vi "AlliGator Settings Storage.vi"(6 "Get(F)/Set":bool, 7 "AlliGator Settings List":T1=enum."Source Image:Use Image Histogram for Contrast", 8 "Error In":errorcluster, 11 "Variant Data in":variant) -> (0 "Error Out":errorcluster, 3 "Variant Data out":variant)   [LabVIEW 2021, in "AlliGator Settings.lvlib"]
doc: "Get/Set Settings parameter values using variant attributes."
uses:
  AlliGator Settings.lvlib
  Phasor/Phasor Explorer Gate Parameters.ctl
  Phasor/Phasor Gate Type.ctl
  Phasor/Phasor Type of User-defined Function.ctl
  Phasor/Phasor Explorer Decay Parameters.ctl
  Phasor/Phasor IRF Model.ctl
  Phasor/Phasor Explorer Phasor Parameters.ctl
  Phasor/Phasor Calculation Type.ctl
  Phasor/Phasor SEPL Type.ctl
  Phasor/Phasor Explorer Display Parameters.ctl
  Phasor/Phasor Type of Series.ctl
  Image/Image Save File Format.ctl
  AlliGator Phasor Plot Size.ctl
  AlliGator Gates to Skip.ctl
  Graphs/XY Graph/XY Graph Plot Shift Parameters.ctl
  Graphs/XY Graph/XY Graph Plot Shift Method.ctl
  Fits/IRF(X)PSED/IRF(X)PSED Extraction Options.ctl
  Fits/IRF(X)PSED/Fourier Series Smoothing Option.ctl
  Fits/IRF(X)PSED/Fourier Series Truncation.ctl
  Fits/IRF(X)PSED/IRF Extraction Method.ctl
  AlliGator Settings List.ctl
  AlliGator Low Count Pixels Rejection Options.ctl
  Phasor/Phasor Ratio Type.ctl
  AlliGator Baseline Subtraction Method.ctl
  Fits/IRF(X)PSED/Decay Fit Options v2.ctl
  Fits/Decay Convolution/Decay Model.ctl
  Fits/Residual Type.ctl
  Fits/IRF(X)PSED/Fit Weights Type.ctl
  Fits/Non-linear Fitting Method v2.ctl
  Fits/Fit Calculation Method.ctl
  Fits/Non-linear Fitting Algorithm.ctl
  Fits/IRF(X)PSED/Decay Fit Parameters & Derived Quantities List.ctl
  AlliGator Decay Fit Parameter Constraints 2.ctl
  Fits/IRF(X)PSED/Decay Fit Parameters In List.ctl
  AlliGator IRF Optimization Controls.ctl
  AlliGator IRF Deconvolution Metrics.ctl
  Math/Advanced Signal Processing Toolkit/Wavelet Analysis Options.ctl
  AlliGator High Count Pixels Rejection Options.ctl
  AlliGator Image Smoothing Options.ctl
  Arrays/Kernel Type.ctl
  Arrays/Smoothing Algorithm.ctl
  Fits/Square Pulse/Square Pulse Options.ctl
  Fits/Square Pulse/Square Pulse Levels Type.ctl
  AlliGator Image Binning Options.ctl
  AlliGator Phasor Plot Smoothing Options.ctl
  AlliGator Phasor Plot Graphics Options.ctl
  AlliGator Exported Image Settings.ctl
  AlliGator Define Gates to.ctl
  AlliGator Gates to Keep.ctl
  AlliGator Phasor Ratio Color-Coded Quantity.ctl
  Phasor/Phasor Calibration Type.ctl
  Histograms/Linear Histogram Options.ctl
  Histograms/Histogram Bin Option.ctl
  Histograms/Histogram Bin Position.ctl
  AlliGator Gate Arithmetic.ctl
  AlliGator Phasor Reference Associated with Shortest Lifetime.ctl
  AlliGator Python Settings.ctl
  SwissSPAD/SwissSPAD Live_Image Display Options.ctl
  AlliGator Average Lifetime Options.ctl
  AlliGator Calibration Map Algorithm.ctl
  AlliGator Guess Parameters Options.ctl
  Phasor/Phasor Standard Deviation Options.ctl
  AlliGator Source Image Scale Bar Options.ctl
  Fits/IRF(X)PSED/MLE Baseline Offset Type.ctl
  Image/Flatfield Correction Options.ctl
  Graphs/XY Graph/XY Plot Data.ctl
  Phasor/Phasor User-defined Gate & IRF.vi
  Notebook/Verbose Mode.vi
  Notebook/Notebook.lvlib
  Graphs/XY Graph/XY Graph Add-Ons.lvlib
  Phasor/Phasor.lvlib
  Utilities/Utilities.lvlib
  AlliGator Decay Analysis.lvlib
  AlliGator Phasor Plot.lvlib
  Image/Image.lvlib
  AlliGator Decay Preprocessing.lvlib
  Fits/Fits.lvlib
  AlliGator Decay Fit.lvlib
  AlliGator IRF.lvlib
  Math/Math.lvlib
  Arrays/Arrays.lvlib
  AlliGator Source Image.lvlib
  Phasor/Phasor Explorer.lvlib
  AlliGator Phasor Ratio.lvlib
  Histograms/Histogram Window.lvlib
  SwissSPAD/SwissSPAD Live.lvlib
  AlliGator Phasor Calibration.lvlib
panel:
  in  "Show Dead Left Columns Correction":bool
  in  "Tab Control":T2(tab)
  in  "Source ImageTab":T3(tab)
  in  "Use Image Histogram for Contrast":bool=TRUE
  in  "Low Count Pixels Rejection Options":T4={"Background Low Threshold Factor"=0.0, "Fixed Low Background Threshold"=20000.0, "Reject Low Count Pixels"=FALSE, "Low Percentile"=0.0} {"Low Percentile" min=0.0 max=100.0}
  in  "High Count Pixels Rejection Options":T5={"Background High Threshold Factor"=0.0, "Fixed High Background Threshold"=20000.0, "Reject High Count Pixels"=FALSE, "High Percentile"=100.0} {"High Percentile" min=0.0 max=100.0}
  in  "Hot Pixel Removal":T6 {"Percentile" min=0 max=100}
  in  "Dead Left Columns Correction":bool
  in  "Use Fixed ROI Diameter":bool
  in  "ROI Diameter":i32=12
  in  "ROI Center Color":u32(colorbox)=16711680
  in  "Image Binning Options":T7={"Use Image Binning"=FALSE, "X Bin"=1, "Y Bin"=1} {"Y Bin" min=1; "X Bin" min=1}
  in  "Flatfield Correction":T8={"Flatfield Estimation Options"={"Sampling Grid Size X"=256, "Sampling Grid Size Y"=256, "Polynomial Degree"=5}, "Background Options"={"Estimate Background"=TRUE, "Background Estimation Size"=32, "Niblack Deviation Factor [0. 1]"=0.2}, "Correction Factor"=1.1} {"Background Options"."Niblack Deviation Factor [0. 1]" min=0.0 max=1.0}
  in  "Image Smoothing Options":T9={"Use Image Smoothing"=FALSE, "Kernel Type"=enum."Bilinear", "Bin"=500, "Algorithm"=enum."Rapid"} {"Bin" min=1}
  in  "Peak Threshold":dbl=500.0
  in  "Intensity Threshold":dbl=500.0
  in  "Invert Binary Mask":bool
  in  "Image Pre-Processing Operations Order":string[](array[string]) caption="Order"
  in  "Median Overlay Color":u32(colorbox)
  in  "Overlay ROI Median":bool=TRUE caption="Use Image Brightness"
  in  "Image Resolution (Pixel Size)":dbl[unit]
  in  "Scale Bar Options":T12 caption="Scale Bar Options (*)"
  in  "Overlay Analyzed ROI Center":bool
  in  "Use Image Brightness":bool=TRUE
  in  "Blend Overlay with Image Background":bool=TRUE
  in  "Dataset Scaling Factor":dbl=1.0 caption="Scaling Factor" min=0.0
  in  "Gate Image Integration":dbl[unit]=3e-10 min=0.0 format="%#.3g"
  in  "Gate Image Exposure":dbl[unit]=3e-10 min=0.0 format="%#.3g"
  in  "Background File Subtraction":bool
  in  "Background Scaling Factor":dbl=1.0 caption="Scaling Factor"
  in  "Background File":path
  in  "Background Pile-up Correction":bool caption="Pile-up Correction"
  in  "Background Pixel Well Capacity":u32=1 caption="Max Value" min=1 step=1
  in  "Channel Arithmetic":T13
  in  "Available Gate Names":string[](array[string])
  in  "Channel Name":u16(ring) items=["Gate"]
  in  "Gates to Keep":T14 caption="Gates to Keep (*)"
  in  "Define Gates to":T15
  in  "Laser Period":dbl[unit] format="%#_3g"
  in  "Gates to Skip":T16
  in  "Gate Separation":dbl[unit]=4e-11
  in  "Gate Width":dbl[unit]=3e-10
  in  "Gate Step":i32=1 min=1
  in  "Pile-up Correction":bool
  in  "Pixel Well Capacity":i32=1 min=1
  in  "# Gates":u32=1 min=1 step=1
  in  "SYNC Period":dbl[unit] caption="IRF Period" min=0.0 format="%#_3g"
  in  "Mscrotime Gate Separation":dbl[unit]=1.0 min=0.0
  in  "Decay Tabs":T17(tab)
  in  "# Folds":u32=1 min=1
  in  "Fold Decay":bool caption="Straighten Decay"
  in  "Use Decay Pre-Processing":bool=TRUE
  in  "Head Fraction":dbl min=0.0 max=1.0
  in  "Use Cursors":bool
  in  "Use Periodicity":bool
  in  "Pixel-Normalize Decay":bool
  in  "Verbose Decay Pre-Processing":bool=TRUE caption="Verbose Devay Pre-Processing"
  in  "Straighten Decay":bool
  in  "Reverse Gates":bool caption="Revert Gates"
  in  "Additional Points":u32 caption="Gate Duration"
  in  "Tail Fraction":dbl caption="Gate Duration" min=0.0 max=1.0
  in  "Extrapolate Decay":bool
  in  "Baseline Subtraction Method":T18=enum."Min" caption="Method"
  in  "Background Definition Range":T19={"Min Gate"=0.0, "Max Gate"=8e-10}
  in  "Decay Shift Parameters":T20
  in  "Shift Decay":bool
  in  "Smoothen Decay":bool caption="Smooth Decay"
  in  "Smoothing Parameter":dbl caption="Gate Duration" min=0.0 max=1.0
  in  "1-Normalize Decay":bool
  in  "Background Subtraction":bool=TRUE
  in  "Constant Background":dbl=1.0
  in  "Decay Pre-Processing Operations Order":string[](array[string]) caption="Order"
  in  "[0-1]-Normalize Decay":bool caption="1- Normalize Decay"
  in  "Average Lifetime Options":T22={"Use Local IRF "=TRUE, "Use IRF Offset"=TRUE, "Use Fixed Offset"=TRUE, "Fixed Offset"=0.0, "Baseline %"=0.0} caption="Use Local IRF" {"Baseline %" min=0.0 max=100.0}
  in  "IRF Time Constants":dbl[](array[numeric])
  in  "IRF order":i32
  in  "Square Pulse Options":T23={"Method"=enum."Mode", "# Bins"=0, "Threshold %"=10.0, "Center on Midpoint"=FALSE, "Smoothen Plot"=FALSE} {"Threshold %" min=0.0 max=100.0}
  in  "Wavelet Analysis Options":T25={"Wavelet"=enum."db02", "Option for Approximate Coefficients"=enum."None", "# Levels"=1, "Threshold Settings"={"Thresholding Rule"=enum."Universal", "Rescaling Method"=enum."Single level", "Soft Threshold?"=TRUE}, "Wavelet Transform Type"=enum."Discrete"}
  in  "Time Constant for IRF Extraction":T26={"Time Constant for IRF Extraction"=1e-18, "IRF Order"=1, "Fourier Series Smoothing"=enum."None", "Noise Threshold"=0.0, "Smoothing Width"=0.0, "Fourier Series Truncation"=enum."Automatic", "Truncation Order"=0, "Save Power Spectrum"=FALSE, "Smoothing"=FALSE, "Smoothing Parameter"=0.0, "Smoothing Order"=1, "Method"=enum."Direct"} caption="Gate Duration" {"Smoothing Order" min=1 max=10; "Time Constant for IRF Extraction" format="%#_5g"}
  in  "Extract IRF instead of Decay":bool
  in  "IRF Optimization Options":T30={"Search Range"=1e-18, "Search Step"=1e-09, "Tail Threshold (%)"=1e-09, "Regularized IRF"=FALSE, "Export Plot"=FALSE, "Export Data"=FALSE, "Smooth Metrics"=FALSE, "S-G Side Points"=1, "S-G Polynomial Order"=3, "Metrics"=enum."Average"} {"S-G Polynomial Order" min=3 max=10; "S-G Side Points" min=1; "Search Range" min=0.0 max=1e-09}
  in  "Use Data Information Laser Period":bool
  in  "Use Legagy Fitting Approach":bool
  in  "Fit Options":T32={"Show Fit Residuals"=TRUE, "Fit Model"=enum."1-Exponential", "Residual Type"=enum."Standard", "Max Decay Percentile"=0.0, "Min Decay Percentile"=0.0, "Show Full Decay"=TRUE, "Weights"=enum."Unweighted", "Fitting Method"=enum."Least Square", "Compute Parameter Uncertainties"=TRUE, "Periodic Boundaries"=TRUE, "Model Calculation"=enum."Simulation", "Period"=1.2500000000000001e-08, "Termination Criteria"={"Max Iterations"=1000, "Max Function Calls"=0, "Max Time"=1000.0, "Function Tolerance"=1e-06, "Parameter Tolerance"=1e-06, "Gradient Tolerance"=0.0, "Min Lambda"=1e-06, "Max Lambda"=1e-06, "Initial Tick Count"=0}, "Offset Resolution"=1.2500000000000001e-08, "Use Local IRF"=TRUE, "Fitting Algorithm"=enum."Levenberg-Marquardt"} {"Offset Resolution" min=0.0; "Period" min=0.0; "Min Decay Percentile" min=0.0 max=1.0; "Max Decay Percentile" min=0.0 max=1.0}
  in  "MLE Baseline Offset Type":T39
  in  "MLE Baseline Offset":dbl
  in  "Guess Parameters Options":T40 caption="Options"
  in  "Guess Parameters Names":T41[](array[typedef])
  in  "Guess Parameter Values":dbl[](array[numeric]) caption="Guess Parameters"
  in  "Fit Parameter Constraints":T42[](array[typedef]) {"Max Value" format="%#.3g"; "Min Value" format="%#.3g"}
  in  "Displayed Fit Parameters":T43[](array[typedef])
  in  "Export Tabulated Results":bool=TRUE
  in  "Decay Graph Color Array":u32[](array[colorbox])
  in  "Show Last Decay only":bool
  in  "Max Peak Value":dbl
  in  "Reject High Decay Peak Pixels":bool
  in  "Min Peak Value":dbl
  in  "Reject Low Decay Peak Pixels":bool
  in  "Intensity Correction File":path
  in  "Use Intensity Correction File":bool
  in  "Use File Timestamp":bool
  in  "Time Step":dbl[unit]=1.0
  in  "User-defined Quantity":string
  in  "Blend Overlay with Phasor Background":bool=TRUE
  in  "Draw Reference Segment":bool
  in  "Store Phasor Harmonics":bool
  in  "All Phasor Plot ROIs":bool
  in  "Selected Phasor Plot ROI(s)":bool
  in  "Phasor Ratio Color-Coded Quantity":T44 caption="Displayed Quantity"
  in  "All Image ROIs":bool
  in  "Selected Image ROI(s)":bool
  in  "Reference Radius":i32=512
  in  "Phasor Ratio Display Range":cluster{dbl, dbl}(slide)={0.0, 454.0} scale=0.0..1.0
  in  "Phasor Plot Graphics Options":T45={"UC Color"=3381759, "Show UC Tau Ticks"=FALSE, "SEPL Color"=3381759, "Show SEPL Tau Ticks"=FALSE, "Axes Color"=16776960, "Show (g,s) Ticks"=FALSE, "Show UC"=FALSE, "Show SEPL"=FALSE, "Show Axes"=FALSE, "Show UC Tau Labels"=FALSE, "Show SEPL Tau Labels"=FALSE, "Show (g,s) Labels"=FALSE, "UC Label Size"=18, "UC Label Distance"=0.0, "SEPL Label Size"=18, "SEPL Label Distance"=0.0, "Axes Label Size"=18, "Axes Label Distance"=0.0}
  in  "Phasor Plot Smoothing Options":T46={"Use Phasor Plot Smoothing"=FALSE, "Kernel Type"=enum."Uniform", "Bin"=1, "Algorithm"=enum."Rapid"} {"Bin" min=1 step=2}
  in  "Phasor Ratio Color Map":string
  in  "Phasor Ratio Color Map Type":T47(radio)
  in  "Show Color Map Vertices":bool=TRUE
  in  "Exponential Fading":bool
  in  "Phasor Ratio Reference Colors":T48={"Reference 1"=3381759, "Reference 2"=3381759, "Boundary"=3381759}
  in  "Phasor Ratio Decay Range":dbl=1.0
  in  "Show References":bool
  in  "Save Phasor Plot":bool
  in  "Cumulative Phasor Plot":bool
  in  "Phasor Plot Size":T49={"H"=512, "V"=512, "Margin"=0.2} {"Margin" min=0.0}
  in  "Use Phasor Brightness":bool
  in  "Phasor SDV Options":T50={"Compute Estimated SDV"=FALSE, "# Replicas"=100, "Use Estimated Average Phasor"=FALSE}
  in  "Define Shortest Lifetime as":T51
  in  "Save Phasor Graph Image":bool
  in  "Pixel-level Phasor Computation":bool
  in  "Phasor Ratio Type":T52
  in  "Phasor Frequency":dbl[unit]=160000000.0
  in  "Phasor Graph Active":bool caption="Save Phasor Graph Image"
  in  "SEPL Tabs":enum32{"Display", "Phasor", "IRF", "Gates"}(tab)
  in  "SEPL Display Parameters":T53={"# Points"=1000, "Ramp Type"=enum."Logarithmic", "Type of Series"=enum."1-Exp Decays", "Min tau"=1.0000000000000002e-12, "Max tau"=1.0000000000000001e-07, "Include 0"=FALSE, "Include Infinity"=FALSE} {"Min tau" min=0.0; "Max tau" min=0.0; "# Points" min=1 step=1}
  in  "SEPL Phasor Parameters":T55={"Harmonic Frequency"=0.0, "Use f* = 1/D Frequency"=FALSE, "Calibrated Phasor"=FALSE, "Calibration Lifetime"=1e-09, "Phasor Calculation"=enum."Direct Sum", "SEPL Type"=enum."UC", "# Gates"=1.0, "Square Gate Width"=1e-09, "Show Ticks"=FALSE} {"Square Gate Width" min=0.0; "# Gates" min=0.0; "Calibration Lifetime" min=0.0; "Harmonic Frequency" min=0.0}
  in  "SEPL IRF Parameters":T58={"Lifetime"=3.0000000000000004e-09, "IRF Offset"=0.0, "IRF Period"=1.2500000000000001e-08, "Normalized Decays"=FALSE, "IRF Model"=enum."Dirac", "IRF Parameter 1"=0.0} {"Lifetime" min=0.0; "IRF Period" min=0.0}
  in  "SEPL Gate Parameters":T60={"First Gate Start"=0.0, "Use Gate Center"=FALSE, "Gate Width"=0.0, "Gate Step"=0.0, "# Gates"=1.0, "Gate Type"=enum."Square", "Edge Width"=0.0, "Top Slope"=0.0, "Reversed Sawtooth?"=FALSE, "Analytical Computation"=FALSE, "Integration"=enum."Item 0", "Tolerance"=1.0, "# Steps"=1.0, "Type of User-defined Function"=enum."Gate", "Use Gate Step"=FALSE} {"# Steps" min=0.0; "Tolerance" min=0.0; "Top Slope" min=0.0; "Edge Width" min=0.0; "Gate Step" min=0.0; "# Gates" min=1.0 step=1.0; "Gate Width" min=0.0}
  in  "Calibration Map Algorithm":T63
  in  "Calibration Type":T64=enum."Single Phasor"
  in  "Use Backup Calibration if needed":bool=TRUE
  in  "Backup Calibration Type":T65(ring) caption="Backup Calibration"
  in  "Calibration Lifetime":dbl[unit]=1e-09
  in  "Decay Analysis Parameters":T20
  in  "Python Settings":T66
  in  "Transparent Mask Color":u32(colorbox)
  in  "ROI Description Max Characters":i32=256
  in  "Beep on Error":bool caption="Verbose Error Mode"
  in  "# Logical Processors Used":i32 caption="Used" min=1 max=16
  in  "Histogram Options":T67={"Bin Size"=0.0, "Bin Number"=0, "Bin Option"=enum."Bin Number", "Min Value"=-inf, "Max Value"=inf, "Filter NaN & Infinite Values"=TRUE, "Frequency Plot"=FALSE, "Align Bins"=FALSE, "Bin Location"=enum."Left", "Project Outside Values"=FALSE, "Max Histogram Size"=100000} {"Max Histogram Size" format="%.0e"}
  in  "Exported Gate Image Settings":T70
  in  "Verbose Error Mode":bool
  in  "Verbose Settings Mode":bool
  in  "Beep after Script":bool
  in  "Verbose Mode":bool
  in  "Saved Displayed Image File Format":T71
  in  "Visible Settings Tab":string caption="Settings Tab List"
  in  "Include Loading in Timing":bool
  in  "Last Run Version":string
  # "see the AlliGator License on the block diagram (Ctrl+E or Window:Show Block Diagram)"
  # "Gates Characteristics"
  # "Limit Phasor Plot Analysis  to:"
  # "Lifetime Analysis Options"
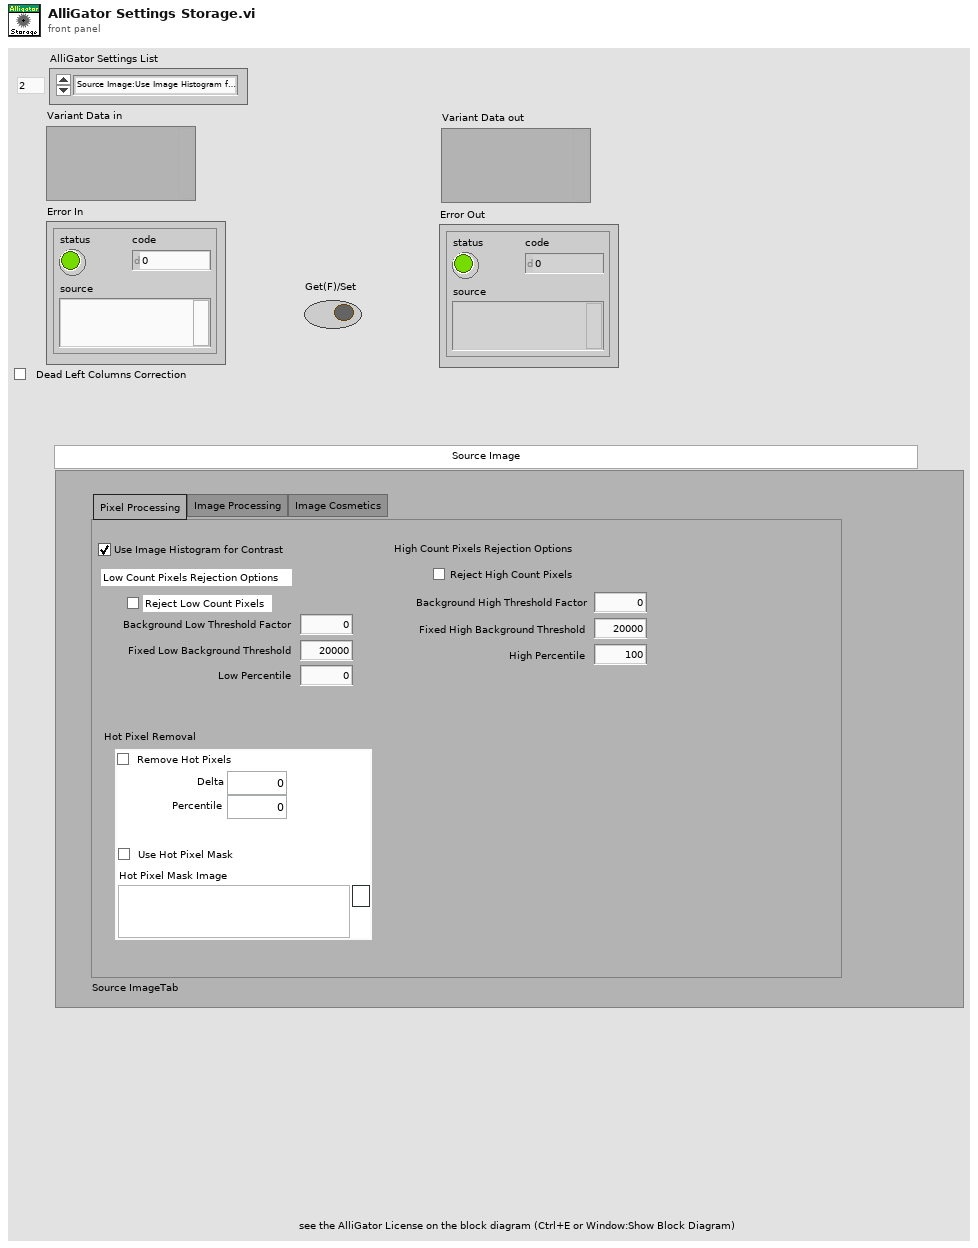
[diagram p1: front panel]
types:
  T1 = typedef "AlliGator Settings.lvlib/AlliGator Settings List.ctl" = enum16{"GUI:Visible Settings Tab", "GUI:Last Run Version", "Source Image:Use Image Histogram for Contrast", "Source Image:Low Count Pixels Rejection Options", "Source Image:High Count Pixels Rejection Options", "Source Image:Use Image Brightness", "Source Image:Blend Overlay with Image Background", "Source Image:Use Fixed ROI Diameter", "Source Image:ROI Diameter", "Source Image:ROI Center Color", "Source Image:Peak Threshold", "Source Image:Intensity Threshold", "Source Image:Image Binning Options", "Source Image:Image Smoothing Options", "Source Image:Image Histogram Active", "Source Image:Invert Binary Mask", "Source Image:Hot Pixel Removal", "Source Image:Overlay Analyzed ROI Center", "Source Image:Auto-Adjust Contrast", "Source Image:Histogram Lower Percentile", "Source Image:Histogram Upper Percentile", "Source Image:Save Source Image", "Source Image:Scale Bar Options", "Source Image:Image Resolution (Pixel Size)", "Source Image:Flatfield Correction", "Source Image:Show Dead Left Columns Correction", "Source Image:Dead Left Columns Correction", "Source Image:Image Pre-Processing Operations Order", "Source Image:Overlay ROI Median", "Source Image:Median Overlay Color", "Data Information:Gate Width", "Data Information:Nanotime Gate Separation", "Data Information:Macrotime Gate Separation", "Data Information:Gate Step", "Data Information:# Gates", "Data Information:Gate Image Exposure", "Data Information:Gate Image Integration", "Data Information:Gates to Skip", "Data Information:Gates to Keep", "Data Information:Define Gates to", "Data Information:Channel Name", "Data Information:Available Channel Names", "Data Information:Channel Arithmetic", "Data Information:Background File Subtraction", "Data Information:Background File", "Data Information:Background Scaling Factor", "Data Information:Background Pile-up Correction", "Data Information:Background Pixel Well Capacity", "Data Information:Laser Period", "Data Information:SYNC Period", "Data Information:Pile-up Correction", "Data Information:Pixel Well Capacity", "Data Information:Dataset Scaling Factor", "Fluorescence Decay_Decay Pre-Processing:Reverse Gates", "Fluorescence Decay_Decay Pre-Processing:Verbose Decay Pre-Processing", "Fluorescence Decay_Decay Pre-Processing:Use Decay Pre-Processing", "Fluorescence Decay_Decay Pre-Processing:Background Subtraction", "Fluorescence Decay_Decay Pre-Processing:Background Definition Range", "Fluorescence Decay_Decay Pre-Processing:Baseline Subtraction Method", "Fluorescence Decay_Decay Pre-Processing:Decay Pre-Processing Operations Order", "Fluorescence Decay_Decay Pre-Processing:Smoothing Parameter", "Fluorescence Decay_Decay Pre-Processing:Shift Decay", "Fluorescence Decay_Decay Pre-Processing:Decay Shift Parameters", "Fluorescence Decay_Decay Pre-Processing:Fold Decay", "Fluorescence Decay_Decay Pre-Processing:# Folds", "Fluorescence Decay_Decay Pre-Processing:1-Normalize Decay", "Fluorescence Decay_Decay Pre-Processing:[0-1]-Normalize Decay", "Fluorescence Decay_Decay Pre-Processing:Smoothen Decay", "Fluorescence Decay_Decay Pre-Processing:Extrapolate Decay", "Fluorescence Decay_Decay Pre-Processing:Use Periodicity", "Fluorescence Decay_Decay Pre-Processing:Use Cursors", "Fluorescence Decay_Decay Pre-Processing:Tail Fraction", "Fluorescence Decay_Decay Pre-Processing:Head Fraction", "Fluorescence Decay_Decay Pre-Processing:Additional Points", "Fluorescence Decay_Decay Pre-Processing:Straighten Decay", "Fluorescence Decay_Decay Pre-Processing:Constant Background", "Fluorescence Decay_Decay Pre-Processing:Pixel-Normalize Decay", "Fluorescence Decay_Advanced Analysis:Extract IRF instead of Decay", "Fluorescence Decay_Advanced Analysis:IRF Extraction Options", "Fluorescence Decay_Advanced Analysis:IRF Optimization Options", "Fluorescence Decay_Advanced Analysis:Square Pulse Options", "Fluorescence Decay_Advanced Analysis:IRF Order", "Fluorescence Decay_Advanced Analysis:IRF Time Constants", "Fluorescence Decay_Advanced Analysis:Wavelet Analysis Options", "Fluorescence Decay_Advanced Analysis:Average Lifetime Options", "Fluorescence Decay_Fit Options:Fit Options", "Fluorescence Decay_Fit Options:Use Legacy Fitting Approach", "Fluorescence Decay_Fit Options:Use Data Information Laser Period", "Fluorescence Decay_Fit Parameters:Displayed Fit Parameters", "Fluorescence Decay_Fit Parameters:Fit Parameter Constraints", "Fluorescence Decay_Fit Parameters:Export Tabulated Results", "Fluorescence Decay_Fit Parameters:MLE Baseline Offset Type", "Fluorescence Decay_Fit Parameters:MLE Baseline Offset", "Fluorescence Decay_Fit Parameters:Guess Parameter Names", "Fluorescence Decay_Fit Parameters:Guess Parameter Values", "Fluorescence Decay_Fit Parameters:Guess Parameters Options", "Fluorescence Decay_Styles:Show Last Decay Only", "Fluorescence Decay_Styles:Decay Graph Color Array", "Fluorescence Decay:Decay Graph Active", "Fluorescence Decay Statistics:Min Peak Value", "Fluorescence Decay Statistics:Reject Low Decay Peak Pixels", "Fluorescence Decay Statistics:Reject High Decay Peak Pixels", "Fluorescence Decay Statistics:Max Peak Value", "Time Traces:Use File Timestamp", "Time Traces:Time Step", "Time Traces:Use Intensity Correction File", "Time Traces:Intensity Correction File", "Phasor Plot:Phasor Plot Smoothing Options", "Phasor Plot:Phasor Plot Size", "Phasor Plot:Phasor Plot Graphics Options", "Phasor Plot:Cumulative Phasor Plot", "Phasor Plot:Use Phasor Brightness", "Phasor Plot:Blend Overlay with Phasor Background", "Phasor Plot:Save Phasor Plot", "Phasor Plot:Show References", "Phasor Plot:Phasor Ratio Decay Range", "Phasor Plot:Exponential Fading", "Phasor Plot:Phasor Ratio Reference Colors", "Phasor Plot:Reference Radius", "Phasor Plot:Show Color Map Vertices", "Phasor Plot:Phasor Plot Active", "Phasor Plot:Phasor Ratio Color Map Type", "Phasor Plot:Phasor Ratio Color Map", "Phasor Plot:Phasor Ratio Display Range", "Phasor Plot:Selected Image ROI(s)", "Phasor Plot:All Image ROIs", "Phasor Plot:Selected Phasor Plot ROI(s)", "Phasor Plot:All Phasor Plot ROIs", "Phasor Plot:Phasor Ratio Color-Coded Quantity", "Phasor Plot:Store Phasor Harmonics", "Phasor Plot:Draw Reference Segment", "Phasor Plot:User-Defined Quantity", "Phasor Graph:Phasor Frequency", "Phasor Graph:Phasor Ratio Type", "Phasor Graph:Pixel-level Phasor Computation", "Phasor Graph:Save Phasor Graph", "Phasor Graph:Phasor Graph Active", "Phasor Graph:Phasor SDV Options", "Phasor Calibration:Use Backup Calibration if needed", "Phasor Graph:Define Shortest Lifetime as", "Phasor Calibration:Backup Calibration Type", "Phasor Calibration:Calibration Type", "Phasor Calibration:Calibration Lifetime", "Phasor Calibration:Calibration Map Algorithm", "Single-Exponential Phasor Locus (SEPL):Gate Parameters", "Single-Exponential Phasor Locus (SEPL):User-defined Gate", "Single-Exponential Phasor Locus (SEPL):User-defined IRF", "Single-Exponential Phasor Locus (SEPL):Phasor Parameters", "Single-Exponential Phasor Locus (SEPL):Decay & IRF Parameters", "Single-Exponential Phasor Locus (SEPL):Display Parameters", "Lifetime Analysis:Decay Analysis Parameters", "Lifetime Analysis:Lifetime Map Active", "Plugins:Python Settings", "Miscellaneous:Verbose Mode", "Miscellaneous:Beep after Script", "Miscellaneous:Saved Image File Format", "Miscellaneous:Exported Gate Image Settings", "Miscellaneous:Include Loading in Timing", "Miscellaneous:Verbose Settings Mode", "Miscellaneous:Histogram Options", "Miscellaneous:Beep on Error", "Miscellaneous:# Logical Processors Used", "Miscellaneous:ROI Description Max Characters", "Miscellaneous:Verbose Error Mode", "Miscellaneous:Transparent Mask Color"}
  T2 = enum32{"Source Image", "Data Information", "Fluorescence Decay", "Fluorescence Decay Statistics", "Time Traces", "Phasor Plot", "Phasor Graph", "Single-Exponential Phasor Locus (SEPL)", "Phasor Calibration", "Lifetime Analysis", "Plugins", "Miscellaneous"}
  T3 = enum32{"Pixel Processing", "Image Processing", "Image Cosmetics"}
  T4 = typedef "AlliGator Settings.lvlib/AlliGator Low Count Pixels Rejection Options.ctl" = cluster{"Background Low Threshold Factor":dbl, "Fixed Low Background Threshold":dbl, "Reject Low Count Pixels":bool, "Low Percentile":dbl}
  T5 = typedef "AlliGator Settings.lvlib/AlliGator High Count Pixels Rejection Options.ctl" = cluster{"Background High Threshold Factor":dbl, "Fixed High Background Threshold":dbl, "Reject High Count Pixels":bool, "High Percentile":dbl}
  T6 = typedef "SwissSPAD Live.lvlib/SwissSPAD Live_Image Display Options.ctl" = cluster{"Remove Screamers":bool, "Delta":sgl, "Equalize Histogram":bool, "Percentile":sgl, "Hot Pixel Mask Image":path, "Use Hot Pixel Mask":bool}
  T7 = typedef "AlliGator Source Image.lvlib/AlliGator Image Binning Options.ctl" = cluster{"Use Image Binning":bool, "X Bin":i32, "Y Bin":i32}
  T8 = typedef "Image.lvlib/Flatfield Correction Options.ctl" = cluster{"Flatfield Estimation Options":cluster{"Sampling Grid Size X":i32, "Sampling Grid Size Y":i32, "Polynomial Degree":i32}, "Background Options":cluster{"Estimate Background":bool, "Background Estimation Size":i32, "Niblack Deviation Factor [0. 1]":dbl}, "Correction Factor":sgl}
  T9 = typedef "AlliGator Settings.lvlib/AlliGator Image Smoothing Options.ctl" = cluster{"Use Image Smoothing":bool, "Kernel Type":T10, "Bin":i32, "Algorithm":T11}
  T10 = typedef "Arrays.lvlib/Kernel Type.ctl" = enum16{"Uniform", "Bilinear", "Gaussian"}
  T11 = typedef "Arrays.lvlib/Smoothing Algorithm.ctl" = enum16{"Rapid", "Thorough"}
  T12 = typedef "AlliGator Source Image.lvlib/AlliGator Source Image Scale Bar Options.ctl" = cluster{"Show Scale Bar Overlay":bool, "Scale Bar Length":dbl[unit], "Scale Bar Color":u32, "Scale Bar X":u32, "Scale Bar Y":u32, "Scale Bar Height":dbl[unit]}
  T13 = typedef "AlliGator Settings.lvlib/AlliGator Gate Arithmetic.ctl" = enum16{"None", "INT-G2", "G2/INT*<INT>", "(1 - G2/INT)*<INT>"}
  T14 = typedef "AlliGator Settings.lvlib/AlliGator Gates to Keep.ctl" = cluster{"First":u32, "Last":u32}
  T15 = typedef "AlliGator Settings.lvlib/AlliGator Define Gates to.ctl" = enum32{"Skip", "Keep"}
  T16 = typedef "AlliGator Decay Analysis.lvlib/AlliGator Gates to Skip.ctl" = cluster{"Start":u32, "End":u32}
  T17 = enum32{"Decay Pre-Processing", "Advanced Analysis", "Fit Options", "Fit Parameters", "Styles"}
  T18 = typedef "AlliGator Decay Analysis.lvlib/AlliGator Decay Preprocessing.lvlib/AlliGator Baseline Subtraction Method.ctl" = enum16{"Mean", "Min", "Square Gated Single-Exponential", "File", "Constant"}
  T19 = cluster{"Min Gate":dbl[unit], "Max Gate":dbl[unit]}
  T20 = typedef "XY Graph Add-Ons.lvlib/XY Graph Plot Shift Parameters.ctl" = cluster{"Type":T21, "Shift":dbl[unit], "Threshold":dbl, "Rotate":bool}
  T21 = typedef "XY Graph Add-Ons.lvlib/XY Graph Plot Shift Method.ctl" = enum16{"Default", "CFD", "Threshold", "Cross-Correlation"}
  T22 = typedef "AlliGator Settings.lvlib/AlliGator Average Lifetime Options.ctl" = cluster{"Use Local IRF ":bool, "Use IRF Offset":bool, "Use Fixed Offset":bool, "Fixed Offset":dbl[unit], "Baseline %":dbl}
  T23 = typedef "Fits.lvlib/Square Pulse Options.ctl" = cluster{"Method":T24, "# Bins":i32, "Threshold %":dbl, "Center on Midpoint":bool, "Smoothen Plot":bool}
  T24 = typedef "Fits.lvlib/Square Pulse Levels Type.ctl" = enum16{"Mode", "Mean"}
  T25 = typedef "Math.lvlib/Wavelet Analysis Options.ctl" = cluster{"Wavelet":enum16{"db02", "db03", "db04", "db05", "db06", "db07", "db08", "db09", "db10", "db11", "db12", "db13", "db14", "Haar", "bior1_3", "bior1_5", "bior2_2", "bior2_4", "bior2_6", "bior2_8", "bior3_1", "bior3_3", "bior3_5", "bior3_7", "bior3_9", "bior4_4 (FBI)", "bior5_5", "bior6_8", "coif1", "coif2", "coif3", "coif4", "coif5", "sym2", "sym3", "sym4", "sym5", "sym6", "sym7", "sym8"}, "Option for Approximate Coefficients":enum16{"None", "Threshold", "Detrend"}, "# Levels":i32, "Threshold Settings":cluster{"Thresholding Rule":enum16{"SURE", "Hybrid", "Universal", "Minimax"}, "Rescaling Method":enum16{"One", "Single level", "Multiple levels"}, "Soft Threshold?":bool}, "Wavelet Transform Type":enum16{"Discrete", "Undecimated"}}
  T26 = typedef "Fits.lvlib/IRF(X)PSED Extraction Options.ctl" = cluster{"Time Constant for IRF Extraction":dbl[unit], "IRF Order":i32, "Fourier Series Smoothing":T27, "Noise Threshold":dbl, "Smoothing Width":dbl, "Fourier Series Truncation":T28, "Truncation Order":i32, "Save Power Spectrum":bool, "Smoothing":bool, "Smoothing Parameter":dbl, "Smoothing Order":u32, "Method":T29}
  T27 = typedef "Fits.lvlib/Fourier Series Smoothing Option.ctl" = enum16{"None", "Lanczos Factors", "Fejer Summation"}
  T28 = typedef "Fits.lvlib/Fourier Series Truncation.ctl" = enum16{"Automatic", "Fixed"}
  T29 = typedef "Fits.lvlib/IRF Extraction Method.ctl" = enum16{"Direct", "Topless", "Toeplitz"}
  T30 = typedef "AlliGator Decay Analysis.lvlib/AlliGator IRF.lvlib/AlliGator IRF Optimization Controls.ctl" = cluster{"Search Range":dbl[unit], "Search Step":dbl[unit], "Tail Threshold (%)":dbl, "Regularized IRF":bool, "Export Plot":bool, "Export Data":bool, "Smooth Metrics":bool, "S-G Side Points":i32, "S-G Polynomial Order":i32, "Metrics":T31}
  T31 = typedef "AlliGator Decay Analysis.lvlib/AlliGator IRF.lvlib/AlliGator IRF Deconvolution Metrics.ctl" = enum16{"Average", "SDV", "Max", "Average * SDV", "Slope"}
  T32 = typedef "Fits.lvlib/Decay Fit Options v2.ctl" = cluster{"Show Fit Residuals":bool, "Fit Model":T33, "Residual Type":T34, "Max Decay Percentile":dbl, "Min Decay Percentile":dbl, "Show Full Decay":bool, "Weights":T35, "Fitting Method":T36, "Compute Parameter Uncertainties":bool, "Periodic Boundaries":bool, "Model Calculation":T37, "Period":dbl[unit], "Termination Criteria":cluster{"Max Iterations":i32, "Max Function Calls":i32, "Max Time":dbl[unit], "Function Tolerance":dbl, "Parameter Tolerance":dbl, "Gradient Tolerance":dbl, "Min Lambda":dbl, "Max Lambda":dbl, "Initial Tick Count":u32}, "Offset Resolution":dbl[unit], "Use Local IRF":bool, "Fitting Algorithm":T38}
  T33 = typedef "Fits.lvlib/Decay Model.ctl" = enum16{"1-Exponential", "2-Exponentials"}
  T34 = typedef "Fits.lvlib/Residual Type.ctl" = enum16{"Standard", "Normalized", "Reduced"}
  T35 = typedef "Fits.lvlib/Fit Weights Type.ctl" = enum16{"Unweighted", "1/Variance", "Best of All"}
  T36 = typedef "Fits.lvlib/Non-linear Fitting Method v2.ctl" = enum16{"Least Square", "Least Absolute Residual", "Bisquare", "MLE", "-", "Best of All"}
  T37 = typedef "Fits.lvlib/Fit Calculation Method.ctl" = enum16{"Simulation", "Convolution", "Integration"}
  T38 = typedef "Fits.lvlib/Non-linear Fitting Algorithm.ctl" = enum16{"Levenberg-Marquardt", "Trust-Region Dogleg"}
  T39 = typedef "Fits.lvlib/MLE Baseline Offset Type.ctl" = enum32{"Absolute", "Percentage"}
  T40 = typedef "AlliGator Decay Analysis.lvlib/AlliGator Decay Fit.lvlib/AlliGator Guess Parameters Options.ctl" = enum16{"Numerically estimated", "User-provided", "User-provided (normalized)", "Last valid fitted parameters"}
  T41 = typedef "Fits.lvlib/Decay Fit Parameters In List.ctl" = enum16{"Offset", "Baseline", "A_1", "tau_1", "A_2", "tau_2"}
  T42 = typedef "AlliGator Decay Analysis.lvlib/AlliGator Decay Fit.lvlib/AlliGator Decay Fit Parameter Constraints 2.ctl" = cluster{"Fit Parameter":T41, "Min Value":dbl, "Max Value":dbl, "Global":bool, "Used":bool}
  T43 = typedef "Fits.lvlib/Decay Fit Parameters & Derived Quantities List.ctl" = enum16{"Offset", "Baseline", "A_1", "tau_1", "A_2", "tau_2", "<tau>_a", "f1_a", "f2_a", "<tau>_i", "f1_i", "f2_i", "-", "R^2", "Chi^2"}
  T44 = typedef "AlliGator Phasor Ratio.lvlib/AlliGator Phasor Ratio Color-Coded Quantity.ctl" = enum16{"Phasor Ratio (f1 or a1)", "Average Lifetime (<tau>_i or <tau>_a))", "User-Defined Quantity"}
  T45 = typedef "AlliGator Settings.lvlib/AlliGator Phasor Plot Graphics Options.ctl" = cluster{"UC Color":u32, "Show UC Tau Ticks":bool, "SEPL Color":u32, "Show SEPL Tau Ticks":bool, "Axes Color":u32, "Show (g,s) Ticks":bool, "Show UC":bool, "Show SEPL":bool, "Show Axes":bool, "Show UC Tau Labels":bool, "Show SEPL Tau Labels":bool, "Show (g,s) Labels":bool, "UC Label Size":i16, "UC Label Distance":dbl, "SEPL Label Size":i16, "SEPL Label Distance":dbl, "Axes Label Size":i16, "Axes Label Distance":dbl}
  T46 = typedef "AlliGator Phasor Plot.lvlib/AlliGator Phasor Plot Smoothing Options.ctl" = cluster{"Use Phasor Plot Smoothing":bool, "Kernel Type":T10, "Bin":i32, "Algorithm":T11}
  T47 = enum32{"Interpolate Reference Colors", "Use Custom Map"}
  T48 = cluster{"Reference 1":u32, "Reference 2":u32, "Boundary":u32}
  T49 = typedef "AlliGator Phasor Plot.lvlib/AlliGator Phasor Plot Size.ctl" = cluster{"H":i32, "V":i32, "Margin":dbl}
  T50 = typedef "Phasor.lvlib/Phasor Standard Deviation Options.ctl" = cluster{"Compute Estimated SDV":bool, "# Replicas":u32, "Use Estimated Average Phasor":bool}
  T51 = typedef "AlliGator Phasor Ratio.lvlib/AlliGator Phasor Reference Associated with Shortest Lifetime.ctl" = enum32{"Reference 1", "Reference 2"}
  T52 = typedef "Phasor.lvlib/Phasor Ratio Type.ctl" = enum32{"Intensity-weighted", "Amplitude-weighted"}
  T53 = typedef "Phasor Explorer.lvlib/Phasor Explorer Display Parameters.ctl" = cluster{"# Points":i32, "Ramp Type":enum16{"Linear", "Logarithmic"}, "Type of Series":T54, "Min tau":dbl[unit], "Max tau":dbl[unit], "Include 0":bool, "Include Infinity":bool}
  T54 = typedef "Phasor.lvlib/Phasor Type of Series.ctl" = enum16{"1-Exp Decays", "Linear Combination of 1-Exp"}
  T55 = typedef "Phasor Explorer.lvlib/Phasor Explorer Phasor Parameters.ctl" = cluster{"Harmonic Frequency":dbl[unit], "Use f* = 1/D Frequency":bool, "Calibrated Phasor":bool, "Calibration Lifetime":dbl[unit], "Phasor Calculation":T56, "SEPL Type":T57, "# Gates":dbl, "Square Gate Width":dbl[unit], "Show Ticks":bool}
  T56 = typedef "Phasor.lvlib/Phasor Calculation Type.ctl" = enum16{"Direct Sum", "Analytical Formula"}
  T57 = typedef "Phasor.lvlib/Phasor SEPL Type.ctl" = enum16{"UC", "L_N", "L_N[W]", "L_X"}
  T58 = typedef "Phasor Explorer.lvlib/Phasor Explorer Decay Parameters.ctl" = cluster{"Lifetime":dbl[unit], "IRF Offset":dbl[unit], "IRF Period":dbl[unit], "Normalized Decays":bool, "IRF Model":T59, "IRF Parameter 1":dbl[unit]}
  T59 = typedef "Phasor.lvlib/Phasor IRF Model.ctl" = enum16{"Dirac", "Exponential"}
  T60 = typedef "Phasor Explorer.lvlib/Phasor Explorer Gate Parameters.ctl" = cluster{"First Gate Start":dbl[unit], "Use Gate Center":bool, "Gate Width":dbl[unit], "Gate Step":dbl[unit], "# Gates":dbl, "Gate Type":T61, "Edge Width":dbl[unit], "Top Slope":dbl[unit], "Reversed Sawtooth?":bool, "Analytical Computation":bool, "Integration":enum32{"Item 0", "Item 1"}, "Tolerance":dbl, "# Steps":dbl, "Type of User-defined Function":T62, "Use Gate Step":bool}
  T61 = typedef "Phasor.lvlib/Phasor Gate Type.ctl" = enum16{"Square", "Finite Edge Square", "Finite Edge, Tilted Top Square", "Triangle", "Sawtooth", "User-defined"}
  T62 = typedef "Phasor.lvlib/Phasor Type of User-defined Function.ctl" = enum16{"Gate", "IRF"}
  T63 = typedef "AlliGator Phasor Calibration.lvlib/AlliGator Calibration Map Algorithm.ctl" = enum16{"Simple Search", "Min Distance"}
  T64 = typedef "Phasor.lvlib/Phasor Calibration Type.ctl" = enum16{"None", "Single Phasor", "Phasor Series", "Phasor Map"}
  T65 = enum16{"Single Calibration", "Nearest Valid Calibration"}
  T66 = typedef "AlliGator Settings.lvlib/AlliGator Python Settings.ctl" = cluster{"Python Version":string, "Use PATH definition":bool, "Python.exe Path":path, "Include Example Plugins":bool}
  T67 = typedef "Histogram Window.lvlib/Linear Histogram Options.ctl" = cluster{"Bin Size":dbl, "Bin Number":i32, "Bin Option":T68, "Min Value":dbl, "Max Value":dbl, "Filter NaN & Infinite Values":bool, "Frequency Plot":bool, "Align Bins":bool, "Bin Location":T69, "Project Outside Values":bool, "Max Histogram Size":i32}
  T68 = typedef "Histogram Window.lvlib/Histogram Bin Option.ctl" = enum32{"Bin Number", "Bin Size"}
  T69 = typedef "Histogram Window.lvlib/Histogram Bin Position.ctl" = enum16{"Left", "Center", "Right"}
  T70 = typedef "AlliGator Settings.lvlib/AlliGator Exported Image Settings.ctl" = cluster{"bitness":bool, " Min Value":sgl, " Max Value":sgl}
  T71 = typedef "Image.lvlib/Image Save File Format.ctl" = enum16{"PNG", "JPEG", "BMP"}
  T72 = typedef "XY Graph Add-Ons.lvlib/XY Plot Data.ctl" = cluster{"X Array":dbl[], "Y Array":dbl[]}
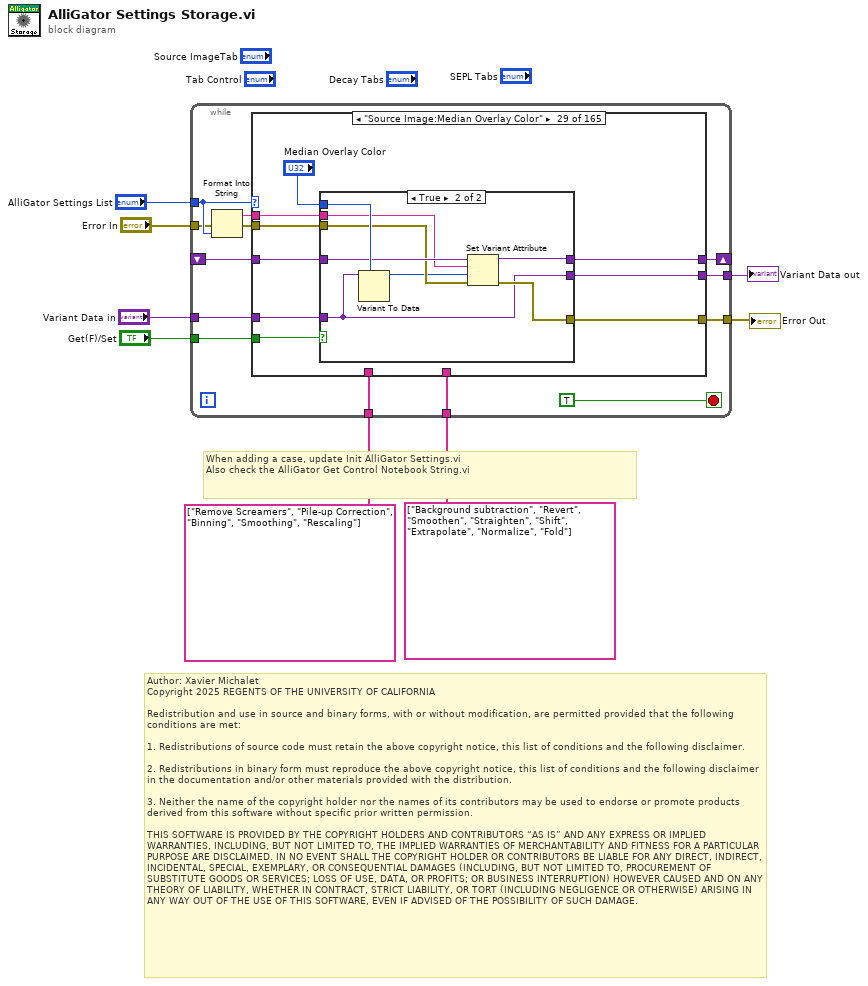
[diagram p0: block diagram]
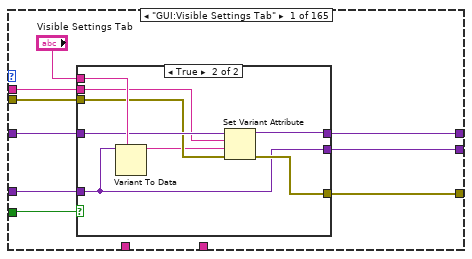
[diagram p2: hidden frame]
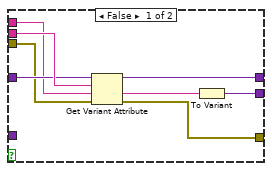
[diagram p3: hidden frame]
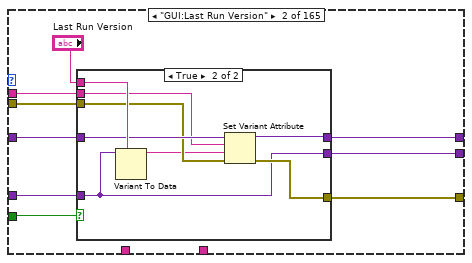
[diagram p4: hidden frame]
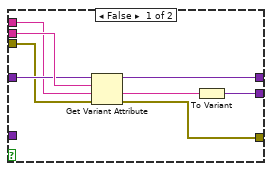
[diagram p5: hidden frame]
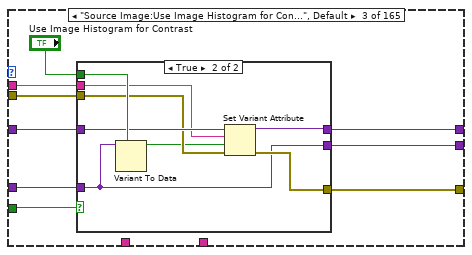
[diagram p6: hidden frame]
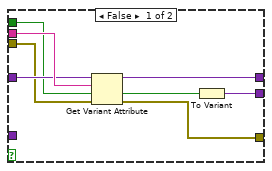
[diagram p7: hidden frame]
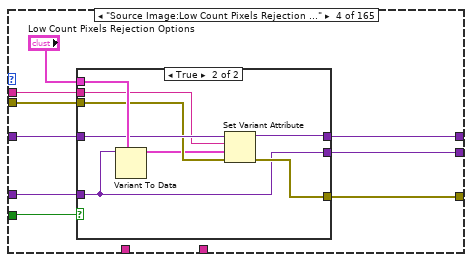
[diagram p8: hidden frame]
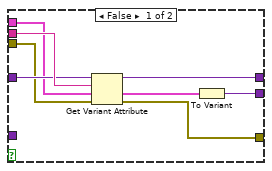
[diagram p9: hidden frame]
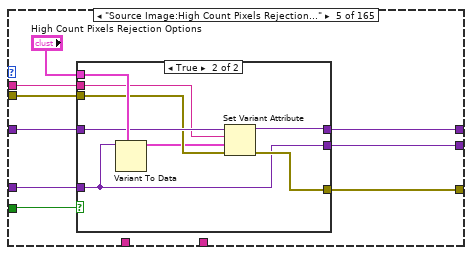
[diagram p10: hidden frame]
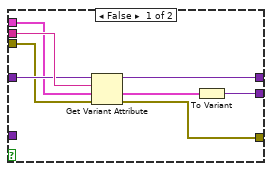
[diagram p11: hidden frame]
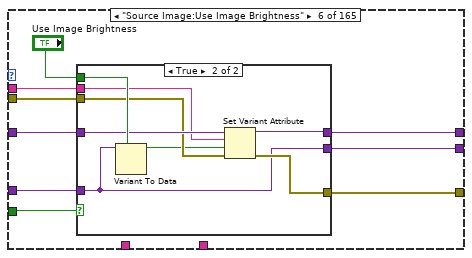
[diagram p12: hidden frame]
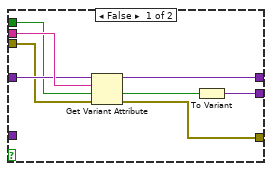
[diagram p13: hidden frame]
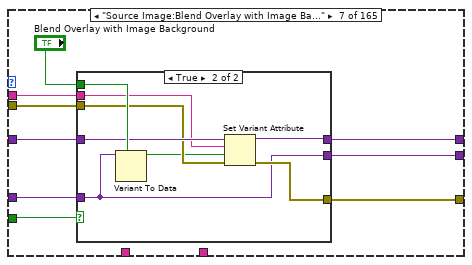
[diagram p14: hidden frame]
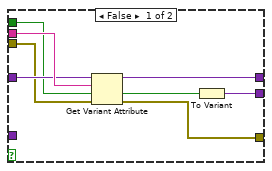
[diagram p15: hidden frame]
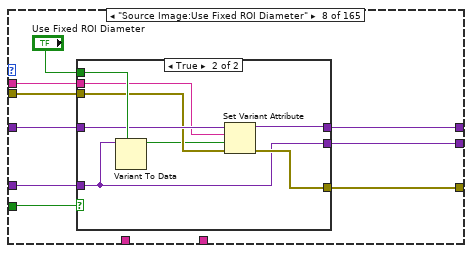
[diagram p16: hidden frame]
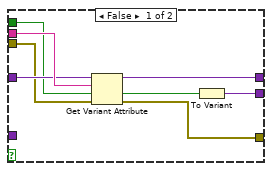
[diagram p17: hidden frame]
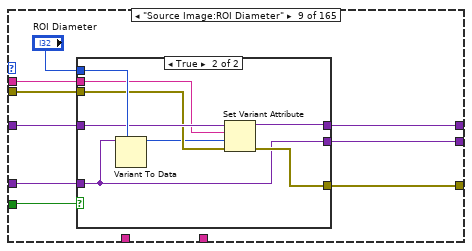
[diagram p18: hidden frame]
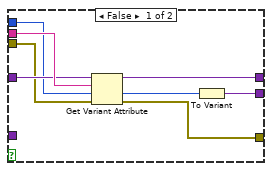
[diagram p19: hidden frame]
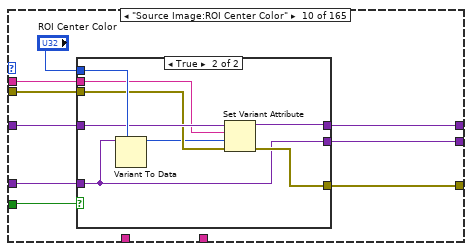
[diagram p20: hidden frame]
diagram:
  # "Author: Xavier Michalet\nCopyright 2025 REGENTS OF THE UNIVERSITY OF CALIFORNIA\n\nRedistribution and use in source and binary forms, with or without modification, are permitted provided that the following conditions are met:\n\n1. Redistributions of source code must retain the above copyright notice, this list of conditions and the following disclaimer.\n\n2. Redistributions in binary form must reproduce the above copyright notice, this list of conditions and the following disclaimer in the documentation and/or other materials provided with the distribution.\n\n3. Neither the name of the copyright holder nor the names of its contributors may be used to endorse or promote products derived from this software without specific prior written permission.\n\nTHIS SOFTWARE IS PROVIDED BY THE COPYRIGHT HOLDERS AND CONTRIBUTORS “AS IS” AND ANY EXPRESS OR IMPLIED WARRANTIES, INCLUDING, BUT NOT LIMITED TO, THE IMPLIED WARRANTIES OF MERCHANTABILITY AND FITNESS FOR A PARTICULAR PURPOSE ARE DISCLAIMED. IN NO EVENT SHALL THE COPYRIGHT HOLDER OR CONTRIBUTORS BE LIABLE FOR ANY DIRECT, INDIRECT, INCIDENTAL, SPECIAL, EXEMPLARY, OR CONSEQUENTIAL DAMAGES (INCLUDING, BUT NOT LIMITED TO, PROCUREMENT OF SUBSTITUTE GOODS OR SERVICES; LOSS OF USE, DATA, OR PROFITS; OR BUSINESS INTERRUPTION) HOWEVER CAUSED AND ON ANY THEORY OF LIABILITY, WHETHER IN CONTRACT, STRICT LIABILITY, OR TORT (INCLUDING NEGLIGENCE OR OTHERWISE) ARISING IN ANY WAY OUT OF THE USE OF THIS SOFTWARE, EVEN IF ADVISED OF THE POSSIBILITY OF SUCH DAMAGE."
  # "When adding a case, update Init AlliGator Settings.vi\nAlso check the AlliGator Get Control Notebook String.vi"
  n1 = while {
    tunnel: "AlliGator Settings List" -> [w21]
    tunnel: "Get(F)/Set" -> [w18]
    tunnel: "Variant Data in" -> [w17]
    tunnel: "Error In" -> [w16]
    shift-right: [w13] -> _
    shift-left: _ -> [w14]
    tunnel: [w12] -> w4
    tunnel: [w11] -> w3
    tunnel: string[] ["Background subtraction", "Revert", "Smoothen", "Straighten", "Shift", "Extrapolate", "Normalize", "Fold"] ("Operation Order") -> [w10]
    tunnel: string[] ["Remove Screamers", "Pile-up Correction", "Binning", "Smoothing", "Rescaling"] ("Operation Order") -> [w9]
    stop <- TRUE stop-if-true
    n2 = Format Into String(error in=w16, w21) -> (resulting string=w20:string, error out=w15:errorcluster)  [unwired: 2 in]
    n3 = case shown="\"Source Image:Median Overlay Color\"" w21 {
      tunnel: w20 -> [w29 w54 w79 w104 w129 w154 w179 w204 w229 w254 w279 w304 w329 w354 w379 w404 w429 w454 w479 w504 w529 w554 w579 w604 w629 w654 w679 w704 w729 w754 w779 w804 w829 w854 w879 w904 w929 w954 w979 w1004 w1029 w1054 w1079 w1104 w1129 w1154 w1179 w1204 w1229 w1254 w1279 w1304 w1329 w1354 w1379 w1404 w1429 w1454 w1480 w1511 w1541 w1566 w1591 w1616 w1641 w1666 w1691 w1716 w1741 w1766 w1791 w1816 w1841 w1866 w1891 w1916 w1941 w1966 w1991 w2016 w2041 w2066 w2091 w2118 w2143 w2168 w2193 w2218 w2243 w2268 w2293 w2318 w2343 w2368 w2393 w2418 w2443 w2468 w2493 w2518 w2543 w2568 w2593 w2618 w2643 w2668 w2693 w2718 w2743 w2768 w2793 w2818 w2843 w2868 w2893 w2918 w2943 w2968 w2993 w3018 w3043 w3068 w3093 w3121 w3146 w3171 w3196 w3221 w3246 w3271 w3296 w3321 w3346 w3371 w3396 w3421 w3446 w3471 w3496 w3521 w3546 w3571 w3596 w3621 w3646 w3671 w3696 w3721 w3746 w3771 w3796 w3821 w3846 w3871 w3896 w3921 w3946 w3971 w3996 w4021 w4046 w4071 w4097 w4122 w4147]
      tunnel: w18 -> [w30 w55 w80 w105 w130 w155 w180 w205 w230 w255 w280 w305 w330 w355 w380 w405 w430 w455 w480 w505 w530 w555 w580 w605 w630 w655 w680 w705 w730 w755 w780 w805 w830 w855 w880 w905 w930 w955 w980 w1005 w1030 w1055 w1080 w1105 w1130 w1155 w1180 w1205 w1230 w1255 w1280 w1305 w1330 w1355 w1380 w1405 w1430 w1455 w1481 w1512 w1542 w1567 w1592 w1617 w1642 w1667 w1692 w1717 w1742 w1767 w1792 w1817 w1842 w1867 w1892 w1917 w1942 w1967 w1992 w2017 w2042 w2067 w2092 w2119 w2144 w2169 w2194 w2219 w2244 w2269 w2294 w2319 w2344 w2369 w2394 w2419 w2444 w2469 w2494 w2519 w2544 w2569 w2594 w2619 w2644 w2669 w2694 w2719 w2744 w2769 w2794 w2819 w2844 w2869 w2894 w2919 w2944 w2969 w2994 w3019 w3044 w3069 w3094 w3122 w3147 w3172 w3197 w3222 w3247 w3272 w3297 w3322 w3347 w3372 w3397 w3422 w3447 w3472 w3497 w3522 w3547 w3572 w3597 w3622 w3647 w3672 w3697 w3722 w3747 w3772 w3797 w3822 w3847 w3872 w3897 w3922 w3947 w3972 w3997 w4022 w4047 w4072 w4098 w4123 w4148]
      tunnel: w17 -> [w23 w48 w72 w98 w123 w148 w173 w198 w223 w248 w273 w298 w323 w348 w373 w398 w423 w448 w473 w498 w523 w548 w573 w598 w623 w648 w673 w698 w723 w748 w773 w798 w823 w848 w873 w898 w923 w948 w973 w998 w1023 w1048 w1073 w1098 w1123 w1148 w1173 w1198 w1223 w1248 w1273 w1298 w1323 w1348 w1373 w1398 w1423 w1448 w1474 w1505 w1535 w1560 w1585 w1610 w1635 w1660 w1685 w1710 w1735 w1760 w1785 w1810 w1835 w1860 w1885 w1910 w1935 w1960 w1985 w2010 w2035 w2060 w2085 w2112 w2137 w2162 w2187 w2212 w2237 w2262 w2287 w2312 w2337 w2362 w2387 w2412 w2437 w2462 w2487 w2512 w2537 w2562 w2587 w2612 w2637 w2662 w2687 w2712 w2737 w2762 w2787 w2812 w2837 w2862 w2887 w2912 w2937 w2962 w2987 w3012 w3037 w3062 w3087 w3116 w3141 w3166 w3191 w3216 w3241 w3266 w3291 w3316 w3340 w3365 w3390 w3415 w3440 w3465 w3490 w3515 w3540 w3565 w3590 w3615 w3640 w3665 w3690 w3715 w3740 w3765 w3790 w3815 w3840 w3865 w3890 w3915 w3940 w3965 w3990 w4015 w4040 w4065 w4091 w4116 w4141]
      tunnel: w15 -> [w26 w51 w76 w101 w126 w151 w176 w201 w226 w251 w276 w301 w326 w351 w376 w401 w426 w451 w476 w501 w526 w551 w576 w601 w626 w651 w676 w701 w726 w751 w776 w801 w826 w851 w876 w901 w926 w951 w976 w1001 w1026 w1051 w1076 w1101 w1126 w1151 w1176 w1201 w1226 w1251 w1276 w1301 w1326 w1351 w1376 w1401 w1426 w1451 w1477 w1508 w1538 w1563 w1588 w1613 w1638 w1663 w1688 w1713 w1738 w1763 w1788 w1813 w1838 w1863 w1888 w1913 w1938 w1963 w1988 w2013 w2038 w2063 w2088 w2115 w2140 w2165 w2190 w2215 w2240 w2265 w2290 w2315 w2340 w2365 w2390 w2415 w2440 w2465 w2490 w2515 w2540 w2565 w2590 w2615 w2640 w2665 w2690 w2715 w2740 w2765 w2790 w2815 w2840 w2865 w2890 w2915 w2940 w2965 w2990 w3015 w3040 w3065 w3090 w3113 w3140 w3165 w3190 w3215 w3240 w3265 w3290 w3315 w3343 w3368 w3393 w3418 w3443 w3468 w3493 w3518 w3543 w3568 w3593 w3618 w3643 w3668 w3693 w3718 w3743 w3768 w3793 w3818 w3843 w3868 w3893 w3918 w3943 w3968 w3993 w4018 w4043 w4068 w4094 w4119 w4144]
      tunnel: w14 -> [w28 w53 w78 w103 w128 w153 w178 w203 w228 w253 w278 w303 w328 w353 w378 w403 w428 w453 w478 w503 w528 w553 w578 w603 w628 w653 w678 w703 w728 w753 w778 w803 w828 w853 w878 w903 w928 w953 w978 w1003 w1028 w1053 w1078 w1103 w1128 w1153 w1178 w1203 w1228 w1253 w1278 w1303 w1328 w1353 w1378 w1403 w1428 w1453 w1479 w1510 w1540 w1565 w1590 w1615 w1640 w1665 w1690 w1715 w1740 w1765 w1790 w1815 w1840 w1865 w1890 w1915 w1940 w1965 w1990 w2015 w2040 w2065 w2090 w2117 w2142 w2167 w2192 w2217 w2242 w2267 w2292 w2317 w2342 w2367 w2392 w2417 w2442 w2467 w2492 w2517 w2542 w2567 w2592 w2617 w2642 w2667 w2692 w2717 w2742 w2767 w2792 w2817 w2842 w2867 w2892 w2917 w2942 w2967 w2992 w3017 w3042 w3067 w3092 w3120 w3145 w3170 w3195 w3220 w3245 w3270 w3295 w3320 w3345 w3370 w3395 w3420 w3445 w3470 w3495 w3520 w3545 w3570 w3595 w3620 w3645 w3670 w3695 w3720 w3745 w3770 w3795 w3820 w3845 w3870 w3895 w3920 w3945 w3970 w3995 w4020 w4045 w4070 w4096 w4121 w4146]
      tunnel: [w27 w52 w77 w102 w127 w152 w177 w202 w227 w252 w277 w302 w327 w352 w377 w402 w427 w452 w477 w502 w527 w552 w577 w602 w627 w652 w677 w702 w727 w752 w777 w802 w827 w852 w877 w902 w927 w952 w977 w1002 w1027 w1052 w1077 w1102 w1127 w1152 w1177 w1202 w1227 w1252 w1277 w1302 w1327 w1352 w1377 w1402 w1427 w1452 w1478 w1509 w1539 w1564 w1589 w1614 w1639 w1664 w1689 w1714 w1739 w1764 w1789 w1814 w1839 w1864 w1889 w1914 w1939 w1964 w1989 w2014 w2039 w2064 w2089 w2116 w2141 w2166 w2191 w2216 w2241 w2266 w2291 w2316 w2341 w2366 w2391 w2416 w2441 w2466 w2491 w2516 w2541 w2566 w2591 w2616 w2641 w2666 w2691 w2716 w2741 w2766 w2791 w2816 w2841 w2866 w2891 w2916 w2941 w2966 w2991 w3016 w3041 w3066 w3091 w3119 w3144 w3169 w3194 w3219 w3244 w3269 w3294 w3319 w3344 w3369 w3394 w3419 w3444 w3469 w3494 w3519 w3544 w3569 w3594 w3619 w3644 w3669 w3694 w3719 w3744 w3769 w3794 w3819 w3844 w3869 w3894 w3919 w3944 w3969 w3994 w4019 w4044 w4069 w4095 w4120 w4145] -> w13
      tunnel: [w25 w50 w75 w100 w125 w150 w175 w200 w225 w250 w275 w300 w325 w350 w375 w400 w425 w450 w475 w500 w525 w550 w575 w600 w625 w650 w675 w700 w725 w750 w775 w800 w825 w850 w875 w900 w925 w950 w975 w1000 w1025 w1050 w1075 w1100 w1125 w1150 w1175 w1200 w1225 w1250 w1275 w1300 w1325 w1350 w1375 w1400 w1425 w1450 w1476 w1507 w1537 w1562 w1587 w1612 w1637 w1662 w1687 w1712 w1737 w1762 w1787 w1812 w1837 w1862 w1887 w1912 w1937 w1962 w1987 w2012 w2037 w2062 w2087 w2114 w2139 w2164 w2189 w2214 w2239 w2264 w2289 w2314 w2339 w2364 w2389 w2414 w2439 w2464 w2489 w2514 w2539 w2564 w2589 w2614 w2639 w2664 w2689 w2714 w2739 w2764 w2789 w2814 w2839 w2864 w2889 w2914 w2939 w2964 w2989 w3014 w3039 w3064 w3089 w3118 w3143 w3168 w3193 w3218 w3243 w3268 w3293 w3318 w3342 w3367 w3392 w3417 w3442 w3467 w3492 w3517 w3542 w3567 w3592 w3617 w3642 w3667 w3692 w3717 w3742 w3767 w3792 w3817 w3842 w3867 w3892 w3917 w3942 w3967 w3992 w4017 w4042 w4067 w4093 w4118 w4143] -> w12
      tunnel: [w24 w49 w73 w99 w124 w149 w174 w199 w224 w249 w274 w299 w324 w349 w374 w399 w424 w449 w474 w499 w524 w549 w574 w599 w624 w649 w674 w699 w724 w749 w774 w799 w824 w849 w874 w899 w924 w949 w974 w999 w1024 w1049 w1074 w1099 w1124 w1149 w1174 w1199 w1224 w1249 w1274 w1299 w1324 w1349 w1374 w1399 w1424 w1449 w1475 w1506 w1536 w1561 w1586 w1611 w1636 w1661 w1686 w1711 w1736 w1761 w1786 w1811 w1836 w1861 w1886 w1911 w1936 w1961 w1986 w2011 w2036 w2061 w2086 w2113 w2138 w2163 w2188 w2213 w2238 w2263 w2288 w2313 w2338 w2363 w2388 w2413 w2438 w2463 w2488 w2513 w2538 w2563 w2588 w2613 w2638 w2663 w2688 w2713 w2738 w2763 w2788 w2813 w2838 w2863 w2888 w2913 w2938 w2963 w2988 w3013 w3038 w3063 w3088 w3117 w3142 w3167 w3192 w3217 w3242 w3267 w3292 w3317 w3341 w3366 w3391 w3416 w3441 w3466 w3491 w3516 w3541 w3566 w3591 w3616 w3641 w3666 w3691 w3716 w3741 w3766 w3791 w3816 w3841 w3866 w3891 w3916 w3941 w3966 w3991 w4016 w4041 w4066 w4092 w4117 w4142] -> w11
      tunnel: w10 -> [_ _ _ _ _ _ _ _ _ _ _ _ _ _ _ _ _ _ _ _ _ _ _ _ _ _ _ _ _ _ _ _ _ _ _ _ _ _ _ _ _ _ _ _ _ _ _ _ _ _ _ _ _ _ _ _ _ _ w1472 _ _ _ _ _ _ _ _ _ _ _ _ _ _ _ _ _ _ _ _ _ _ _ _ _ _ _ _ _ _ _ _ _ _ _ _ _ _ _ _ _ _ _ _ _ _ _ _ _ _ _ _ _ _ _ _ _ _ _ _ _ _ _ _ _ _ _ _ _ _ _ _ _ _ _ _ _ _ _ _ _ _ _ _ _ _ _ _ _ _ _ _ _ _ _ _ _ _ _ _ _ _ _ _ _ _]
      tunnel: w9 -> [_ _ _ _ _ _ _ _ _ _ _ _ _ _ _ _ _ _ _ _ _ _ _ _ _ _ _ _ _ _ _ _ _ _ _ _ _ _ _ _ _ _ _ _ _ _ _ _ _ _ _ _ _ _ _ _ _ _ _ w1503 _ _ _ _ _ _ _ _ _ _ _ _ _ _ _ _ _ _ _ _ _ _ _ _ _ _ _ _ _ _ _ _ _ _ _ _ _ _ _ _ _ _ _ _ _ _ _ _ _ _ _ _ _ _ _ _ _ _ _ _ _ _ _ _ _ _ _ _ _ _ _ _ _ _ _ _ _ _ _ _ _ _ _ _ _ _ _ _ _ _ _ _ _ _ _ _ _ _ _ _ _ _ _ _ _]
      frame "GUI:Visible Settings Tab" {
        n4 = case shown="True" w30 {
          tunnel: w29 -> [w38 w42]
          tunnel: w28 -> [w37 w45]
          tunnel: [w36 w44] -> w27
          tunnel: w26 -> [w35 w43]
          tunnel: [w34 w40] -> w25
          tunnel: "Visible Settings Tab" -> [w33 w46]
          tunnel: [w31 w39] -> w24
          tunnel: w23 -> [_ w39]
          frame False {
            n5 = Get Variant Attribute(Variant=w37, name=w38, default value (empty Variant)=w33, error in=w35) -> (duplicate Variant=w36:variant, value=w32:string, error out=w34:errorcluster)  [unwired: 1 out]
            n6 = To Variant(anything=w32) -> (Variant=w31:variant)
          }
          frame True {
            n7 = Variant To Data(type=w46, Variant=w39) -> (data=w41:string)  [unwired: 1 in, 1 out]
            n8 = Set Variant Attribute(Variant=w45, name=w42, value=w41, error in=w43) -> (Variant out=w44:variant, error out=w40:errorcluster)  [unwired: 1 out]
          }
        }
      }
      frame "GUI:Last Run Version" {
        n9 = case shown="True" w55 {
          tunnel: w54 -> [w63 w67]
          tunnel: w53 -> [w62 w70]
          tunnel: [w61 w69] -> w52
          tunnel: w51 -> [w60 w68]
          tunnel: [w59 w65] -> w50
          tunnel: "Last Run Version" -> [w58 w71]
          tunnel: [w56 w64] -> w49
          tunnel: w48 -> [_ w64]
          frame False {
            n10 = Get Variant Attribute(Variant=w62, name=w63, default value (empty Variant)=w58, error in=w60) -> (duplicate Variant=w61:variant, value=w57:string, error out=w59:errorcluster)  [unwired: 1 out]
            n11 = To Variant(anything=w57) -> (Variant=w56:variant)
          }
          frame True {
            n12 = Variant To Data(type=w71, Variant=w64) -> (data=w66:string)  [unwired: 1 in, 1 out]
            n13 = Set Variant Attribute(Variant=w70, name=w67, value=w66, error in=w68) -> (Variant out=w69:variant, error out=w65:errorcluster)  [unwired: 1 out]
          }
        }
      }
      frame "Source Image:Use Image Histogram for Contrast", Default {
        n14 = case shown="True" w80 {
          tunnel: w79 -> [w88 w92]
          tunnel: w78 -> [w87 w95]
          tunnel: [w86 w94] -> w77
          tunnel: w76 -> [w85 w93]
          tunnel: [w84 w90] -> w75
          tunnel: "Use Image Histogram for Contrast" -> [w83 w96]
          tunnel: [w81 w89] -> w73
          tunnel: w72 -> [_ w89]
          frame False {
            n15 = Get Variant Attribute(Variant=w87, name=w88, default value (empty Variant)=w83, error in=w85) -> (duplicate Variant=w86:variant, value=w82:bool, error out=w84:errorcluster)  [unwired: 1 out]
            n16 = To Variant(anything=w82) -> (Variant=w81:variant)
          }
          frame True {
            n17 = Variant To Data(type=w96, Variant=w89) -> (data=w91:bool)  [unwired: 1 in, 1 out]
            n18 = Set Variant Attribute(Variant=w95, name=w92, value=w91, error in=w93) -> (Variant out=w94:variant, error out=w90:errorcluster)  [unwired: 1 out]
          }
        }
      }
      frame "Source Image:Low Count Pixels Rejection Options" {
        n19 = case shown="True" w105 {
          tunnel: w104 -> [w113 w117]
          tunnel: w103 -> [w112 w120]
          tunnel: [w111 w119] -> w102
          tunnel: w101 -> [w110 w118]
          tunnel: [w109 w115] -> w100
          tunnel: "Low Count Pixels Rejection Options" -> [w108 w121]
          tunnel: [w106 w114] -> w99
          tunnel: w98 -> [_ w114]
          frame False {
            n20 = Get Variant Attribute(Variant=w112, name=w113, default value (empty Variant)=w108, error in=w110) -> (duplicate Variant=w111:variant, value=w107:T4, error out=w109:errorcluster)  [unwired: 1 out]
            n21 = To Variant(anything=w107) -> (Variant=w106:variant)
          }
          frame True {
            n22 = Variant To Data(type=w121, Variant=w114) -> (data=w116:T4)  [unwired: 1 in, 1 out]
            n23 = Set Variant Attribute(Variant=w120, name=w117, value=w116, error in=w118) -> (Variant out=w119:variant, error out=w115:errorcluster)  [unwired: 1 out]
          }
        }
      }
      frame "Source Image:High Count Pixels Rejection Options" {
        n24 = case shown="True" w130 {
          tunnel: w129 -> [w138 w142]
          tunnel: w128 -> [w137 w145]
          tunnel: [w136 w144] -> w127
          tunnel: w126 -> [w135 w143]
          tunnel: [w134 w140] -> w125
          tunnel: "High Count Pixels Rejection Options" -> [w133 w146]
          tunnel: [w131 w139] -> w124
          tunnel: w123 -> [_ w139]
          frame False {
            n25 = Get Variant Attribute(Variant=w137, name=w138, default value (empty Variant)=w133, error in=w135) -> (duplicate Variant=w136:variant, value=w132:T5, error out=w134:errorcluster)  [unwired: 1 out]
            n26 = To Variant(anything=w132) -> (Variant=w131:variant)
          }
          frame True {
            n27 = Variant To Data(type=w146, Variant=w139) -> (data=w141:T5)  [unwired: 1 in, 1 out]
            n28 = Set Variant Attribute(Variant=w145, name=w142, value=w141, error in=w143) -> (Variant out=w144:variant, error out=w140:errorcluster)  [unwired: 1 out]
          }
        }
      }
      frame "Source Image:Use Image Brightness" {
        n29 = case shown="True" w155 {
          tunnel: w154 -> [w163 w167]
          tunnel: w153 -> [w162 w170]
          tunnel: [w161 w169] -> w152
          tunnel: w151 -> [w160 w168]
          tunnel: [w159 w165] -> w150
          tunnel: "Use Image Brightness" -> [w158 w171]
          tunnel: [w156 w164] -> w149
          tunnel: w148 -> [_ w164]
          frame False {
            n30 = Get Variant Attribute(Variant=w162, name=w163, default value (empty Variant)=w158, error in=w160) -> (duplicate Variant=w161:variant, value=w157:bool, error out=w159:errorcluster)  [unwired: 1 out]
            n31 = To Variant(anything=w157) -> (Variant=w156:variant)
          }
          frame True {
            n32 = Variant To Data(type=w171, Variant=w164) -> (data=w166:bool)  [unwired: 1 in, 1 out]
            n33 = Set Variant Attribute(Variant=w170, name=w167, value=w166, error in=w168) -> (Variant out=w169:variant, error out=w165:errorcluster)  [unwired: 1 out]
          }
        }
      }
      frame "Source Image:Blend Overlay with Image Background" {
        n34 = case shown="True" w180 {
          tunnel: w179 -> [w188 w192]
          tunnel: w178 -> [w187 w195]
          tunnel: [w186 w194] -> w177
          tunnel: w176 -> [w185 w193]
          tunnel: [w184 w190] -> w175
          tunnel: "Blend Overlay with Image Background" -> [w183 w196]
          tunnel: [w181 w189] -> w174
          tunnel: w173 -> [_ w189]
          frame False {
            n35 = Get Variant Attribute(Variant=w187, name=w188, default value (empty Variant)=w183, error in=w185) -> (duplicate Variant=w186:variant, value=w182:bool, error out=w184:errorcluster)  [unwired: 1 out]
            n36 = To Variant(anything=w182) -> (Variant=w181:variant)
          }
          frame True {
            n37 = Variant To Data(type=w196, Variant=w189) -> (data=w191:bool)  [unwired: 1 in, 1 out]
            n38 = Set Variant Attribute(Variant=w195, name=w192, value=w191, error in=w193) -> (Variant out=w194:variant, error out=w190:errorcluster)  [unwired: 1 out]
          }
        }
      }
      frame "Source Image:Use Fixed ROI Diameter" {
        n39 = case shown="True" w205 {
          tunnel: w204 -> [w213 w217]
          tunnel: w203 -> [w212 w220]
          tunnel: [w211 w219] -> w202
          tunnel: w201 -> [w210 w218]
          tunnel: [w209 w215] -> w200
          tunnel: "Use Fixed ROI Diameter" -> [w208 w221]
          tunnel: [w206 w214] -> w199
          tunnel: w198 -> [_ w214]
          frame False {
            n40 = Get Variant Attribute(Variant=w212, name=w213, default value (empty Variant)=w208, error in=w210) -> (duplicate Variant=w211:variant, value=w207:bool, error out=w209:errorcluster)  [unwired: 1 out]
            n41 = To Variant(anything=w207) -> (Variant=w206:variant)
          }
          frame True {
            n42 = Variant To Data(type=w221, Variant=w214) -> (data=w216:bool)  [unwired: 1 in, 1 out]
            n43 = Set Variant Attribute(Variant=w220, name=w217, value=w216, error in=w218) -> (Variant out=w219:variant, error out=w215:errorcluster)  [unwired: 1 out]
          }
        }
      }
      frame "Source Image:ROI Diameter" {
        n44 = case shown="True" w230 {
          tunnel: w229 -> [w238 w242]
          tunnel: w228 -> [w237 w245]
          tunnel: [w236 w244] -> w227
          tunnel: w226 -> [w235 w243]
          tunnel: [w234 w240] -> w225
          tunnel: "ROI Diameter" -> [w233 w246]
          tunnel: [w231 w239] -> w224
          tunnel: w223 -> [_ w239]
          frame False {
            n45 = Get Variant Attribute(Variant=w237, name=w238, default value (empty Variant)=w233, error in=w235) -> (duplicate Variant=w236:variant, value=w232:i32, error out=w234:errorcluster)  [unwired: 1 out]
            n46 = To Variant(anything=w232) -> (Variant=w231:variant)
          }
          frame True {
            n47 = Variant To Data(type=w246, Variant=w239) -> (data=w241:i32)  [unwired: 1 in, 1 out]
            n48 = Set Variant Attribute(Variant=w245, name=w242, value=w241, error in=w243) -> (Variant out=w244:variant, error out=w240:errorcluster)  [unwired: 1 out]
          }
        }
      }
      frame "Source Image:ROI Center Color" {
        n49 = case shown="True" w255 {
          tunnel: w254 -> [w263 w267]
          tunnel: w253 -> [w262 w270]
          tunnel: [w261 w269] -> w252
          tunnel: w251 -> [w260 w268]
          tunnel: [w259 w265] -> w250
          tunnel: "ROI Center Color" -> [w258 w271]
          tunnel: [w256 w264] -> w249
          tunnel: w248 -> [_ w264]
          frame False {
            n50 = Get Variant Attribute(Variant=w262, name=w263, default value (empty Variant)=w258, error in=w260) -> (duplicate Variant=w261:variant, value=w257:u32, error out=w259:errorcluster)  [unwired: 1 out]
            n51 = To Variant(anything=w257) -> (Variant=w256:variant)
          }
          frame True {
            n52 = Variant To Data(type=w271, Variant=w264) -> (data=w266:u32)  [unwired: 1 in, 1 out]
            n53 = Set Variant Attribute(Variant=w270, name=w267, value=w266, error in=w268) -> (Variant out=w269:variant, error out=w265:errorcluster)  [unwired: 1 out]
          }
        }
      }
      frame "Source Image:Peak Threshold" {
        n54 = case shown="True" w280 {
          tunnel: w279 -> [w288 w292]
          tunnel: w278 -> [w287 w295]
          tunnel: [w286 w294] -> w277
          tunnel: w276 -> [w285 w293]
          tunnel: [w284 w290] -> w275
          tunnel: "Peak Threshold" -> [w283 w296]
          tunnel: [w281 w289] -> w274
          tunnel: w273 -> [_ w289]
          frame False {
            n55 = Get Variant Attribute(Variant=w287, name=w288, default value (empty Variant)=w283, error in=w285) -> (duplicate Variant=w286:variant, value=w282:dbl, error out=w284:errorcluster)  [unwired: 1 out]
            n56 = To Variant(anything=w282) -> (Variant=w281:variant)
          }
          frame True {
            n57 = Variant To Data(type=w296, Variant=w289) -> (data=w291:dbl)  [unwired: 1 in, 1 out]
            n58 = Set Variant Attribute(Variant=w295, name=w292, value=w291, error in=w293) -> (Variant out=w294:variant, error out=w290:errorcluster)  [unwired: 1 out]
          }
        }
      }
      frame "Source Image:Intensity Threshold" {
        n59 = case shown="True" w305 {
          tunnel: w304 -> [w313 w317]
          tunnel: w303 -> [w312 w320]
          tunnel: [w311 w319] -> w302
          tunnel: w301 -> [w310 w318]
          tunnel: [w309 w315] -> w300
          tunnel: "Intensity Threshold" -> [w308 w321]
          tunnel: [w306 w314] -> w299
          tunnel: w298 -> [_ w314]
          frame False {
            n60 = Get Variant Attribute(Variant=w312, name=w313, default value (empty Variant)=w308, error in=w310) -> (duplicate Variant=w311:variant, value=w307:dbl, error out=w309:errorcluster)  [unwired: 1 out]
            n61 = To Variant(anything=w307) -> (Variant=w306:variant)
          }
          frame True {
            n62 = Variant To Data(type=w321, Variant=w314) -> (data=w316:dbl)  [unwired: 1 in, 1 out]
            n63 = Set Variant Attribute(Variant=w320, name=w317, value=w316, error in=w318) -> (Variant out=w319:variant, error out=w315:errorcluster)  [unwired: 1 out]
          }
        }
      }
      frame "Source Image:Image Binning Options" {
        n64 = case shown="True" w330 {
          tunnel: w329 -> [w338 w342]
          tunnel: w328 -> [w337 w345]
          tunnel: [w336 w344] -> w327
          tunnel: w326 -> [w335 w343]
          tunnel: [w334 w340] -> w325
          tunnel: "Image Binning Options" -> [w333 w346]
          tunnel: [w331 w339] -> w324
          tunnel: w323 -> [_ w339]
          frame False {
            n65 = Get Variant Attribute(Variant=w337, name=w338, default value (empty Variant)=w333, error in=w335) -> (duplicate Variant=w336:variant, value=w332:T7, error out=w334:errorcluster)  [unwired: 1 out]
            n66 = To Variant(anything=w332) -> (Variant=w331:variant)
          }
          frame True {
            n67 = Variant To Data(type=w346, Variant=w339) -> (data=w341:T7)  [unwired: 1 in, 1 out]
            n68 = Set Variant Attribute(Variant=w345, name=w342, value=w341, error in=w343) -> (Variant out=w344:variant, error out=w340:errorcluster)  [unwired: 1 out]
          }
        }
      }
      frame "Source Image:Image Smoothing Options" {
        n69 = case shown="True" w355 {
          tunnel: w354 -> [w363 w367]
          tunnel: w353 -> [w362 w370]
          tunnel: [w361 w369] -> w352
          tunnel: w351 -> [w360 w368]
          tunnel: [w359 w365] -> w350
          tunnel: "Image Smoothing Options" -> [w358 w371]
          tunnel: [w356 w364] -> w349
          tunnel: w348 -> [_ w364]
          frame False {
            n70 = Get Variant Attribute(Variant=w362, name=w363, default value (empty Variant)=w358, error in=w360) -> (duplicate Variant=w361:variant, value=w357:T9, error out=w359:errorcluster)  [unwired: 1 out]
            n71 = To Variant(anything=w357) -> (Variant=w356:variant)
          }
          frame True {
            n72 = Variant To Data(type=w371, Variant=w364) -> (data=w366:T9)  [unwired: 1 in, 1 out]
            n73 = Set Variant Attribute(Variant=w370, name=w367, value=w366, error in=w368) -> (Variant out=w369:variant, error out=w365:errorcluster)  [unwired: 1 out]
          }
        }
      }
      frame "Source Image:Image Histogram Active" {
        w372 = FALSE  # Not a Settings Window Control
        n74 = case shown="True" w380 {
          tunnel: w379 -> [w388 w392]
          tunnel: w378 -> [w387 w395]
          tunnel: [w386 w394] -> w377
          tunnel: w376 -> [w385 w393]
          tunnel: [w384 w390] -> w375
          tunnel: w372 -> [w383 w396]
          tunnel: [w381 w389] -> w374
          tunnel: w373 -> [_ w389]
          frame False {
            n75 = Get Variant Attribute(Variant=w387, name=w388, default value (empty Variant)=w383, error in=w385) -> (duplicate Variant=w386:variant, value=w382:bool, error out=w384:errorcluster)  [unwired: 1 out]
            n76 = To Variant(anything=w382) -> (Variant=w381:variant)
          }
          frame True {
            n77 = Variant To Data(type=w396, Variant=w389) -> (data=w391:bool)  [unwired: 1 in, 1 out]
            n78 = Set Variant Attribute(Variant=w395, name=w392, value=w391, error in=w393) -> (Variant out=w394:variant, error out=w390:errorcluster)  [unwired: 1 out]
          }
        }
      }
      frame "Source Image:Invert Binary Mask" {
        n79 = case shown="True" w405 {
          tunnel: w404 -> [w413 w417]
          tunnel: w403 -> [w412 w420]
          tunnel: [w411 w419] -> w402
          tunnel: w401 -> [w410 w418]
          tunnel: [w409 w415] -> w400
          tunnel: "Invert Binary Mask" -> [w408 w421]
          tunnel: [w406 w414] -> w399
          tunnel: w398 -> [_ w414]
          frame False {
            n80 = Get Variant Attribute(Variant=w412, name=w413, default value (empty Variant)=w408, error in=w410) -> (duplicate Variant=w411:variant, value=w407:bool, error out=w409:errorcluster)  [unwired: 1 out]
            n81 = To Variant(anything=w407) -> (Variant=w406:variant)
          }
          frame True {
            n82 = Variant To Data(type=w421, Variant=w414) -> (data=w416:bool)  [unwired: 1 in, 1 out]
            n83 = Set Variant Attribute(Variant=w420, name=w417, value=w416, error in=w418) -> (Variant out=w419:variant, error out=w415:errorcluster)  [unwired: 1 out]
          }
        }
      }
      frame "Source Image:Hot Pixel Removal" {
        n84 = case shown="True" w430 {
          tunnel: w429 -> [w438 w442]
          tunnel: w428 -> [w437 w445]
          tunnel: [w436 w444] -> w427
          tunnel: w426 -> [w435 w443]
          tunnel: [w434 w440] -> w425
          tunnel: "Hot Pixel Removal" -> [w433 w446]
          tunnel: [w431 w439] -> w424
          tunnel: w423 -> [_ w439]
          frame False {
            n85 = Get Variant Attribute(Variant=w437, name=w438, default value (empty Variant)=w433, error in=w435) -> (duplicate Variant=w436:variant, value=w432:T6, error out=w434:errorcluster)  [unwired: 1 out]
            n86 = To Variant(anything=w432) -> (Variant=w431:variant)
          }
          frame True {
            n87 = Variant To Data(type=w446, Variant=w439) -> (data=w441:T6)  [unwired: 1 in, 1 out]
            n88 = Set Variant Attribute(Variant=w445, name=w442, value=w441, error in=w443) -> (Variant out=w444:variant, error out=w440:errorcluster)  [unwired: 1 out]
          }
        }
      }
      frame "Source Image:Overlay Analyzed ROI Center" {
        n89 = case shown="True" w455 {
          tunnel: w454 -> [w463 w467]
          tunnel: w453 -> [w462 w470]
          tunnel: [w461 w469] -> w452
          tunnel: w451 -> [w460 w468]
          tunnel: [w459 w465] -> w450
          tunnel: "Overlay Analyzed ROI Center" -> [w458 w471]
          tunnel: [w456 w464] -> w449
          tunnel: w448 -> [_ w464]
          frame False {
            n90 = Get Variant Attribute(Variant=w462, name=w463, default value (empty Variant)=w458, error in=w460) -> (duplicate Variant=w461:variant, value=w457:bool, error out=w459:errorcluster)  [unwired: 1 out]
            n91 = To Variant(anything=w457) -> (Variant=w456:variant)
          }
          frame True {
            n92 = Variant To Data(type=w471, Variant=w464) -> (data=w466:bool)  [unwired: 1 in, 1 out]
            n93 = Set Variant Attribute(Variant=w470, name=w467, value=w466, error in=w468) -> (Variant out=w469:variant, error out=w465:errorcluster)  [unwired: 1 out]
          }
        }
      }
      frame "Source Image:Auto-Adjust Contrast" {
        w472 = FALSE  # Not a Settings Window Control
        n94 = case shown="True" w480 {
          tunnel: w479 -> [w488 w492]
          tunnel: w478 -> [w487 w495]
          tunnel: [w486 w494] -> w477
          tunnel: w476 -> [w485 w493]
          tunnel: [w484 w490] -> w475
          tunnel: w472 -> [w483 w496]
          tunnel: [w481 w489] -> w474
          tunnel: w473 -> [_ w489]
          frame False {
            n95 = Get Variant Attribute(Variant=w487, name=w488, default value (empty Variant)=w483, error in=w485) -> (duplicate Variant=w486:variant, value=w482:bool, error out=w484:errorcluster)  [unwired: 1 out]
            n96 = To Variant(anything=w482) -> (Variant=w481:variant)
          }
          frame True {
            n97 = Variant To Data(type=w496, Variant=w489) -> (data=w491:bool)  [unwired: 1 in, 1 out]
            n98 = Set Variant Attribute(Variant=w495, name=w492, value=w491, error in=w493) -> (Variant out=w494:variant, error out=w490:errorcluster)  [unwired: 1 out]
          }
        }
      }
      frame "Source Image:Histogram Lower Percentile" {
        w497 = 1.0  # Not a Settings Window Control
        n99 = case shown="True" w505 {
          tunnel: w504 -> [w513 w517]
          tunnel: w503 -> [w512 w520]
          tunnel: [w511 w519] -> w502
          tunnel: w501 -> [w510 w518]
          tunnel: [w509 w515] -> w500
          tunnel: w497 -> [w508 w521]
          tunnel: [w506 w514] -> w499
          tunnel: w498 -> [_ w514]
          frame False {
            n100 = Get Variant Attribute(Variant=w512, name=w513, default value (empty Variant)=w508, error in=w510) -> (duplicate Variant=w511:variant, value=w507:dbl, error out=w509:errorcluster)  [unwired: 1 out]
            n101 = To Variant(anything=w507) -> (Variant=w506:variant)
          }
          frame True {
            n102 = Variant To Data(type=w521, Variant=w514) -> (data=w516:dbl)  [unwired: 1 in, 1 out]
            n103 = Set Variant Attribute(Variant=w520, name=w517, value=w516, error in=w518) -> (Variant out=w519:variant, error out=w515:errorcluster)  [unwired: 1 out]
          }
        }
      }
      frame "Source Image:Histogram Upper Percentile" {
        w522 = 1.0  # Not a Settings Window Control
        n104 = case shown="True" w530 {
          tunnel: w529 -> [w538 w542]
          tunnel: w528 -> [w537 w545]
          tunnel: [w536 w544] -> w527
          tunnel: w526 -> [w535 w543]
          tunnel: [w534 w540] -> w525
          tunnel: w522 -> [w533 w546]
          tunnel: [w531 w539] -> w524
          tunnel: w523 -> [_ w539]
          frame False {
            n105 = Get Variant Attribute(Variant=w537, name=w538, default value (empty Variant)=w533, error in=w535) -> (duplicate Variant=w536:variant, value=w532:dbl, error out=w534:errorcluster)  [unwired: 1 out]
            n106 = To Variant(anything=w532) -> (Variant=w531:variant)
          }
          frame True {
            n107 = Variant To Data(type=w546, Variant=w539) -> (data=w541:dbl)  [unwired: 1 in, 1 out]
            n108 = Set Variant Attribute(Variant=w545, name=w542, value=w541, error in=w543) -> (Variant out=w544:variant, error out=w540:errorcluster)  [unwired: 1 out]
          }
        }
      }
      frame "Source Image:Save Source Image" {
        w547 = FALSE  # Save Source Image
        n109 = case shown="True" w555 {
          tunnel: w554 -> [w563 w567]
          tunnel: w553 -> [w562 w570]
          tunnel: [w561 w569] -> w552
          tunnel: w551 -> [w560 w568]
          tunnel: [w559 w565] -> w550
          tunnel: w547 -> [w558 w571]
          tunnel: [w556 w564] -> w549
          tunnel: w548 -> [_ w564]
          frame False {
            n110 = Get Variant Attribute(Variant=w562, name=w563, default value (empty Variant)=w558, error in=w560) -> (duplicate Variant=w561:variant, value=w557:bool, error out=w559:errorcluster)  [unwired: 1 out]
            n111 = To Variant(anything=w557) -> (Variant=w556:variant)
          }
          frame True {
            n112 = Variant To Data(type=w571, Variant=w564) -> (data=w566:bool)  [unwired: 1 in, 1 out]
            n113 = Set Variant Attribute(Variant=w570, name=w567, value=w566, error in=w568) -> (Variant out=w569:variant, error out=w565:errorcluster)  [unwired: 1 out]
          }
        }
      }
      frame "Source Image:Scale Bar Options" {
        n114 = case shown="True" w580 {
          tunnel: w579 -> [w588 w592]
          tunnel: w578 -> [w587 w595]
          tunnel: [w586 w594] -> w577
          tunnel: w576 -> [w585 w593]
          tunnel: [w584 w590] -> w575
          tunnel: "Scale Bar Options" -> [w583 w596]
          tunnel: [w581 w589] -> w574
          tunnel: w573 -> [_ w589]
          frame False {
            n115 = Get Variant Attribute(Variant=w587, name=w588, default value (empty Variant)=w583, error in=w585) -> (duplicate Variant=w586:variant, value=w582:T12, error out=w584:errorcluster)  [unwired: 1 out]
            n116 = To Variant(anything=w582) -> (Variant=w581:variant)
          }
          frame True {
            n117 = Variant To Data(type=w596, Variant=w589) -> (data=w591:T12)  [unwired: 1 in, 1 out]
            n118 = Set Variant Attribute(Variant=w595, name=w592, value=w591, error in=w593) -> (Variant out=w594:variant, error out=w590:errorcluster)  [unwired: 1 out]
          }
        }
      }
      frame "Source Image:Image Resolution (Pixel Size)" {
        n119 = case shown="True" w605 {
          tunnel: w604 -> [w613 w617]
          tunnel: w603 -> [w612 w620]
          tunnel: [w611 w619] -> w602
          tunnel: w601 -> [w610 w618]
          tunnel: [w609 w615] -> w600
          tunnel: "Image Resolution (Pixel Size)" -> [w608 w621]
          tunnel: [w606 w614] -> w599
          tunnel: w598 -> [_ w614]
          frame False {
            n120 = Get Variant Attribute(Variant=w612, name=w613, default value (empty Variant)=w608, error in=w610) -> (duplicate Variant=w611:variant, value=w607:dbl[unit], error out=w609:errorcluster)  [unwired: 1 out]
            n121 = To Variant(anything=w607) -> (Variant=w606:variant)
          }
          frame True {
            n122 = Variant To Data(type=w621, Variant=w614) -> (data=w616:dbl[unit])  [unwired: 1 in, 1 out]
            n123 = Set Variant Attribute(Variant=w620, name=w617, value=w616, error in=w618) -> (Variant out=w619:variant, error out=w615:errorcluster)  [unwired: 1 out]
          }
        }
      }
      frame "Source Image:Flatfield Correction" {
        n124 = case shown="True" w630 {
          tunnel: w629 -> [w638 w642]
          tunnel: w628 -> [w637 w645]
          tunnel: [w636 w644] -> w627
          tunnel: w626 -> [w635 w643]
          tunnel: [w634 w640] -> w625
          tunnel: "Flatfield Correction" -> [w633 w646]
          tunnel: [w631 w639] -> w624
          tunnel: w623 -> [_ w639]
          frame False {
            n125 = Get Variant Attribute(Variant=w637, name=w638, default value (empty Variant)=w633, error in=w635) -> (duplicate Variant=w636:variant, value=w632:T8, error out=w634:errorcluster)  [unwired: 1 out]
            n126 = To Variant(anything=w632) -> (Variant=w631:variant)
          }
          frame True {
            n127 = Variant To Data(type=w646, Variant=w639) -> (data=w641:T8)  [unwired: 1 in, 1 out]
            n128 = Set Variant Attribute(Variant=w645, name=w642, value=w641, error in=w643) -> (Variant out=w644:variant, error out=w640:errorcluster)  [unwired: 1 out]
          }
        }
      }
      frame "Source Image:Show Dead Left Columns Correction" {
        n129 = case shown="True" w655 {
          tunnel: w654 -> [w663 w667]
          tunnel: w653 -> [w662 w670]
          tunnel: [w661 w669] -> w652
          tunnel: w651 -> [w660 w668]
          tunnel: [w659 w665] -> w650
          tunnel: "Show Dead Left Columns Correction" -> [w658 w671]
          tunnel: [w656 w664] -> w649
          tunnel: w648 -> [_ w664]
          frame False {
            n130 = Get Variant Attribute(Variant=w662, name=w663, default value (empty Variant)=w658, error in=w660) -> (duplicate Variant=w661:variant, value=w657:bool, error out=w659:errorcluster)  [unwired: 1 out]
            n131 = To Variant(anything=w657) -> (Variant=w656:variant)
          }
          frame True {
            n132 = Variant To Data(type=w671, Variant=w664) -> (data=w666:bool)  [unwired: 1 in, 1 out]
            n133 = Set Variant Attribute(Variant=w670, name=w667, value=w666, error in=w668) -> (Variant out=w669:variant, error out=w665:errorcluster)  [unwired: 1 out]
          }
        }
      }
      frame "Source Image:Dead Left Columns Correction" {
        n134 = case shown="True" w680 {
          tunnel: w679 -> [w688 w692]
          tunnel: w678 -> [w687 w695]
          tunnel: [w686 w694] -> w677
          tunnel: w676 -> [w685 w693]
          tunnel: [w684 w690] -> w675
          tunnel: "Dead Left Columns Correction" -> [w683 w696]
          tunnel: [w681 w689] -> w674
          tunnel: w673 -> [_ w689]
          frame False {
            n135 = Get Variant Attribute(Variant=w687, name=w688, default value (empty Variant)=w683, error in=w685) -> (duplicate Variant=w686:variant, value=w682:bool, error out=w684:errorcluster)  [unwired: 1 out]
            n136 = To Variant(anything=w682) -> (Variant=w681:variant)
          }
          frame True {
            n137 = Variant To Data(type=w696, Variant=w689) -> (data=w691:bool)  [unwired: 1 in, 1 out]
            n138 = Set Variant Attribute(Variant=w695, name=w692, value=w691, error in=w693) -> (Variant out=w694:variant, error out=w690:errorcluster)  [unwired: 1 out]
          }
        }
      }
      frame "Source Image:Overlay ROI Median" {
        n139 = case shown="True" w705 {
          tunnel: w704 -> [w713 w717]
          tunnel: w703 -> [w712 w720]
          tunnel: [w711 w719] -> w702
          tunnel: w701 -> [w710 w718]
          tunnel: [w709 w715] -> w700
          tunnel: "Overlay ROI Median" -> [w708 w721]
          tunnel: [w706 w714] -> w699
          tunnel: w698 -> [_ w714]
          frame False {
            n140 = Get Variant Attribute(Variant=w712, name=w713, default value (empty Variant)=w708, error in=w710) -> (duplicate Variant=w711:variant, value=w707:bool, error out=w709:errorcluster)  [unwired: 1 out]
            n141 = To Variant(anything=w707) -> (Variant=w706:variant)
          }
          frame True {
            n142 = Variant To Data(type=w721, Variant=w714) -> (data=w716:bool)  [unwired: 1 in, 1 out]
            n143 = Set Variant Attribute(Variant=w720, name=w717, value=w716, error in=w718) -> (Variant out=w719:variant, error out=w715:errorcluster)  [unwired: 1 out]
          }
        }
      }
      frame "Source Image:Median Overlay Color" {
        n144 = case shown="True" w730 {
          tunnel: w729 -> [w738 w742]
          tunnel: w728 -> [w737 w745]
          tunnel: [w736 w744] -> w727
          tunnel: w726 -> [w735 w743]
          tunnel: [w734 w740] -> w725
          tunnel: "Median Overlay Color" -> [w733 w746]
          tunnel: [w731 w739] -> w724
          tunnel: w723 -> [_ w739]
          frame False {
            n145 = Get Variant Attribute(Variant=w737, name=w738, default value (empty Variant)=w733, error in=w735) -> (duplicate Variant=w736:variant, value=w732:u32, error out=w734:errorcluster)  [unwired: 1 out]
            n146 = To Variant(anything=w732) -> (Variant=w731:variant)
          }
          frame True {
            n147 = Variant To Data(type=w746, Variant=w739) -> (data=w741:u32)  [unwired: 1 in, 1 out]
            n148 = Set Variant Attribute(Variant=w745, name=w742, value=w741, error in=w743) -> (Variant out=w744:variant, error out=w740:errorcluster)  [unwired: 1 out]
          }
        }
      }
      frame "Data Information:Gate Width" {
        n149 = case shown="True" w755 {
          tunnel: w754 -> [w763 w767]
          tunnel: w753 -> [w762 w770]
          tunnel: [w761 w769] -> w752
          tunnel: w751 -> [w760 w768]
          tunnel: [w759 w765] -> w750
          tunnel: "Gate Width" -> [w758 w771]
          tunnel: [w756 w764] -> w749
          tunnel: w748 -> [_ w764]
          frame False {
            n150 = Get Variant Attribute(Variant=w762, name=w763, default value (empty Variant)=w758, error in=w760) -> (duplicate Variant=w761:variant, value=w757:dbl[unit], error out=w759:errorcluster)  [unwired: 1 out]
            n151 = To Variant(anything=w757) -> (Variant=w756:variant)
          }
          frame True {
            n152 = Variant To Data(type=w771, Variant=w764) -> (data=w766:dbl[unit])  [unwired: 1 in, 1 out]
            n153 = Set Variant Attribute(Variant=w770, name=w767, value=w766, error in=w768) -> (Variant out=w769:variant, error out=w765:errorcluster)  [unwired: 1 out]
          }
        }
      }
      frame "Data Information:Nanotime Gate Separation" {
        n154 = case shown="True" w780 {
          tunnel: w779 -> [w788 w792]
          tunnel: w778 -> [w787 w795]
          tunnel: [w786 w794] -> w777
          tunnel: w776 -> [w785 w793]
          tunnel: [w784 w790] -> w775
          tunnel: "Gate Separation" -> [w783 w796]
          tunnel: [w781 w789] -> w774
          tunnel: w773 -> [_ w789]
          frame False {
            n155 = Get Variant Attribute(Variant=w787, name=w788, default value (empty Variant)=w783, error in=w785) -> (duplicate Variant=w786:variant, value=w782:dbl[unit], error out=w784:errorcluster)  [unwired: 1 out]
            n156 = To Variant(anything=w782) -> (Variant=w781:variant)
          }
          frame True {
            n157 = Variant To Data(type=w796, Variant=w789) -> (data=w791:dbl[unit])  [unwired: 1 in, 1 out]
            n158 = Set Variant Attribute(Variant=w795, name=w792, value=w791, error in=w793) -> (Variant out=w794:variant, error out=w790:errorcluster)  [unwired: 1 out]
          }
        }
      }
      frame "Data Information:Gate Step" {
        n159 = case shown="True" w805 {
          tunnel: w804 -> [w813 w817]
          tunnel: w803 -> [w812 w820]
          tunnel: [w811 w819] -> w802
          tunnel: w801 -> [w810 w818]
          tunnel: [w809 w815] -> w800
          tunnel: "Gate Step" -> [w808 w821]
          tunnel: [w806 w814] -> w799
          tunnel: w798 -> [_ w814]
          frame False {
            n160 = Get Variant Attribute(Variant=w812, name=w813, default value (empty Variant)=w808, error in=w810) -> (duplicate Variant=w811:variant, value=w807:i32, error out=w809:errorcluster)  [unwired: 1 out]
            n161 = To Variant(anything=w807) -> (Variant=w806:variant)
          }
          frame True {
            n162 = Variant To Data(type=w821, Variant=w814) -> (data=w816:i32)  [unwired: 1 in, 1 out]
            n163 = Set Variant Attribute(Variant=w820, name=w817, value=w816, error in=w818) -> (Variant out=w819:variant, error out=w815:errorcluster)  [unwired: 1 out]
          }
        }
      }
      frame "Data Information:# Gates" {
        n164 = case shown="True" w830 {
          tunnel: w829 -> [w838 w842]
          tunnel: w828 -> [w837 w845]
          tunnel: [w836 w844] -> w827
          tunnel: w826 -> [w835 w843]
          tunnel: [w834 w840] -> w825
          tunnel: "# Gates" -> [w833 w846]
          tunnel: [w831 w839] -> w824
          tunnel: w823 -> [_ w839]
          frame False {
            n165 = Get Variant Attribute(Variant=w837, name=w838, default value (empty Variant)=w833, error in=w835) -> (duplicate Variant=w836:variant, value=w832:u32, error out=w834:errorcluster)  [unwired: 1 out]
            n166 = To Variant(anything=w832) -> (Variant=w831:variant)
          }
          frame True {
            n167 = Variant To Data(type=w846, Variant=w839) -> (data=w841:u32)  [unwired: 1 in, 1 out]
            n168 = Set Variant Attribute(Variant=w845, name=w842, value=w841, error in=w843) -> (Variant out=w844:variant, error out=w840:errorcluster)  [unwired: 1 out]
          }
        }
      }
      frame "Data Information:Gate Image Exposure" {
        n169 = case shown="True" w855 {
          tunnel: w854 -> [w863 w867]
          tunnel: w853 -> [w862 w870]
          tunnel: [w861 w869] -> w852
          tunnel: w851 -> [w860 w868]
          tunnel: [w859 w865] -> w850
          tunnel: "Gate Image Exposure" -> [w858 w871]
          tunnel: [w856 w864] -> w849
          tunnel: w848 -> [_ w864]
          frame False {
            n170 = Get Variant Attribute(Variant=w862, name=w863, default value (empty Variant)=w858, error in=w860) -> (duplicate Variant=w861:variant, value=w857:dbl[unit], error out=w859:errorcluster)  [unwired: 1 out]
            n171 = To Variant(anything=w857) -> (Variant=w856:variant)
          }
          frame True {
            n172 = Variant To Data(type=w871, Variant=w864) -> (data=w866:dbl[unit])  [unwired: 1 in, 1 out]
            n173 = Set Variant Attribute(Variant=w870, name=w867, value=w866, error in=w868) -> (Variant out=w869:variant, error out=w865:errorcluster)  [unwired: 1 out]
          }
        }
      }
      frame "Data Information:Gate Image Integration" {
        n174 = case shown="True" w880 {
          tunnel: w879 -> [w888 w892]
          tunnel: w878 -> [w887 w895]
          tunnel: [w886 w894] -> w877
          tunnel: w876 -> [w885 w893]
          tunnel: [w884 w890] -> w875
          tunnel: "Gate Image Integration" -> [w883 w896]
          tunnel: [w881 w889] -> w874
          tunnel: w873 -> [_ w889]
          frame False {
            n175 = Get Variant Attribute(Variant=w887, name=w888, default value (empty Variant)=w883, error in=w885) -> (duplicate Variant=w886:variant, value=w882:dbl[unit], error out=w884:errorcluster)  [unwired: 1 out]
            n176 = To Variant(anything=w882) -> (Variant=w881:variant)
          }
          frame True {
            n177 = Variant To Data(type=w896, Variant=w889) -> (data=w891:dbl[unit])  [unwired: 1 in, 1 out]
            n178 = Set Variant Attribute(Variant=w895, name=w892, value=w891, error in=w893) -> (Variant out=w894:variant, error out=w890:errorcluster)  [unwired: 1 out]
          }
        }
      }
      frame "Data Information:Gates to Skip" {
        n179 = case shown="True" w905 {
          tunnel: w904 -> [w913 w917]
          tunnel: w903 -> [w912 w920]
          tunnel: [w911 w919] -> w902
          tunnel: w901 -> [w910 w918]
          tunnel: [w909 w915] -> w900
          tunnel: "Gates to Skip" -> [w908 w921]
          tunnel: [w906 w914] -> w899
          tunnel: w898 -> [_ w914]
          frame False {
            n180 = Get Variant Attribute(Variant=w912, name=w913, default value (empty Variant)=w908, error in=w910) -> (duplicate Variant=w911:variant, value=w907:T16, error out=w909:errorcluster)  [unwired: 1 out]
            n181 = To Variant(anything=w907) -> (Variant=w906:variant)
          }
          frame True {
            n182 = Variant To Data(type=w921, Variant=w914) -> (data=w916:T16)  [unwired: 1 in, 1 out]
            n183 = Set Variant Attribute(Variant=w920, name=w917, value=w916, error in=w918) -> (Variant out=w919:variant, error out=w915:errorcluster)  [unwired: 1 out]
          }
        }
      }
      frame "Data Information:Gates to Keep" {
        n184 = case shown="True" w930 {
          tunnel: w929 -> [w938 w942]
          tunnel: w928 -> [w937 w945]
          tunnel: [w936 w944] -> w927
          tunnel: w926 -> [w935 w943]
          tunnel: [w934 w940] -> w925
          tunnel: "Gates to Keep" -> [w933 w946]
          tunnel: [w931 w939] -> w924
          tunnel: w923 -> [_ w939]
          frame False {
            n185 = Get Variant Attribute(Variant=w937, name=w938, default value (empty Variant)=w933, error in=w935) -> (duplicate Variant=w936:variant, value=w932:T14, error out=w934:errorcluster)  [unwired: 1 out]
            n186 = To Variant(anything=w932) -> (Variant=w931:variant)
          }
          frame True {
            n187 = Variant To Data(type=w946, Variant=w939) -> (data=w941:T14)  [unwired: 1 in, 1 out]
            n188 = Set Variant Attribute(Variant=w945, name=w942, value=w941, error in=w943) -> (Variant out=w944:variant, error out=w940:errorcluster)  [unwired: 1 out]
          }
        }
      }
      frame "Data Information:Define Gates to" {
        n189 = case shown="True" w955 {
          tunnel: w954 -> [w963 w967]
          tunnel: w953 -> [w962 w970]
          tunnel: [w961 w969] -> w952
          tunnel: w951 -> [w960 w968]
          tunnel: [w959 w965] -> w950
          tunnel: "Define Gates to" -> [w958 w971]
          tunnel: [w956 w964] -> w949
          tunnel: w948 -> [_ w964]
          frame False {
            n190 = Get Variant Attribute(Variant=w962, name=w963, default value (empty Variant)=w958, error in=w960) -> (duplicate Variant=w961:variant, value=w957:T15, error out=w959:errorcluster)  [unwired: 1 out]
            n191 = To Variant(anything=w957) -> (Variant=w956:variant)
          }
          frame True {
            n192 = Variant To Data(type=w971, Variant=w964) -> (data=w966:T15)  [unwired: 1 in, 1 out]
            n193 = Set Variant Attribute(Variant=w970, name=w967, value=w966, error in=w968) -> (Variant out=w969:variant, error out=w965:errorcluster)  [unwired: 1 out]
          }
        }
      }
      frame "Data Information:Channel Name" {
        n194 = case shown="True" w980 {
          tunnel: w979 -> [w988 w992]
          tunnel: w978 -> [w987 w995]
          tunnel: [w986 w994] -> w977
          tunnel: w976 -> [w985 w993]
          tunnel: [w984 w990] -> w975
          tunnel: "Channel Name" -> [w983 w996]
          tunnel: [w981 w989] -> w974
          tunnel: w973 -> [_ w989]
          frame False {
            n195 = Get Variant Attribute(Variant=w987, name=w988, default value (empty Variant)=w983, error in=w985) -> (duplicate Variant=w986:variant, value=w982:u16, error out=w984:errorcluster)  [unwired: 1 out]
            n196 = To Variant(anything=w982) -> (Variant=w981:variant)
          }
          frame True {
            n197 = Variant To Data(type=w996, Variant=w989) -> (data=w991:u16)  [unwired: 1 in, 1 out]
            n198 = Set Variant Attribute(Variant=w995, name=w992, value=w991, error in=w993) -> (Variant out=w994:variant, error out=w990:errorcluster)  [unwired: 1 out]
          }
        }
      }
      frame "Data Information:Available Channel Names" {
        n199 = case shown="True" w1005 {
          tunnel: w1004 -> [w1013 w1017]
          tunnel: w1003 -> [w1012 w1020]
          tunnel: [w1011 w1019] -> w1002
          tunnel: w1001 -> [w1010 w1018]
          tunnel: [w1009 w1015] -> w1000
          tunnel: "Available Gate Names" -> [w1008 w1021]
          tunnel: [w1006 w1014] -> w999
          tunnel: w998 -> [_ w1014]
          frame False {
            n200 = Get Variant Attribute(Variant=w1012, name=w1013, default value (empty Variant)=w1008, error in=w1010) -> (duplicate Variant=w1011:variant, value=w1007:string[], error out=w1009:errorcluster)  [unwired: 1 out]
            n201 = To Variant(anything=w1007) -> (Variant=w1006:variant)
          }
          frame True {
            n202 = Variant To Data(type=w1021, Variant=w1014) -> (data=w1016:string[])  [unwired: 1 in, 1 out]
            n203 = Set Variant Attribute(Variant=w1020, name=w1017, value=w1016, error in=w1018) -> (Variant out=w1019:variant, error out=w1015:errorcluster)  [unwired: 1 out]
          }
        }
      }
      frame "Data Information:Channel Arithmetic" {
        n204 = case shown="True" w1030 {
          tunnel: w1029 -> [w1038 w1042]
          tunnel: w1028 -> [w1037 w1045]
          tunnel: [w1036 w1044] -> w1027
          tunnel: w1026 -> [w1035 w1043]
          tunnel: [w1034 w1040] -> w1025
          tunnel: "Channel Arithmetic" -> [w1033 w1046]
          tunnel: [w1031 w1039] -> w1024
          tunnel: w1023 -> [_ w1039]
          frame False {
            n205 = Get Variant Attribute(Variant=w1037, name=w1038, default value (empty Variant)=w1033, error in=w1035) -> (duplicate Variant=w1036:variant, value=w1032:T13, error out=w1034:errorcluster)  [unwired: 1 out]
            n206 = To Variant(anything=w1032) -> (Variant=w1031:variant)
          }
          frame True {
            n207 = Variant To Data(type=w1046, Variant=w1039) -> (data=w1041:T13)  [unwired: 1 in, 1 out]
            n208 = Set Variant Attribute(Variant=w1045, name=w1042, value=w1041, error in=w1043) -> (Variant out=w1044:variant, error out=w1040:errorcluster)  [unwired: 1 out]
          }
        }
      }
      frame "Data Information:Background File Subtraction" {
        n209 = case shown="True" w1055 {
          tunnel: w1054 -> [w1063 w1067]
          tunnel: w1053 -> [w1062 w1070]
          tunnel: [w1061 w1069] -> w1052
          tunnel: w1051 -> [w1060 w1068]
          tunnel: [w1059 w1065] -> w1050
          tunnel: "Background File Subtraction" -> [w1058 w1071]
          tunnel: [w1056 w1064] -> w1049
          tunnel: w1048 -> [_ w1064]
          frame False {
            n210 = Get Variant Attribute(Variant=w1062, name=w1063, default value (empty Variant)=w1058, error in=w1060) -> (duplicate Variant=w1061:variant, value=w1057:bool, error out=w1059:errorcluster)  [unwired: 1 out]
            n211 = To Variant(anything=w1057) -> (Variant=w1056:variant)
          }
          frame True {
            n212 = Variant To Data(type=w1071, Variant=w1064) -> (data=w1066:bool)  [unwired: 1 in, 1 out]
            n213 = Set Variant Attribute(Variant=w1070, name=w1067, value=w1066, error in=w1068) -> (Variant out=w1069:variant, error out=w1065:errorcluster)  [unwired: 1 out]
          }
        }
      }
      frame "Data Information:Background File" {
        n214 = case shown="True" w1080 {
          tunnel: w1079 -> [w1088 w1092]
          tunnel: w1078 -> [w1087 w1095]
          tunnel: [w1086 w1094] -> w1077
          tunnel: w1076 -> [w1085 w1093]
          tunnel: [w1084 w1090] -> w1075
          tunnel: "Background File" -> [w1083 w1096]
          tunnel: [w1081 w1089] -> w1074
          tunnel: w1073 -> [_ w1089]
          frame False {
            n215 = Get Variant Attribute(Variant=w1087, name=w1088, default value (empty Variant)=w1083, error in=w1085) -> (duplicate Variant=w1086:variant, value=w1082:path, error out=w1084:errorcluster)  [unwired: 1 out]
            n216 = To Variant(anything=w1082) -> (Variant=w1081:variant)
          }
          frame True {
            n217 = Variant To Data(type=w1096, Variant=w1089) -> (data=w1091:path)  [unwired: 1 in, 1 out]
            n218 = Set Variant Attribute(Variant=w1095, name=w1092, value=w1091, error in=w1093) -> (Variant out=w1094:variant, error out=w1090:errorcluster)  [unwired: 1 out]
          }
        }
      }
      frame "Data Information:Background Scaling Factor" {
        n219 = case shown="True" w1105 {
          tunnel: w1104 -> [w1113 w1117]
          tunnel: w1103 -> [w1112 w1120]
          tunnel: [w1111 w1119] -> w1102
          tunnel: w1101 -> [w1110 w1118]
          tunnel: [w1109 w1115] -> w1100
          tunnel: "Background Scaling Factor" -> [w1108 w1121]
          tunnel: [w1106 w1114] -> w1099
          tunnel: w1098 -> [_ w1114]
          frame False {
            n220 = Get Variant Attribute(Variant=w1112, name=w1113, default value (empty Variant)=w1108, error in=w1110) -> (duplicate Variant=w1111:variant, value=w1107:dbl, error out=w1109:errorcluster)  [unwired: 1 out]
            n221 = To Variant(anything=w1107) -> (Variant=w1106:variant)
          }
          frame True {
            n222 = Variant To Data(type=w1121, Variant=w1114) -> (data=w1116:dbl)  [unwired: 1 in, 1 out]
            n223 = Set Variant Attribute(Variant=w1120, name=w1117, value=w1116, error in=w1118) -> (Variant out=w1119:variant, error out=w1115:errorcluster)  [unwired: 1 out]
          }
        }
      }
      frame "Data Information:Background Pile-up Correction" {
        n224 = case shown="True" w1130 {
          tunnel: w1129 -> [w1138 w1142]
          tunnel: w1128 -> [w1137 w1145]
          tunnel: [w1136 w1144] -> w1127
          tunnel: w1126 -> [w1135 w1143]
          tunnel: [w1134 w1140] -> w1125
          tunnel: "Background Pile-up Correction" -> [w1133 w1146]
          tunnel: [w1131 w1139] -> w1124
          tunnel: w1123 -> [_ w1139]
          frame False {
            n225 = Get Variant Attribute(Variant=w1137, name=w1138, default value (empty Variant)=w1133, error in=w1135) -> (duplicate Variant=w1136:variant, value=w1132:bool, error out=w1134:errorcluster)  [unwired: 1 out]
            n226 = To Variant(anything=w1132) -> (Variant=w1131:variant)
          }
          frame True {
            n227 = Variant To Data(type=w1146, Variant=w1139) -> (data=w1141:bool)  [unwired: 1 in, 1 out]
            n228 = Set Variant Attribute(Variant=w1145, name=w1142, value=w1141, error in=w1143) -> (Variant out=w1144:variant, error out=w1140:errorcluster)  [unwired: 1 out]
          }
        }
      }
      frame "Data Information:Background Pixel Well Capacity" {
        n229 = case shown="True" w1155 {
          tunnel: w1154 -> [w1163 w1167]
          tunnel: w1153 -> [w1162 w1170]
          tunnel: [w1161 w1169] -> w1152
          tunnel: w1151 -> [w1160 w1168]
          tunnel: [w1159 w1165] -> w1150
          tunnel: "Background Pixel Well Capacity" -> [w1158 w1171]
          tunnel: [w1156 w1164] -> w1149
          tunnel: w1148 -> [_ w1164]
          frame False {
            n230 = Get Variant Attribute(Variant=w1162, name=w1163, default value (empty Variant)=w1158, error in=w1160) -> (duplicate Variant=w1161:variant, value=w1157:u32, error out=w1159:errorcluster)  [unwired: 1 out]
            n231 = To Variant(anything=w1157) -> (Variant=w1156:variant)
          }
          frame True {
            n232 = Variant To Data(type=w1171, Variant=w1164) -> (data=w1166:u32)  [unwired: 1 in, 1 out]
            n233 = Set Variant Attribute(Variant=w1170, name=w1167, value=w1166, error in=w1168) -> (Variant out=w1169:variant, error out=w1165:errorcluster)  [unwired: 1 out]
          }
        }
      }
      frame "Data Information:Laser Period" {
        n234 = case shown="False" w1180 {
          tunnel: w1179 -> [w1188 w1192]
          tunnel: w1178 -> [w1187 w1195]
          tunnel: [w1186 w1194] -> w1177
          tunnel: w1176 -> [w1185 w1193]
          tunnel: [w1184 w1190] -> w1175
          tunnel: "Laser Period" -> [w1183 w1196]
          tunnel: [w1181 w1189] -> w1174
          tunnel: w1173 -> [_ w1189]
          frame False {
            n235 = Get Variant Attribute(Variant=w1187, name=w1188, default value (empty Variant)=w1183, error in=w1185) -> (duplicate Variant=w1186:variant, value=w1182:dbl[unit], error out=w1184:errorcluster)  [unwired: 1 out]
            n236 = To Variant(anything=w1182) -> (Variant=w1181:variant)
          }
          frame True {
            n237 = Variant To Data(type=w1196, Variant=w1189) -> (data=w1191:dbl[unit])  [unwired: 1 in, 1 out]
            n238 = Set Variant Attribute(Variant=w1195, name=w1192, value=w1191, error in=w1193) -> (Variant out=w1194:variant, error out=w1190:errorcluster)  [unwired: 1 out]
          }
        }
      }
      frame "Data Information:SYNC Period" {
        n239 = case shown="False" w1205 {
          tunnel: w1204 -> [w1213 w1217]
          tunnel: w1203 -> [w1212 w1220]
          tunnel: [w1211 w1219] -> w1202
          tunnel: w1201 -> [w1210 w1218]
          tunnel: [w1209 w1215] -> w1200
          tunnel: "SYNC Period" -> [w1208 w1221]
          tunnel: [w1206 w1214] -> w1199
          tunnel: w1198 -> [_ w1214]
          frame False {
            n240 = Get Variant Attribute(Variant=w1212, name=w1213, default value (empty Variant)=w1208, error in=w1210) -> (duplicate Variant=w1211:variant, value=w1207:dbl[unit], error out=w1209:errorcluster)  [unwired: 1 out]
            n241 = To Variant(anything=w1207) -> (Variant=w1206:variant)
          }
          frame True {
            n242 = Variant To Data(type=w1221, Variant=w1214) -> (data=w1216:dbl[unit])  [unwired: 1 in, 1 out]
            n243 = Set Variant Attribute(Variant=w1220, name=w1217, value=w1216, error in=w1218) -> (Variant out=w1219:variant, error out=w1215:errorcluster)  [unwired: 1 out]
          }
        }
      }
      frame "Data Information:Pile-up Correction" {
        n244 = case shown="True" w1230 {
          tunnel: w1229 -> [w1238 w1242]
          tunnel: w1228 -> [w1237 w1245]
          tunnel: [w1236 w1244] -> w1227
          tunnel: w1226 -> [w1235 w1243]
          tunnel: [w1234 w1240] -> w1225
          tunnel: "Pile-up Correction" -> [w1233 w1246]
          tunnel: [w1231 w1239] -> w1224
          tunnel: w1223 -> [_ w1239]
          frame False {
            n245 = Get Variant Attribute(Variant=w1237, name=w1238, default value (empty Variant)=w1233, error in=w1235) -> (duplicate Variant=w1236:variant, value=w1232:bool, error out=w1234:errorcluster)  [unwired: 1 out]
            n246 = To Variant(anything=w1232) -> (Variant=w1231:variant)
          }
          frame True {
            n247 = Variant To Data(type=w1246, Variant=w1239) -> (data=w1241:bool)  [unwired: 1 in, 1 out]
            n248 = Set Variant Attribute(Variant=w1245, name=w1242, value=w1241, error in=w1243) -> (Variant out=w1244:variant, error out=w1240:errorcluster)  [unwired: 1 out]
          }
        }
      }
      frame "Data Information:Pixel Well Capacity" {
        n249 = case shown="True" w1255 {
          tunnel: w1254 -> [w1263 w1267]
          tunnel: w1253 -> [w1262 w1270]
          tunnel: [w1261 w1269] -> w1252
          tunnel: w1251 -> [w1260 w1268]
          tunnel: [w1259 w1265] -> w1250
          tunnel: "Pixel Well Capacity" -> [w1258 w1271]
          tunnel: [w1256 w1264] -> w1249
          tunnel: w1248 -> [_ w1264]
          frame False {
            n250 = Get Variant Attribute(Variant=w1262, name=w1263, default value (empty Variant)=w1258, error in=w1260) -> (duplicate Variant=w1261:variant, value=w1257:i32, error out=w1259:errorcluster)  [unwired: 1 out]
            n251 = To Variant(anything=w1257) -> (Variant=w1256:variant)
          }
          frame True {
            n252 = Variant To Data(type=w1271, Variant=w1264) -> (data=w1266:i32)  [unwired: 1 in, 1 out]
            n253 = Set Variant Attribute(Variant=w1270, name=w1267, value=w1266, error in=w1268) -> (Variant out=w1269:variant, error out=w1265:errorcluster)  [unwired: 1 out]
          }
        }
      }
      frame "Data Information:Dataset Scaling Factor" {
        n254 = case shown="True" w1280 {
          tunnel: w1279 -> [w1288 w1292]
          tunnel: w1278 -> [w1287 w1295]
          tunnel: [w1286 w1294] -> w1277
          tunnel: w1276 -> [w1285 w1293]
          tunnel: [w1284 w1290] -> w1275
          tunnel: "Dataset Scaling Factor" -> [w1283 w1296]
          tunnel: [w1281 w1289] -> w1274
          tunnel: w1273 -> [_ w1289]
          frame False {
            n255 = Get Variant Attribute(Variant=w1287, name=w1288, default value (empty Variant)=w1283, error in=w1285) -> (duplicate Variant=w1286:variant, value=w1282:dbl, error out=w1284:errorcluster)  [unwired: 1 out]
            n256 = To Variant(anything=w1282) -> (Variant=w1281:variant)
          }
          frame True {
            n257 = Variant To Data(type=w1296, Variant=w1289) -> (data=w1291:dbl)  [unwired: 1 in, 1 out]
            n258 = Set Variant Attribute(Variant=w1295, name=w1292, value=w1291, error in=w1293) -> (Variant out=w1294:variant, error out=w1290:errorcluster)  [unwired: 1 out]
          }
        }
      }
      frame "Data Information:Macrotime Gate Separation" {
        n259 = case shown="True" w1305 {
          tunnel: w1304 -> [w1313 w1317]
          tunnel: w1303 -> [w1312 w1320]
          tunnel: [w1311 w1319] -> w1302
          tunnel: w1301 -> [w1310 w1318]
          tunnel: [w1309 w1315] -> w1300
          tunnel: "Mscrotime Gate Separation" -> [w1308 w1321]
          tunnel: [w1306 w1314] -> w1299
          tunnel: w1298 -> [_ w1314]
          frame False {
            n260 = Get Variant Attribute(Variant=w1312, name=w1313, default value (empty Variant)=w1308, error in=w1310) -> (duplicate Variant=w1311:variant, value=w1307:dbl[unit], error out=w1309:errorcluster)  [unwired: 1 out]
            n261 = To Variant(anything=w1307) -> (Variant=w1306:variant)
          }
          frame True {
            n262 = Variant To Data(type=w1321, Variant=w1314) -> (data=w1316:dbl[unit])  [unwired: 1 in, 1 out]
            n263 = Set Variant Attribute(Variant=w1320, name=w1317, value=w1316, error in=w1318) -> (Variant out=w1319:variant, error out=w1315:errorcluster)  [unwired: 1 out]
          }
        }
      }
      frame "Fluorescence Decay_Decay Pre-Processing:Reverse Gates" {
        n264 = case shown="True" w1330 {
          tunnel: w1329 -> [w1338 w1342]
          tunnel: w1328 -> [w1337 w1345]
          tunnel: [w1336 w1344] -> w1327
          tunnel: w1326 -> [w1335 w1343]
          tunnel: [w1334 w1340] -> w1325
          tunnel: "Reverse Gates" -> [w1333 w1346]
          tunnel: [w1331 w1339] -> w1324
          tunnel: w1323 -> [_ w1339]
          frame False {
            n265 = Get Variant Attribute(Variant=w1337, name=w1338, default value (empty Variant)=w1333, error in=w1335) -> (duplicate Variant=w1336:variant, value=w1332:bool, error out=w1334:errorcluster)  [unwired: 1 out]
            n266 = To Variant(anything=w1332) -> (Variant=w1331:variant)
          }
          frame True {
            n267 = Variant To Data(type=w1346, Variant=w1339) -> (data=w1341:bool)  [unwired: 1 in, 1 out]
            n268 = Set Variant Attribute(Variant=w1345, name=w1342, value=w1341, error in=w1343) -> (Variant out=w1344:variant, error out=w1340:errorcluster)  [unwired: 1 out]
          }
        }
      }
      frame "Fluorescence Decay_Decay Pre-Processing:Verbose Decay Pre-Processing" {
        n269 = case shown="True" w1355 {
          tunnel: w1354 -> [w1363 w1367]
          tunnel: w1353 -> [w1362 w1370]
          tunnel: [w1361 w1369] -> w1352
          tunnel: w1351 -> [w1360 w1368]
          tunnel: [w1359 w1365] -> w1350
          tunnel: "Verbose Decay Pre-Processing" -> [w1358 w1371]
          tunnel: [w1356 w1364] -> w1349
          tunnel: w1348 -> [_ w1364]
          frame False {
            n270 = Get Variant Attribute(Variant=w1362, name=w1363, default value (empty Variant)=w1358, error in=w1360) -> (duplicate Variant=w1361:variant, value=w1357:bool, error out=w1359:errorcluster)  [unwired: 1 out]
            n271 = To Variant(anything=w1357) -> (Variant=w1356:variant)
          }
          frame True {
            n272 = Variant To Data(type=w1371, Variant=w1364) -> (data=w1366:bool)  [unwired: 1 in, 1 out]
            n273 = Set Variant Attribute(Variant=w1370, name=w1367, value=w1366, error in=w1368) -> (Variant out=w1369:variant, error out=w1365:errorcluster)  [unwired: 1 out]
          }
        }
      }
      frame "Fluorescence Decay_Decay Pre-Processing:Use Decay Pre-Processing" {
        n274 = case shown="True" w1380 {
          tunnel: w1379 -> [w1388 w1392]
          tunnel: w1378 -> [w1387 w1395]
          tunnel: [w1386 w1394] -> w1377
          tunnel: w1376 -> [w1385 w1393]
          tunnel: [w1384 w1390] -> w1375
          tunnel: "Use Decay Pre-Processing" -> [w1383 w1396]
          tunnel: [w1381 w1389] -> w1374
          tunnel: w1373 -> [_ w1389]
          frame False {
            n275 = Get Variant Attribute(Variant=w1387, name=w1388, default value (empty Variant)=w1383, error in=w1385) -> (duplicate Variant=w1386:variant, value=w1382:bool, error out=w1384:errorcluster)  [unwired: 1 out]
            n276 = To Variant(anything=w1382) -> (Variant=w1381:variant)
          }
          frame True {
            n277 = Variant To Data(type=w1396, Variant=w1389) -> (data=w1391:bool)  [unwired: 1 in, 1 out]
            n278 = Set Variant Attribute(Variant=w1395, name=w1392, value=w1391, error in=w1393) -> (Variant out=w1394:variant, error out=w1390:errorcluster)  [unwired: 1 out]
          }
        }
      }
      frame "Fluorescence Decay_Decay Pre-Processing:Background Subtraction" {
        n279 = case shown="True" w1405 {
          tunnel: w1404 -> [w1413 w1417]
          tunnel: w1403 -> [w1412 w1420]
          tunnel: [w1411 w1419] -> w1402
          tunnel: w1401 -> [w1410 w1418]
          tunnel: [w1409 w1415] -> w1400
          tunnel: "Background Subtraction" -> [w1408 w1421]
          tunnel: [w1406 w1414] -> w1399
          tunnel: w1398 -> [_ w1414]
          frame False {
            n280 = Get Variant Attribute(Variant=w1412, name=w1413, default value (empty Variant)=w1408, error in=w1410) -> (duplicate Variant=w1411:variant, value=w1407:bool, error out=w1409:errorcluster)  [unwired: 1 out]
            n281 = To Variant(anything=w1407) -> (Variant=w1406:variant)
          }
          frame True {
            n282 = Variant To Data(type=w1421, Variant=w1414) -> (data=w1416:bool)  [unwired: 1 in, 1 out]
            n283 = Set Variant Attribute(Variant=w1420, name=w1417, value=w1416, error in=w1418) -> (Variant out=w1419:variant, error out=w1415:errorcluster)  [unwired: 1 out]
          }
        }
      }
      frame "Fluorescence Decay_Decay Pre-Processing:Background Definition Range" {
        n284 = case shown="True" w1430 {
          tunnel: w1429 -> [w1438 w1442]
          tunnel: w1428 -> [w1437 w1445]
          tunnel: [w1436 w1444] -> w1427
          tunnel: w1426 -> [w1435 w1443]
          tunnel: [w1434 w1440] -> w1425
          tunnel: "Background Definition Range" -> [w1433 w1446]
          tunnel: [w1431 w1439] -> w1424
          tunnel: w1423 -> [_ w1439]
          frame False {
            n285 = Get Variant Attribute(Variant=w1437, name=w1438, default value (empty Variant)=w1433, error in=w1435) -> (duplicate Variant=w1436:variant, value=w1432:T19, error out=w1434:errorcluster)  [unwired: 1 out]
            n286 = To Variant(anything=w1432) -> (Variant=w1431:variant)
          }
          frame True {
            n287 = Variant To Data(type=w1446, Variant=w1439) -> (data=w1441:T19)  [unwired: 1 in, 1 out]
            n288 = Set Variant Attribute(Variant=w1445, name=w1442, value=w1441, error in=w1443) -> (Variant out=w1444:variant, error out=w1440:errorcluster)  [unwired: 1 out]
          }
        }
      }
      frame "Fluorescence Decay_Decay Pre-Processing:Baseline Subtraction Method" {
        n289 = case shown="True" w1455 {
          tunnel: w1454 -> [w1463 w1467]
          tunnel: w1453 -> [w1462 w1470]
          tunnel: [w1461 w1469] -> w1452
          tunnel: w1451 -> [w1460 w1468]
          tunnel: [w1459 w1465] -> w1450
          tunnel: "Baseline Subtraction Method" -> [w1458 w1471]
          tunnel: [w1456 w1464] -> w1449
          tunnel: w1448 -> [_ w1464]
          frame False {
            n290 = Get Variant Attribute(Variant=w1462, name=w1463, default value (empty Variant)=w1458, error in=w1460) -> (duplicate Variant=w1461:variant, value=w1457:T18, error out=w1459:errorcluster)  [unwired: 1 out]
            n291 = To Variant(anything=w1457) -> (Variant=w1456:variant)
          }
          frame True {
            n292 = Variant To Data(type=w1471, Variant=w1464) -> (data=w1466:T18)  [unwired: 1 in, 1 out]
            n293 = Set Variant Attribute(Variant=w1470, name=w1467, value=w1466, error in=w1468) -> (Variant out=w1469:variant, error out=w1465:errorcluster)  [unwired: 1 out]
          }
        }
      }
      frame "Fluorescence Decay_Decay Pre-Processing:Decay Pre-Processing Operations Order" {
        n294 = case shown="True" w1481 {
          tunnel: w1480 -> [w1489 w1496]
          tunnel: w1479 -> [w1488 w1499]
          tunnel: [w1487 w1498] -> w1478
          tunnel: w1477 -> [w1486 w1497]
          tunnel: [w1485 w1495] -> w1476
          tunnel: "Decay Pre-Processing Operations Order" -> [w1484 w1500]
          tunnel: [w1482 w1494] -> w1475
          tunnel: w1474 -> [_ w1494]
          tunnel: w1472 -> [_ w1490]
          frame False {
            n295 = Get Variant Attribute(Variant=w1488, name=w1489, default value (empty Variant)=w1484, error in=w1486) -> (duplicate Variant=w1487:variant, value=w1483:string[], error out=w1485:errorcluster)  [unwired: 1 out]
            n296 = To Variant(anything=w1483) -> (Variant=w1482:variant)
          }
          frame True {
            n297 = Variant To Data(type=w1500, Variant=w1494) -> (data=w1492:string[])  [unwired: 1 in, 1 out]
            n298 = Array Size(array=w1492) -> (size(s)=w1491:i32)
            n299 = case shown="8" w1491 {
              tunnel: w1492 -> [w1501 _]
              tunnel: [w1501 w1502] -> w1493
              tunnel: w1490 -> [_ w1502]
              frame 8 {
              }
              frame 0, Default {
              }
            }
            n300 = Set Variant Attribute(Variant=w1499, name=w1496, value=w1493, error in=w1497) -> (Variant out=w1498:variant, error out=w1495:errorcluster)  [unwired: 1 out]
          }
        }
      }
      frame "Source Image:Image Pre-Processing Operations Order" {
        n301 = case shown="True" w1512 {
          tunnel: w1511 -> [w1520 w1527]
          tunnel: w1510 -> [w1519 w1530]
          tunnel: [w1518 w1529] -> w1509
          tunnel: w1508 -> [w1517 w1528]
          tunnel: [w1516 w1526] -> w1507
          tunnel: "Image Pre-Processing Operations Order" -> [w1515 w1531]
          tunnel: [w1513 w1525] -> w1506
          tunnel: w1505 -> [_ w1525]
          tunnel: w1503 -> [_ w1521]
          frame False {
            n302 = Get Variant Attribute(Variant=w1519, name=w1520, default value (empty Variant)=w1515, error in=w1517) -> (duplicate Variant=w1518:variant, value=w1514:string[], error out=w1516:errorcluster)  [unwired: 1 out]
            n303 = To Variant(anything=w1514) -> (Variant=w1513:variant)
          }
          frame True {
            n304 = Variant To Data(type=w1531, Variant=w1525) -> (data=w1523:string[])  [unwired: 1 in, 1 out]
            n305 = Array Size(array=w1523) -> (size(s)=w1522:i32)
            n306 = case shown="5, 6" w1522 {
              tunnel: w1523 -> [w1532 _]
              tunnel: [w1532 w1533] -> w1524
              tunnel: w1521 -> [_ w1533]
              frame 5, 6 {
              }
              frame 0, Default {
              }
            }
            n307 = Set Variant Attribute(Variant=w1530, name=w1527, value=w1524, error in=w1528) -> (Variant out=w1529:variant, error out=w1526:errorcluster)  [unwired: 1 out]
          }
        }
      }
      frame "Fluorescence Decay_Decay Pre-Processing:Smoothing Parameter" {
        n308 = case shown="True" w1542 {
          tunnel: w1541 -> [w1550 w1554]
          tunnel: w1540 -> [w1549 w1557]
          tunnel: [w1548 w1556] -> w1539
          tunnel: w1538 -> [w1547 w1555]
          tunnel: [w1546 w1552] -> w1537
          tunnel: "Smoothing Parameter" -> [w1545 w1558]
          tunnel: [w1543 w1551] -> w1536
          tunnel: w1535 -> [_ w1551]
          frame False {
            n309 = Get Variant Attribute(Variant=w1549, name=w1550, default value (empty Variant)=w1545, error in=w1547) -> (duplicate Variant=w1548:variant, value=w1544:dbl, error out=w1546:errorcluster)  [unwired: 1 out]
            n310 = To Variant(anything=w1544) -> (Variant=w1543:variant)
          }
          frame True {
            n311 = Variant To Data(type=w1558, Variant=w1551) -> (data=w1553:dbl)  [unwired: 1 in, 1 out]
            n312 = Set Variant Attribute(Variant=w1557, name=w1554, value=w1553, error in=w1555) -> (Variant out=w1556:variant, error out=w1552:errorcluster)  [unwired: 1 out]
          }
        }
      }
      frame "Fluorescence Decay_Decay Pre-Processing:Shift Decay" {
        n313 = case shown="True" w1567 {
          tunnel: w1566 -> [w1575 w1579]
          tunnel: w1565 -> [w1574 w1582]
          tunnel: [w1573 w1581] -> w1564
          tunnel: w1563 -> [w1572 w1580]
          tunnel: [w1571 w1577] -> w1562
          tunnel: "Shift Decay" -> [w1570 w1583]
          tunnel: [w1568 w1576] -> w1561
          tunnel: w1560 -> [_ w1576]
          frame False {
            n314 = Get Variant Attribute(Variant=w1574, name=w1575, default value (empty Variant)=w1570, error in=w1572) -> (duplicate Variant=w1573:variant, value=w1569:bool, error out=w1571:errorcluster)  [unwired: 1 out]
            n315 = To Variant(anything=w1569) -> (Variant=w1568:variant)
          }
          frame True {
            n316 = Variant To Data(type=w1583, Variant=w1576) -> (data=w1578:bool)  [unwired: 1 in, 1 out]
            n317 = Set Variant Attribute(Variant=w1582, name=w1579, value=w1578, error in=w1580) -> (Variant out=w1581:variant, error out=w1577:errorcluster)  [unwired: 1 out]
          }
        }
      }
      frame "Fluorescence Decay_Decay Pre-Processing:Decay Shift Parameters" {
        n318 = case shown="True" w1592 {
          tunnel: w1591 -> [w1600 w1604]
          tunnel: w1590 -> [w1599 w1607]
          tunnel: [w1598 w1606] -> w1589
          tunnel: w1588 -> [w1597 w1605]
          tunnel: [w1596 w1602] -> w1587
          tunnel: "Decay Shift Parameters" -> [w1595 w1608]
          tunnel: [w1593 w1601] -> w1586
          tunnel: w1585 -> [_ w1601]
          frame False {
            n319 = Get Variant Attribute(Variant=w1599, name=w1600, default value (empty Variant)=w1595, error in=w1597) -> (duplicate Variant=w1598:variant, value=w1594:T20, error out=w1596:errorcluster)  [unwired: 1 out]
            n320 = To Variant(anything=w1594) -> (Variant=w1593:variant)
          }
          frame True {
            n321 = Variant To Data(type=w1608, Variant=w1601) -> (data=w1603:T20)  [unwired: 1 in, 1 out]
            n322 = Set Variant Attribute(Variant=w1607, name=w1604, value=w1603, error in=w1605) -> (Variant out=w1606:variant, error out=w1602:errorcluster)  [unwired: 1 out]
          }
        }
      }
      frame "Fluorescence Decay_Decay Pre-Processing:Fold Decay" {
        n323 = case shown="True" w1617 {
          tunnel: w1616 -> [w1625 w1629]
          tunnel: w1615 -> [w1624 w1632]
          tunnel: [w1623 w1631] -> w1614
          tunnel: w1613 -> [w1622 w1630]
          tunnel: [w1621 w1627] -> w1612
          tunnel: "Fold Decay" -> [w1620 w1633]
          tunnel: [w1618 w1626] -> w1611
          tunnel: w1610 -> [_ w1626]
          frame False {
            n324 = Get Variant Attribute(Variant=w1624, name=w1625, default value (empty Variant)=w1620, error in=w1622) -> (duplicate Variant=w1623:variant, value=w1619:bool, error out=w1621:errorcluster)  [unwired: 1 out]
            n325 = To Variant(anything=w1619) -> (Variant=w1618:variant)
          }
          frame True {
            n326 = Variant To Data(type=w1633, Variant=w1626) -> (data=w1628:bool)  [unwired: 1 in, 1 out]
            n327 = Set Variant Attribute(Variant=w1632, name=w1629, value=w1628, error in=w1630) -> (Variant out=w1631:variant, error out=w1627:errorcluster)  [unwired: 1 out]
          }
        }
      }
      frame "Fluorescence Decay_Decay Pre-Processing:# Folds" {
        n328 = case shown="True" w1642 {
          tunnel: w1641 -> [w1650 w1654]
          tunnel: w1640 -> [w1649 w1657]
          tunnel: [w1648 w1656] -> w1639
          tunnel: w1638 -> [w1647 w1655]
          tunnel: [w1646 w1652] -> w1637
          tunnel: "# Folds" -> [w1645 w1658]
          tunnel: [w1643 w1651] -> w1636
          tunnel: w1635 -> [_ w1651]
          frame False {
            n329 = Get Variant Attribute(Variant=w1649, name=w1650, default value (empty Variant)=w1645, error in=w1647) -> (duplicate Variant=w1648:variant, value=w1644:u32, error out=w1646:errorcluster)  [unwired: 1 out]
            n330 = To Variant(anything=w1644) -> (Variant=w1643:variant)
          }
          frame True {
            n331 = Variant To Data(type=w1658, Variant=w1651) -> (data=w1653:u32)  [unwired: 1 in, 1 out]
            n332 = Set Variant Attribute(Variant=w1657, name=w1654, value=w1653, error in=w1655) -> (Variant out=w1656:variant, error out=w1652:errorcluster)  [unwired: 1 out]
          }
        }
      }
      frame "Fluorescence Decay_Decay Pre-Processing:1-Normalize Decay" {
        n333 = case shown="True" w1667 {
          tunnel: w1666 -> [w1675 w1679]
          tunnel: w1665 -> [w1674 w1682]
          tunnel: [w1673 w1681] -> w1664
          tunnel: w1663 -> [w1672 w1680]
          tunnel: [w1671 w1677] -> w1662
          tunnel: "1-Normalize Decay" -> [w1670 w1683]
          tunnel: [w1668 w1676] -> w1661
          tunnel: w1660 -> [_ w1676]
          frame False {
            n334 = Get Variant Attribute(Variant=w1674, name=w1675, default value (empty Variant)=w1670, error in=w1672) -> (duplicate Variant=w1673:variant, value=w1669:bool, error out=w1671:errorcluster)  [unwired: 1 out]
            n335 = To Variant(anything=w1669) -> (Variant=w1668:variant)
          }
          frame True {
            n336 = Variant To Data(type=w1683, Variant=w1676) -> (data=w1678:bool)  [unwired: 1 in, 1 out]
            n337 = Set Variant Attribute(Variant=w1682, name=w1679, value=w1678, error in=w1680) -> (Variant out=w1681:variant, error out=w1677:errorcluster)  [unwired: 1 out]
          }
        }
      }
      frame "Fluorescence Decay_Decay Pre-Processing:[0-1]-Normalize Decay" {
        n338 = case shown="True" w1692 {
          tunnel: w1691 -> [w1700 w1704]
          tunnel: w1690 -> [w1699 w1707]
          tunnel: [w1698 w1706] -> w1689
          tunnel: w1688 -> [w1697 w1705]
          tunnel: [w1696 w1702] -> w1687
          tunnel: "[0-1]-Normalize Decay" -> [w1695 w1708]
          tunnel: [w1693 w1701] -> w1686
          tunnel: w1685 -> [_ w1701]
          frame False {
            n339 = Get Variant Attribute(Variant=w1699, name=w1700, default value (empty Variant)=w1695, error in=w1697) -> (duplicate Variant=w1698:variant, value=w1694:bool, error out=w1696:errorcluster)  [unwired: 1 out]
            n340 = To Variant(anything=w1694) -> (Variant=w1693:variant)
          }
          frame True {
            n341 = Variant To Data(type=w1708, Variant=w1701) -> (data=w1703:bool)  [unwired: 1 in, 1 out]
            n342 = Set Variant Attribute(Variant=w1707, name=w1704, value=w1703, error in=w1705) -> (Variant out=w1706:variant, error out=w1702:errorcluster)  [unwired: 1 out]
          }
        }
      }
      frame "Fluorescence Decay_Decay Pre-Processing:Smoothen Decay" {
        n343 = case shown="True" w1717 {
          tunnel: w1716 -> [w1725 w1729]
          tunnel: w1715 -> [w1724 w1732]
          tunnel: [w1723 w1731] -> w1714
          tunnel: w1713 -> [w1722 w1730]
          tunnel: [w1721 w1727] -> w1712
          tunnel: "Smoothen Decay" -> [w1720 w1733]
          tunnel: [w1718 w1726] -> w1711
          tunnel: w1710 -> [_ w1726]
          frame False {
            n344 = Get Variant Attribute(Variant=w1724, name=w1725, default value (empty Variant)=w1720, error in=w1722) -> (duplicate Variant=w1723:variant, value=w1719:bool, error out=w1721:errorcluster)  [unwired: 1 out]
            n345 = To Variant(anything=w1719) -> (Variant=w1718:variant)
          }
          frame True {
            n346 = Variant To Data(type=w1733, Variant=w1726) -> (data=w1728:bool)  [unwired: 1 in, 1 out]
            n347 = Set Variant Attribute(Variant=w1732, name=w1729, value=w1728, error in=w1730) -> (Variant out=w1731:variant, error out=w1727:errorcluster)  [unwired: 1 out]
          }
        }
      }
      frame "Fluorescence Decay_Decay Pre-Processing:Extrapolate Decay" {
        n348 = case shown="True" w1742 {
          tunnel: w1741 -> [w1750 w1754]
          tunnel: w1740 -> [w1749 w1757]
          tunnel: [w1748 w1756] -> w1739
          tunnel: w1738 -> [w1747 w1755]
          tunnel: [w1746 w1752] -> w1737
          tunnel: "Extrapolate Decay" -> [w1745 w1758]
          tunnel: [w1743 w1751] -> w1736
          tunnel: w1735 -> [_ w1751]
          frame False {
            n349 = Get Variant Attribute(Variant=w1749, name=w1750, default value (empty Variant)=w1745, error in=w1747) -> (duplicate Variant=w1748:variant, value=w1744:bool, error out=w1746:errorcluster)  [unwired: 1 out]
            n350 = To Variant(anything=w1744) -> (Variant=w1743:variant)
          }
          frame True {
            n351 = Variant To Data(type=w1758, Variant=w1751) -> (data=w1753:bool)  [unwired: 1 in, 1 out]
            n352 = Set Variant Attribute(Variant=w1757, name=w1754, value=w1753, error in=w1755) -> (Variant out=w1756:variant, error out=w1752:errorcluster)  [unwired: 1 out]
          }
        }
      }
      frame "Fluorescence Decay_Decay Pre-Processing:Use Periodicity" {
        n353 = case shown="True" w1767 {
          tunnel: w1766 -> [w1775 w1779]
          tunnel: w1765 -> [w1774 w1782]
          tunnel: [w1773 w1781] -> w1764
          tunnel: w1763 -> [w1772 w1780]
          tunnel: [w1771 w1777] -> w1762
          tunnel: "Use Periodicity" -> [w1770 w1783]
          tunnel: [w1768 w1776] -> w1761
          tunnel: w1760 -> [_ w1776]
          frame False {
            n354 = Get Variant Attribute(Variant=w1774, name=w1775, default value (empty Variant)=w1770, error in=w1772) -> (duplicate Variant=w1773:variant, value=w1769:bool, error out=w1771:errorcluster)  [unwired: 1 out]
            n355 = To Variant(anything=w1769) -> (Variant=w1768:variant)
          }
          frame True {
            n356 = Variant To Data(type=w1783, Variant=w1776) -> (data=w1778:bool)  [unwired: 1 in, 1 out]
            n357 = Set Variant Attribute(Variant=w1782, name=w1779, value=w1778, error in=w1780) -> (Variant out=w1781:variant, error out=w1777:errorcluster)  [unwired: 1 out]
          }
        }
      }
      frame "Fluorescence Decay_Decay Pre-Processing:Use Cursors" {
        n358 = case shown="True" w1792 {
          tunnel: w1791 -> [w1800 w1804]
          tunnel: w1790 -> [w1799 w1807]
          tunnel: [w1798 w1806] -> w1789
          tunnel: w1788 -> [w1797 w1805]
          tunnel: [w1796 w1802] -> w1787
          tunnel: "Use Cursors" -> [w1795 w1808]
          tunnel: [w1793 w1801] -> w1786
          tunnel: w1785 -> [_ w1801]
          frame False {
            n359 = Get Variant Attribute(Variant=w1799, name=w1800, default value (empty Variant)=w1795, error in=w1797) -> (duplicate Variant=w1798:variant, value=w1794:bool, error out=w1796:errorcluster)  [unwired: 1 out]
            n360 = To Variant(anything=w1794) -> (Variant=w1793:variant)
          }
          frame True {
            n361 = Variant To Data(type=w1808, Variant=w1801) -> (data=w1803:bool)  [unwired: 1 in, 1 out]
            n362 = Set Variant Attribute(Variant=w1807, name=w1804, value=w1803, error in=w1805) -> (Variant out=w1806:variant, error out=w1802:errorcluster)  [unwired: 1 out]
          }
        }
      }
      frame "Fluorescence Decay_Decay Pre-Processing:Tail Fraction" {
        n363 = case shown="True" w1817 {
          tunnel: w1816 -> [w1825 w1829]
          tunnel: w1815 -> [w1824 w1832]
          tunnel: [w1823 w1831] -> w1814
          tunnel: w1813 -> [w1822 w1830]
          tunnel: [w1821 w1827] -> w1812
          tunnel: "Tail Fraction" -> [w1820 w1833]
          tunnel: [w1818 w1826] -> w1811
          tunnel: w1810 -> [_ w1826]
          frame False {
            n364 = Get Variant Attribute(Variant=w1824, name=w1825, default value (empty Variant)=w1820, error in=w1822) -> (duplicate Variant=w1823:variant, value=w1819:dbl, error out=w1821:errorcluster)  [unwired: 1 out]
            n365 = To Variant(anything=w1819) -> (Variant=w1818:variant)
          }
          frame True {
            n366 = Variant To Data(type=w1833, Variant=w1826) -> (data=w1828:dbl)  [unwired: 1 in, 1 out]
            n367 = Set Variant Attribute(Variant=w1832, name=w1829, value=w1828, error in=w1830) -> (Variant out=w1831:variant, error out=w1827:errorcluster)  [unwired: 1 out]
          }
        }
      }
      frame "Fluorescence Decay_Decay Pre-Processing:Head Fraction" {
        n368 = case shown="True" w1842 {
          tunnel: w1841 -> [w1850 w1854]
          tunnel: w1840 -> [w1849 w1857]
          tunnel: [w1848 w1856] -> w1839
          tunnel: w1838 -> [w1847 w1855]
          tunnel: [w1846 w1852] -> w1837
          tunnel: "Head Fraction" -> [w1845 w1858]
          tunnel: [w1843 w1851] -> w1836
          tunnel: w1835 -> [_ w1851]
          frame False {
            n369 = Get Variant Attribute(Variant=w1849, name=w1850, default value (empty Variant)=w1845, error in=w1847) -> (duplicate Variant=w1848:variant, value=w1844:dbl, error out=w1846:errorcluster)  [unwired: 1 out]
            n370 = To Variant(anything=w1844) -> (Variant=w1843:variant)
          }
          frame True {
            n371 = Variant To Data(type=w1858, Variant=w1851) -> (data=w1853:dbl)  [unwired: 1 in, 1 out]
            n372 = Set Variant Attribute(Variant=w1857, name=w1854, value=w1853, error in=w1855) -> (Variant out=w1856:variant, error out=w1852:errorcluster)  [unwired: 1 out]
          }
        }
      }
      frame "Fluorescence Decay_Decay Pre-Processing:Additional Points" {
        n373 = case shown="True" w1867 {
          tunnel: w1866 -> [w1875 w1879]
          tunnel: w1865 -> [w1874 w1882]
          tunnel: [w1873 w1881] -> w1864
          tunnel: w1863 -> [w1872 w1880]
          tunnel: [w1871 w1877] -> w1862
          tunnel: "Additional Points" -> [w1870 w1883]
          tunnel: [w1868 w1876] -> w1861
          tunnel: w1860 -> [_ w1876]
          frame False {
            n374 = Get Variant Attribute(Variant=w1874, name=w1875, default value (empty Variant)=w1870, error in=w1872) -> (duplicate Variant=w1873:variant, value=w1869:u32, error out=w1871:errorcluster)  [unwired: 1 out]
            n375 = To Variant(anything=w1869) -> (Variant=w1868:variant)
          }
          frame True {
            n376 = Variant To Data(type=w1883, Variant=w1876) -> (data=w1878:u32)  [unwired: 1 in, 1 out]
            n377 = Set Variant Attribute(Variant=w1882, name=w1879, value=w1878, error in=w1880) -> (Variant out=w1881:variant, error out=w1877:errorcluster)  [unwired: 1 out]
          }
        }
      }
      frame "Fluorescence Decay_Decay Pre-Processing:Straighten Decay" {
        n378 = case shown="True" w1892 {
          tunnel: w1891 -> [w1900 w1904]
          tunnel: w1890 -> [w1899 w1907]
          tunnel: [w1898 w1906] -> w1889
          tunnel: w1888 -> [w1897 w1905]
          tunnel: [w1896 w1902] -> w1887
          tunnel: "Straighten Decay" -> [w1895 w1908]
          tunnel: [w1893 w1901] -> w1886
          tunnel: w1885 -> [_ w1901]
          frame False {
            n379 = Get Variant Attribute(Variant=w1899, name=w1900, default value (empty Variant)=w1895, error in=w1897) -> (duplicate Variant=w1898:variant, value=w1894:bool, error out=w1896:errorcluster)  [unwired: 1 out]
            n380 = To Variant(anything=w1894) -> (Variant=w1893:variant)
          }
          frame True {
            n381 = Variant To Data(type=w1908, Variant=w1901) -> (data=w1903:bool)  [unwired: 1 in, 1 out]
            n382 = Set Variant Attribute(Variant=w1907, name=w1904, value=w1903, error in=w1905) -> (Variant out=w1906:variant, error out=w1902:errorcluster)  [unwired: 1 out]
          }
        }
      }
      frame "Fluorescence Decay_Decay Pre-Processing:Constant Background" {
        n383 = case shown="True" w1917 {
          tunnel: w1916 -> [w1925 w1929]
          tunnel: w1915 -> [w1924 w1932]
          tunnel: [w1923 w1931] -> w1914
          tunnel: w1913 -> [w1922 w1930]
          tunnel: [w1921 w1927] -> w1912
          tunnel: "Constant Background" -> [w1920 w1933]
          tunnel: [w1918 w1926] -> w1911
          tunnel: w1910 -> [_ w1926]
          frame False {
            n384 = Get Variant Attribute(Variant=w1924, name=w1925, default value (empty Variant)=w1920, error in=w1922) -> (duplicate Variant=w1923:variant, value=w1919:dbl, error out=w1921:errorcluster)  [unwired: 1 out]
            n385 = To Variant(anything=w1919) -> (Variant=w1918:variant)
          }
          frame True {
            n386 = Variant To Data(type=w1933, Variant=w1926) -> (data=w1928:dbl)  [unwired: 1 in, 1 out]
            n387 = Set Variant Attribute(Variant=w1932, name=w1929, value=w1928, error in=w1930) -> (Variant out=w1931:variant, error out=w1927:errorcluster)  [unwired: 1 out]
          }
        }
      }
      frame "Fluorescence Decay_Decay Pre-Processing:Pixel-Normalize Decay" {
        n388 = case shown="True" w1942 {
          tunnel: w1941 -> [w1950 w1954]
          tunnel: w1940 -> [w1949 w1957]
          tunnel: [w1948 w1956] -> w1939
          tunnel: w1938 -> [w1947 w1955]
          tunnel: [w1946 w1952] -> w1937
          tunnel: "Pixel-Normalize Decay" -> [w1945 w1958]
          tunnel: [w1943 w1951] -> w1936
          tunnel: w1935 -> [_ w1951]
          frame False {
            n389 = Get Variant Attribute(Variant=w1949, name=w1950, default value (empty Variant)=w1945, error in=w1947) -> (duplicate Variant=w1948:variant, value=w1944:bool, error out=w1946:errorcluster)  [unwired: 1 out]
            n390 = To Variant(anything=w1944) -> (Variant=w1943:variant)
          }
          frame True {
            n391 = Variant To Data(type=w1958, Variant=w1951) -> (data=w1953:bool)  [unwired: 1 in, 1 out]
            n392 = Set Variant Attribute(Variant=w1957, name=w1954, value=w1953, error in=w1955) -> (Variant out=w1956:variant, error out=w1952:errorcluster)  [unwired: 1 out]
          }
        }
      }
      frame "Fluorescence Decay_Advanced Analysis:Extract IRF instead of Decay" {
        n393 = case shown="True" w1967 {
          tunnel: w1966 -> [w1975 w1979]
          tunnel: w1965 -> [w1974 w1982]
          tunnel: [w1973 w1981] -> w1964
          tunnel: w1963 -> [w1972 w1980]
          tunnel: [w1971 w1977] -> w1962
          tunnel: "Extract IRF instead of Decay" -> [w1970 w1983]
          tunnel: [w1968 w1976] -> w1961
          tunnel: w1960 -> [_ w1976]
          frame False {
            n394 = Get Variant Attribute(Variant=w1974, name=w1975, default value (empty Variant)=w1970, error in=w1972) -> (duplicate Variant=w1973:variant, value=w1969:bool, error out=w1971:errorcluster)  [unwired: 1 out]
            n395 = To Variant(anything=w1969) -> (Variant=w1968:variant)
          }
          frame True {
            n396 = Variant To Data(type=w1983, Variant=w1976) -> (data=w1978:bool)  [unwired: 1 in, 1 out]
            n397 = Set Variant Attribute(Variant=w1982, name=w1979, value=w1978, error in=w1980) -> (Variant out=w1981:variant, error out=w1977:errorcluster)  [unwired: 1 out]
          }
        }
      }
      frame "Fluorescence Decay_Advanced Analysis:IRF Extraction Options" {
        n398 = case shown="True" w1992 {
          tunnel: w1991 -> [w2000 w2004]
          tunnel: w1990 -> [w1999 w2007]
          tunnel: [w1998 w2006] -> w1989
          tunnel: w1988 -> [w1997 w2005]
          tunnel: [w1996 w2002] -> w1987
          tunnel: "Time Constant for IRF Extraction" -> [w1995 w2008]
          tunnel: [w1993 w2001] -> w1986
          tunnel: w1985 -> [_ w2001]
          frame False {
            n399 = Get Variant Attribute(Variant=w1999, name=w2000, default value (empty Variant)=w1995, error in=w1997) -> (duplicate Variant=w1998:variant, value=w1994:T26, error out=w1996:errorcluster)  [unwired: 1 out]
            n400 = To Variant(anything=w1994) -> (Variant=w1993:variant)
          }
          frame True {
            n401 = Variant To Data(type=w2008, Variant=w2001) -> (data=w2003:T26)  [unwired: 1 in, 1 out]
            n402 = Set Variant Attribute(Variant=w2007, name=w2004, value=w2003, error in=w2005) -> (Variant out=w2006:variant, error out=w2002:errorcluster)  [unwired: 1 out]
          }
        }
      }
      frame "Fluorescence Decay_Advanced Analysis:IRF Optimization Options" {
        n403 = case shown="True" w2017 {
          tunnel: w2016 -> [w2025 w2029]
          tunnel: w2015 -> [w2024 w2032]
          tunnel: [w2023 w2031] -> w2014
          tunnel: w2013 -> [w2022 w2030]
          tunnel: [w2021 w2027] -> w2012
          tunnel: "IRF Optimization Options" -> [w2020 w2033]
          tunnel: [w2018 w2026] -> w2011
          tunnel: w2010 -> [_ w2026]
          frame False {
            n404 = Get Variant Attribute(Variant=w2024, name=w2025, default value (empty Variant)=w2020, error in=w2022) -> (duplicate Variant=w2023:variant, value=w2019:T30, error out=w2021:errorcluster)  [unwired: 1 out]
            n405 = To Variant(anything=w2019) -> (Variant=w2018:variant)
          }
          frame True {
            n406 = Variant To Data(type=w2033, Variant=w2026) -> (data=w2028:T30)  [unwired: 1 in, 1 out]
            n407 = Set Variant Attribute(Variant=w2032, name=w2029, value=w2028, error in=w2030) -> (Variant out=w2031:variant, error out=w2027:errorcluster)  [unwired: 1 out]
          }
        }
      }
      frame "Fluorescence Decay_Advanced Analysis:Square Pulse Options" {
        n408 = case shown="True" w2042 {
          tunnel: w2041 -> [w2050 w2054]
          tunnel: w2040 -> [w2049 w2057]
          tunnel: [w2048 w2056] -> w2039
          tunnel: w2038 -> [w2047 w2055]
          tunnel: [w2046 w2052] -> w2037
          tunnel: "Square Pulse Options" -> [w2045 w2058]
          tunnel: [w2043 w2051] -> w2036
          tunnel: w2035 -> [_ w2051]
          frame False {
            n409 = Get Variant Attribute(Variant=w2049, name=w2050, default value (empty Variant)=w2045, error in=w2047) -> (duplicate Variant=w2048:variant, value=w2044:T23, error out=w2046:errorcluster)  [unwired: 1 out]
            n410 = To Variant(anything=w2044) -> (Variant=w2043:variant)
          }
          frame True {
            n411 = Variant To Data(type=w2058, Variant=w2051) -> (data=w2053:T23)  [unwired: 1 in, 1 out]
            n412 = Set Variant Attribute(Variant=w2057, name=w2054, value=w2053, error in=w2055) -> (Variant out=w2056:variant, error out=w2052:errorcluster)  [unwired: 1 out]
          }
        }
      }
      frame "Fluorescence Decay_Advanced Analysis:IRF Order" {
        n413 = case shown="True" w2067 {
          tunnel: w2066 -> [w2075 w2079]
          tunnel: w2065 -> [w2074 w2082]
          tunnel: [w2073 w2081] -> w2064
          tunnel: w2063 -> [w2072 w2080]
          tunnel: [w2071 w2077] -> w2062
          tunnel: "IRF order" -> [w2070 w2083]
          tunnel: [w2068 w2076] -> w2061
          tunnel: w2060 -> [_ w2076]
          frame False {
            n414 = Get Variant Attribute(Variant=w2074, name=w2075, default value (empty Variant)=w2070, error in=w2072) -> (duplicate Variant=w2073:variant, value=w2069:i32, error out=w2071:errorcluster)  [unwired: 1 out]
            n415 = To Variant(anything=w2069) -> (Variant=w2068:variant)
          }
          frame True {
            n416 = Variant To Data(type=w2083, Variant=w2076) -> (data=w2078:i32)  [unwired: 1 in, 1 out]
            n417 = Set Variant Attribute(Variant=w2082, name=w2079, value=w2078, error in=w2080) -> (Variant out=w2081:variant, error out=w2077:errorcluster)  [unwired: 1 out]
          }
        }
      }
      frame "Fluorescence Decay_Advanced Analysis:IRF Time Constants" {
        n418 = case shown="True" w2092 {
          tunnel: w2091 -> [w2101 w2106]
          tunnel: w2090 -> [w2100 w2109]
          tunnel: [w2099 w2108] -> w2089
          tunnel: w2088 -> [w2098 w2107]
          tunnel: [w2097 w2104] -> w2087
          tunnel: "IRF Time Constants" -> [w2096 w2110]
          tunnel: [w2094 w2103] -> w2086
          tunnel: w2085 -> [_ w2103]
          tunnel: [w2093 w2102] -> _
          frame False {
            n419 = Get Variant Attribute(Variant=w2100, name=w2101, default value (empty Variant)=w2096, error in=w2098) -> (duplicate Variant=w2099:variant, found=w2093:bool, value=w2095:dbl[], error out=w2097:errorcluster)
            n420 = To Variant(anything=w2095) -> (Variant=w2094:variant)
          }
          frame True {
            n421 = Variant To Data(type=w2110, Variant=w2103) -> (data=w2105:dbl[])  [unwired: 1 in, 1 out]
            n422 = Set Variant Attribute(Variant=w2109, name=w2106, value=w2105, error in=w2107) -> (Variant out=w2108:variant, replaced=w2102:bool, error out=w2104:errorcluster)
          }
        }
      }
      frame "Fluorescence Decay_Advanced Analysis:Wavelet Analysis Options" {
        n423 = case shown="True" w2119 {
          tunnel: w2118 -> [w2127 w2131]
          tunnel: w2117 -> [w2126 w2134]
          tunnel: [w2125 w2133] -> w2116
          tunnel: w2115 -> [w2124 w2132]
          tunnel: [w2123 w2129] -> w2114
          tunnel: "Wavelet Analysis Options" -> [w2122 w2135]
          tunnel: [w2120 w2128] -> w2113
          tunnel: w2112 -> [_ w2128]
          frame False {
            n424 = Get Variant Attribute(Variant=w2126, name=w2127, default value (empty Variant)=w2122, error in=w2124) -> (duplicate Variant=w2125:variant, value=w2121:T25, error out=w2123:errorcluster)  [unwired: 1 out]
            n425 = To Variant(anything=w2121) -> (Variant=w2120:variant)
          }
          frame True {
            n426 = Variant To Data(type=w2135, Variant=w2128) -> (data=w2130:T25)  [unwired: 1 in, 1 out]
            n427 = Set Variant Attribute(Variant=w2134, name=w2131, value=w2130, error in=w2132) -> (Variant out=w2133:variant, error out=w2129:errorcluster)  [unwired: 1 out]
          }
        }
      }
      frame "Fluorescence Decay_Advanced Analysis:Average Lifetime Options" {
        n428 = case shown="True" w2144 {
          tunnel: w2143 -> [w2152 w2156]
          tunnel: w2142 -> [w2151 w2159]
          tunnel: [w2150 w2158] -> w2141
          tunnel: w2140 -> [w2149 w2157]
          tunnel: [w2148 w2154] -> w2139
          tunnel: "Average Lifetime Options" -> [w2147 w2160]
          tunnel: [w2145 w2153] -> w2138
          tunnel: w2137 -> [_ w2153]
          frame False {
            n429 = Get Variant Attribute(Variant=w2151, name=w2152, default value (empty Variant)=w2147, error in=w2149) -> (duplicate Variant=w2150:variant, value=w2146:T22, error out=w2148:errorcluster)  [unwired: 1 out]
            n430 = To Variant(anything=w2146) -> (Variant=w2145:variant)
          }
          frame True {
            n431 = Variant To Data(type=w2160, Variant=w2153) -> (data=w2155:T22)  [unwired: 1 in, 1 out]
            n432 = Set Variant Attribute(Variant=w2159, name=w2156, value=w2155, error in=w2157) -> (Variant out=w2158:variant, error out=w2154:errorcluster)  [unwired: 1 out]
          }
        }
      }
      frame "Fluorescence Decay_Fit Options:Fit Options" {
        n433 = case shown="True" w2169 {
          tunnel: w2168 -> [w2177 w2181]
          tunnel: w2167 -> [w2176 w2184]
          tunnel: [w2175 w2183] -> w2166
          tunnel: w2165 -> [w2174 w2182]
          tunnel: [w2173 w2179] -> w2164
          tunnel: "Fit Options" -> [w2172 w2185]
          tunnel: [w2170 w2178] -> w2163
          tunnel: w2162 -> [_ w2178]
          frame False {
            n434 = Get Variant Attribute(Variant=w2176, name=w2177, default value (empty Variant)=w2172, error in=w2174) -> (duplicate Variant=w2175:variant, value=w2171:T32, error out=w2173:errorcluster)  [unwired: 1 out]
            n435 = To Variant(anything=w2171) -> (Variant=w2170:variant)
          }
          frame True {
            n436 = Variant To Data(type=w2185, Variant=w2178) -> (data=w2180:T32)  [unwired: 1 in, 1 out]
            n437 = Set Variant Attribute(Variant=w2184, name=w2181, value=w2180, error in=w2182) -> (Variant out=w2183:variant, error out=w2179:errorcluster)  [unwired: 1 out]
          }
        }
      }
      frame "Fluorescence Decay_Fit Options:Use Legacy Fitting Approach" {
        n438 = case shown="True" w2194 {
          tunnel: w2193 -> [w2202 w2206]
          tunnel: w2192 -> [w2201 w2209]
          tunnel: [w2200 w2208] -> w2191
          tunnel: w2190 -> [w2199 w2207]
          tunnel: [w2198 w2204] -> w2189
          tunnel: "Use Legagy Fitting Approach" -> [w2197 w2210]
          tunnel: [w2195 w2203] -> w2188
          tunnel: w2187 -> [_ w2203]
          frame False {
            n439 = Get Variant Attribute(Variant=w2201, name=w2202, default value (empty Variant)=w2197, error in=w2199) -> (duplicate Variant=w2200:variant, value=w2196:bool, error out=w2198:errorcluster)  [unwired: 1 out]
            n440 = To Variant(anything=w2196) -> (Variant=w2195:variant)
          }
          frame True {
            n441 = Variant To Data(type=w2210, Variant=w2203) -> (data=w2205:bool)  [unwired: 1 in, 1 out]
            n442 = Set Variant Attribute(Variant=w2209, name=w2206, value=w2205, error in=w2207) -> (Variant out=w2208:variant, error out=w2204:errorcluster)  [unwired: 1 out]
          }
        }
      }
      frame "Fluorescence Decay_Fit Options:Use Data Information Laser Period" {
        n443 = case shown="True" w2219 {
          tunnel: w2218 -> [w2227 w2231]
          tunnel: w2217 -> [w2226 w2234]
          tunnel: [w2225 w2233] -> w2216
          tunnel: w2215 -> [w2224 w2232]
          tunnel: [w2223 w2229] -> w2214
          tunnel: "Use Data Information Laser Period" -> [w2222 w2235]
          tunnel: [w2220 w2228] -> w2213
          tunnel: w2212 -> [_ w2228]
          frame False {
            n444 = Get Variant Attribute(Variant=w2226, name=w2227, default value (empty Variant)=w2222, error in=w2224) -> (duplicate Variant=w2225:variant, value=w2221:bool, error out=w2223:errorcluster)  [unwired: 1 out]
            n445 = To Variant(anything=w2221) -> (Variant=w2220:variant)
          }
          frame True {
            n446 = Variant To Data(type=w2235, Variant=w2228) -> (data=w2230:bool)  [unwired: 1 in, 1 out]
            n447 = Set Variant Attribute(Variant=w2234, name=w2231, value=w2230, error in=w2232) -> (Variant out=w2233:variant, error out=w2229:errorcluster)  [unwired: 1 out]
          }
        }
      }
      frame "Fluorescence Decay_Fit Parameters:Displayed Fit Parameters" {
        n448 = case shown="True" w2244 {
          tunnel: w2243 -> [w2252 w2256]
          tunnel: w2242 -> [w2251 w2259]
          tunnel: [w2250 w2258] -> w2241
          tunnel: w2240 -> [w2249 w2257]
          tunnel: [w2248 w2254] -> w2239
          tunnel: "Displayed Fit Parameters" -> [w2247 w2260]
          tunnel: [w2245 w2253] -> w2238
          tunnel: w2237 -> [_ w2253]
          frame False {
            n449 = Get Variant Attribute(Variant=w2251, name=w2252, default value (empty Variant)=w2247, error in=w2249) -> (duplicate Variant=w2250:variant, value=w2246:T43[], error out=w2248:errorcluster)  [unwired: 1 out]
            n450 = To Variant(anything=w2246) -> (Variant=w2245:variant)
          }
          frame True {
            n451 = Variant To Data(type=w2260, Variant=w2253) -> (data=w2255:T43[])  [unwired: 1 in, 1 out]
            n452 = Set Variant Attribute(Variant=w2259, name=w2256, value=w2255, error in=w2257) -> (Variant out=w2258:variant, error out=w2254:errorcluster)  [unwired: 1 out]
          }
        }
      }
      frame "Fluorescence Decay_Fit Parameters:Fit Parameter Constraints" {
        n453 = case shown="True" w2269 {
          tunnel: w2268 -> [w2277 w2281]
          tunnel: w2267 -> [w2276 w2284]
          tunnel: [w2275 w2283] -> w2266
          tunnel: w2265 -> [w2274 w2282]
          tunnel: [w2273 w2279] -> w2264
          tunnel: "Fit Parameter Constraints" -> [w2272 w2285]
          tunnel: [w2270 w2278] -> w2263
          tunnel: w2262 -> [_ w2278]
          frame False {
            n454 = Get Variant Attribute(Variant=w2276, name=w2277, default value (empty Variant)=w2272, error in=w2274) -> (duplicate Variant=w2275:variant, value=w2271:T42[], error out=w2273:errorcluster)  [unwired: 1 out]
            n455 = To Variant(anything=w2271) -> (Variant=w2270:variant)
          }
          frame True {
            n456 = Variant To Data(type=w2285, Variant=w2278) -> (data=w2280:T42[])  [unwired: 1 in, 1 out]
            n457 = Set Variant Attribute(Variant=w2284, name=w2281, value=w2280, error in=w2282) -> (Variant out=w2283:variant, error out=w2279:errorcluster)  [unwired: 1 out]
          }
        }
      }
      frame "Fluorescence Decay_Fit Parameters:Export Tabulated Results" {
        n458 = case shown="True" w2294 {
          tunnel: w2293 -> [w2302 w2306]
          tunnel: w2292 -> [w2301 w2309]
          tunnel: [w2300 w2308] -> w2291
          tunnel: w2290 -> [w2299 w2307]
          tunnel: [w2298 w2304] -> w2289
          tunnel: "Export Tabulated Results" -> [w2297 w2310]
          tunnel: [w2295 w2303] -> w2288
          tunnel: w2287 -> [_ w2303]
          frame False {
            n459 = Get Variant Attribute(Variant=w2301, name=w2302, default value (empty Variant)=w2297, error in=w2299) -> (duplicate Variant=w2300:variant, value=w2296:bool, error out=w2298:errorcluster)  [unwired: 1 out]
            n460 = To Variant(anything=w2296) -> (Variant=w2295:variant)
          }
          frame True {
            n461 = Variant To Data(type=w2310, Variant=w2303) -> (data=w2305:bool)  [unwired: 1 in, 1 out]
            n462 = Set Variant Attribute(Variant=w2309, name=w2306, value=w2305, error in=w2307) -> (Variant out=w2308:variant, error out=w2304:errorcluster)  [unwired: 1 out]
          }
        }
      }
      frame "Fluorescence Decay_Fit Parameters:MLE Baseline Offset Type" {
        n463 = case shown="True" w2319 {
          tunnel: w2318 -> [w2327 w2331]
          tunnel: w2317 -> [w2326 w2334]
          tunnel: [w2325 w2333] -> w2316
          tunnel: w2315 -> [w2324 w2332]
          tunnel: [w2323 w2329] -> w2314
          tunnel: "MLE Baseline Offset Type" -> [w2322 w2335]
          tunnel: [w2320 w2328] -> w2313
          tunnel: w2312 -> [_ w2328]
          frame False {
            n464 = Get Variant Attribute(Variant=w2326, name=w2327, default value (empty Variant)=w2322, error in=w2324) -> (duplicate Variant=w2325:variant, value=w2321:T39, error out=w2323:errorcluster)  [unwired: 1 out]
            n465 = To Variant(anything=w2321) -> (Variant=w2320:variant)
          }
          frame True {
            n466 = Variant To Data(type=w2335, Variant=w2328) -> (data=w2330:T39)  [unwired: 1 in, 1 out]
            n467 = Set Variant Attribute(Variant=w2334, name=w2331, value=w2330, error in=w2332) -> (Variant out=w2333:variant, error out=w2329:errorcluster)  [unwired: 1 out]
          }
        }
      }
      frame "Fluorescence Decay_Fit Parameters:MLE Baseline Offset" {
        n468 = case shown="True" w2344 {
          tunnel: w2343 -> [w2352 w2356]
          tunnel: w2342 -> [w2351 w2359]
          tunnel: [w2350 w2358] -> w2341
          tunnel: w2340 -> [w2349 w2357]
          tunnel: [w2348 w2354] -> w2339
          tunnel: "MLE Baseline Offset" -> [w2347 w2360]
          tunnel: [w2345 w2353] -> w2338
          tunnel: w2337 -> [_ w2353]
          frame False {
            n469 = Get Variant Attribute(Variant=w2351, name=w2352, default value (empty Variant)=w2347, error in=w2349) -> (duplicate Variant=w2350:variant, value=w2346:dbl, error out=w2348:errorcluster)  [unwired: 1 out]
            n470 = To Variant(anything=w2346) -> (Variant=w2345:variant)
          }
          frame True {
            n471 = Variant To Data(type=w2360, Variant=w2353) -> (data=w2355:dbl)  [unwired: 1 in, 1 out]
            n472 = Set Variant Attribute(Variant=w2359, name=w2356, value=w2355, error in=w2357) -> (Variant out=w2358:variant, error out=w2354:errorcluster)  [unwired: 1 out]
          }
        }
      }
      frame "Fluorescence Decay_Fit Parameters:Guess Parameter Names" {
        n473 = case shown="True" w2369 {
          tunnel: w2368 -> [w2377 w2381]
          tunnel: w2367 -> [w2376 w2384]
          tunnel: [w2375 w2383] -> w2366
          tunnel: w2365 -> [w2374 w2382]
          tunnel: [w2373 w2379] -> w2364
          tunnel: "Guess Parameters Names" -> [w2372 w2385]
          tunnel: [w2370 w2378] -> w2363
          tunnel: w2362 -> [_ w2378]
          frame False {
            n474 = Get Variant Attribute(Variant=w2376, name=w2377, default value (empty Variant)=w2372, error in=w2374) -> (duplicate Variant=w2375:variant, value=w2371:T41[], error out=w2373:errorcluster)  [unwired: 1 out]
            n475 = To Variant(anything=w2371) -> (Variant=w2370:variant)
          }
          frame True {
            n476 = Variant To Data(type=w2385, Variant=w2378) -> (data=w2380:T41[])  [unwired: 1 in, 1 out]
            n477 = Set Variant Attribute(Variant=w2384, name=w2381, value=w2380, error in=w2382) -> (Variant out=w2383:variant, error out=w2379:errorcluster)  [unwired: 1 out]
          }
        }
      }
      frame "Fluorescence Decay_Fit Parameters:Guess Parameter Values" {
        n478 = case shown="True" w2394 {
          tunnel: w2393 -> [w2402 w2406]
          tunnel: w2392 -> [w2401 w2409]
          tunnel: [w2400 w2408] -> w2391
          tunnel: w2390 -> [w2399 w2407]
          tunnel: [w2398 w2404] -> w2389
          tunnel: "Guess Parameter Values" -> [w2397 w2410]
          tunnel: [w2395 w2403] -> w2388
          tunnel: w2387 -> [_ w2403]
          frame False {
            n479 = Get Variant Attribute(Variant=w2401, name=w2402, default value (empty Variant)=w2397, error in=w2399) -> (duplicate Variant=w2400:variant, value=w2396:dbl[], error out=w2398:errorcluster)  [unwired: 1 out]
            n480 = To Variant(anything=w2396) -> (Variant=w2395:variant)
          }
          frame True {
            n481 = Variant To Data(type=w2410, Variant=w2403) -> (data=w2405:dbl[])  [unwired: 1 in, 1 out]
            n482 = Set Variant Attribute(Variant=w2409, name=w2406, value=w2405, error in=w2407) -> (Variant out=w2408:variant, error out=w2404:errorcluster)  [unwired: 1 out]
          }
        }
      }
      frame "Fluorescence Decay_Fit Parameters:Guess Parameters Options" {
        n483 = case shown="True" w2419 {
          tunnel: w2418 -> [w2427 w2431]
          tunnel: w2417 -> [w2426 w2434]
          tunnel: [w2425 w2433] -> w2416
          tunnel: w2415 -> [w2424 w2432]
          tunnel: [w2423 w2429] -> w2414
          tunnel: "Guess Parameters Options" -> [w2422 w2435]
          tunnel: [w2420 w2428] -> w2413
          tunnel: w2412 -> [_ w2428]
          frame False {
            n484 = Get Variant Attribute(Variant=w2426, name=w2427, default value (empty Variant)=w2422, error in=w2424) -> (duplicate Variant=w2425:variant, value=w2421:T40, error out=w2423:errorcluster)  [unwired: 1 out]
            n485 = To Variant(anything=w2421) -> (Variant=w2420:variant)
          }
          frame True {
            n486 = Variant To Data(type=w2435, Variant=w2428) -> (data=w2430:T40)  [unwired: 1 in, 1 out]
            n487 = Set Variant Attribute(Variant=w2434, name=w2431, value=w2430, error in=w2432) -> (Variant out=w2433:variant, error out=w2429:errorcluster)  [unwired: 1 out]
          }
        }
      }
      frame "Fluorescence Decay_Styles:Show Last Decay Only" {
        n488 = case shown="True" w2444 {
          tunnel: w2443 -> [w2452 w2456]
          tunnel: w2442 -> [w2451 w2459]
          tunnel: [w2450 w2458] -> w2441
          tunnel: w2440 -> [w2449 w2457]
          tunnel: [w2448 w2454] -> w2439
          tunnel: "Show Last Decay only" -> [w2447 w2460]
          tunnel: [w2445 w2453] -> w2438
          tunnel: w2437 -> [_ w2453]
          frame False {
            n489 = Get Variant Attribute(Variant=w2451, name=w2452, default value (empty Variant)=w2447, error in=w2449) -> (duplicate Variant=w2450:variant, value=w2446:bool, error out=w2448:errorcluster)  [unwired: 1 out]
            n490 = To Variant(anything=w2446) -> (Variant=w2445:variant)
          }
          frame True {
            n491 = Variant To Data(type=w2460, Variant=w2453) -> (data=w2455:bool)  [unwired: 1 in, 1 out]
            n492 = Set Variant Attribute(Variant=w2459, name=w2456, value=w2455, error in=w2457) -> (Variant out=w2458:variant, error out=w2454:errorcluster)  [unwired: 1 out]
          }
        }
      }
      frame "Fluorescence Decay_Styles:Decay Graph Color Array" {
        n493 = case shown="True" w2469 {
          tunnel: w2468 -> [w2477 w2481]
          tunnel: w2467 -> [w2476 w2484]
          tunnel: [w2475 w2483] -> w2466
          tunnel: w2465 -> [w2474 w2482]
          tunnel: [w2473 w2479] -> w2464
          tunnel: "Decay Graph Color Array" -> [w2472 w2485]
          tunnel: [w2470 w2478] -> w2463
          tunnel: w2462 -> [_ w2478]
          frame False {
            n494 = Get Variant Attribute(Variant=w2476, name=w2477, default value (empty Variant)=w2472, error in=w2474) -> (duplicate Variant=w2475:variant, value=w2471:u32[], error out=w2473:errorcluster)  [unwired: 1 out]
            n495 = To Variant(anything=w2471) -> (Variant=w2470:variant)
          }
          frame True {
            n496 = Variant To Data(type=w2485, Variant=w2478) -> (data=w2480:u32[])  [unwired: 1 in, 1 out]
            n497 = Set Variant Attribute(Variant=w2484, name=w2481, value=w2480, error in=w2482) -> (Variant out=w2483:variant, error out=w2479:errorcluster)  [unwired: 1 out]
          }
        }
      }
      frame "Fluorescence Decay:Decay Graph Active" {
        w2486 = FALSE  # Not a Settings Window Control
        n498 = case shown="True" w2494 {
          tunnel: w2493 -> [w2502 w2506]
          tunnel: w2492 -> [w2501 w2509]
          tunnel: [w2500 w2508] -> w2491
          tunnel: w2490 -> [w2499 w2507]
          tunnel: [w2498 w2504] -> w2489
          tunnel: w2486 -> [w2497 w2510]
          tunnel: [w2495 w2503] -> w2488
          tunnel: w2487 -> [_ w2503]
          frame False {
            n499 = Get Variant Attribute(Variant=w2501, name=w2502, default value (empty Variant)=w2497, error in=w2499) -> (duplicate Variant=w2500:variant, value=w2496:bool, error out=w2498:errorcluster)  [unwired: 1 out]
            n500 = To Variant(anything=w2496) -> (Variant=w2495:variant)
          }
          frame True {
            n501 = Variant To Data(type=w2510, Variant=w2503) -> (data=w2505:bool)  [unwired: 1 in, 1 out]
            n502 = Set Variant Attribute(Variant=w2509, name=w2506, value=w2505, error in=w2507) -> (Variant out=w2508:variant, error out=w2504:errorcluster)  [unwired: 1 out]
          }
        }
      }
      frame "Fluorescence Decay Statistics:Min Peak Value" {
        n503 = case shown="True" w2519 {
          tunnel: w2518 -> [w2527 w2531]
          tunnel: w2517 -> [w2526 w2534]
          tunnel: [w2525 w2533] -> w2516
          tunnel: w2515 -> [w2524 w2532]
          tunnel: [w2523 w2529] -> w2514
          tunnel: "Min Peak Value" -> [w2522 w2535]
          tunnel: [w2520 w2528] -> w2513
          tunnel: w2512 -> [_ w2528]
          frame False {
            n504 = Get Variant Attribute(Variant=w2526, name=w2527, default value (empty Variant)=w2522, error in=w2524) -> (duplicate Variant=w2525:variant, value=w2521:dbl, error out=w2523:errorcluster)  [unwired: 1 out]
            n505 = To Variant(anything=w2521) -> (Variant=w2520:variant)
          }
          frame True {
            n506 = Variant To Data(type=w2535, Variant=w2528) -> (data=w2530:dbl)  [unwired: 1 in, 1 out]
            n507 = Set Variant Attribute(Variant=w2534, name=w2531, value=w2530, error in=w2532) -> (Variant out=w2533:variant, error out=w2529:errorcluster)  [unwired: 1 out]
          }
        }
      }
      frame "Fluorescence Decay Statistics:Reject Low Decay Peak Pixels" {
        n508 = case shown="True" w2544 {
          tunnel: w2543 -> [w2552 w2556]
          tunnel: w2542 -> [w2551 w2559]
          tunnel: [w2550 w2558] -> w2541
          tunnel: w2540 -> [w2549 w2557]
          tunnel: [w2548 w2554] -> w2539
          tunnel: "Reject Low Decay Peak Pixels" -> [w2547 w2560]
          tunnel: [w2545 w2553] -> w2538
          tunnel: w2537 -> [_ w2553]
          frame False {
            n509 = Get Variant Attribute(Variant=w2551, name=w2552, default value (empty Variant)=w2547, error in=w2549) -> (duplicate Variant=w2550:variant, value=w2546:bool, error out=w2548:errorcluster)  [unwired: 1 out]
            n510 = To Variant(anything=w2546) -> (Variant=w2545:variant)
          }
          frame True {
            n511 = Variant To Data(type=w2560, Variant=w2553) -> (data=w2555:bool)  [unwired: 1 in, 1 out]
            n512 = Set Variant Attribute(Variant=w2559, name=w2556, value=w2555, error in=w2557) -> (Variant out=w2558:variant, error out=w2554:errorcluster)  [unwired: 1 out]
          }
        }
      }
      frame "Fluorescence Decay Statistics:Reject High Decay Peak Pixels" {
        n513 = case shown="True" w2569 {
          tunnel: w2568 -> [w2577 w2581]
          tunnel: w2567 -> [w2576 w2584]
          tunnel: [w2575 w2583] -> w2566
          tunnel: w2565 -> [w2574 w2582]
          tunnel: [w2573 w2579] -> w2564
          tunnel: "Reject High Decay Peak Pixels" -> [w2572 w2585]
          tunnel: [w2570 w2578] -> w2563
          tunnel: w2562 -> [_ w2578]
          frame False {
            n514 = Get Variant Attribute(Variant=w2576, name=w2577, default value (empty Variant)=w2572, error in=w2574) -> (duplicate Variant=w2575:variant, value=w2571:bool, error out=w2573:errorcluster)  [unwired: 1 out]
            n515 = To Variant(anything=w2571) -> (Variant=w2570:variant)
          }
          frame True {
            n516 = Variant To Data(type=w2585, Variant=w2578) -> (data=w2580:bool)  [unwired: 1 in, 1 out]
            n517 = Set Variant Attribute(Variant=w2584, name=w2581, value=w2580, error in=w2582) -> (Variant out=w2583:variant, error out=w2579:errorcluster)  [unwired: 1 out]
          }
        }
      }
      frame "Fluorescence Decay Statistics:Max Peak Value" {
        n518 = case shown="True" w2594 {
          tunnel: w2593 -> [w2602 w2606]
          tunnel: w2592 -> [w2601 w2609]
          tunnel: [w2600 w2608] -> w2591
          tunnel: w2590 -> [w2599 w2607]
          tunnel: [w2598 w2604] -> w2589
          tunnel: "Max Peak Value" -> [w2597 w2610]
          tunnel: [w2595 w2603] -> w2588
          tunnel: w2587 -> [_ w2603]
          frame False {
            n519 = Get Variant Attribute(Variant=w2601, name=w2602, default value (empty Variant)=w2597, error in=w2599) -> (duplicate Variant=w2600:variant, value=w2596:dbl, error out=w2598:errorcluster)  [unwired: 1 out]
            n520 = To Variant(anything=w2596) -> (Variant=w2595:variant)
          }
          frame True {
            n521 = Variant To Data(type=w2610, Variant=w2603) -> (data=w2605:dbl)  [unwired: 1 in, 1 out]
            n522 = Set Variant Attribute(Variant=w2609, name=w2606, value=w2605, error in=w2607) -> (Variant out=w2608:variant, error out=w2604:errorcluster)  [unwired: 1 out]
          }
        }
      }
      frame "Time Traces:Use File Timestamp" {
        n523 = case shown="True" w2619 {
          tunnel: w2618 -> [w2627 w2631]
          tunnel: w2617 -> [w2626 w2634]
          tunnel: [w2625 w2633] -> w2616
          tunnel: w2615 -> [w2624 w2632]
          tunnel: [w2623 w2629] -> w2614
          tunnel: "Use File Timestamp" -> [w2622 w2635]
          tunnel: [w2620 w2628] -> w2613
          tunnel: w2612 -> [_ w2628]
          frame False {
            n524 = Get Variant Attribute(Variant=w2626, name=w2627, default value (empty Variant)=w2622, error in=w2624) -> (duplicate Variant=w2625:variant, value=w2621:bool, error out=w2623:errorcluster)  [unwired: 1 out]
            n525 = To Variant(anything=w2621) -> (Variant=w2620:variant)
          }
          frame True {
            n526 = Variant To Data(type=w2635, Variant=w2628) -> (data=w2630:bool)  [unwired: 1 in, 1 out]
            n527 = Set Variant Attribute(Variant=w2634, name=w2631, value=w2630, error in=w2632) -> (Variant out=w2633:variant, error out=w2629:errorcluster)  [unwired: 1 out]
          }
        }
      }
      frame "Time Traces:Time Step" {
        n528 = case shown="True" w2644 {
          tunnel: w2643 -> [w2652 w2656]
          tunnel: w2642 -> [w2651 w2659]
          tunnel: [w2650 w2658] -> w2641
          tunnel: w2640 -> [w2649 w2657]
          tunnel: [w2648 w2654] -> w2639
          tunnel: "Time Step" -> [w2647 w2660]
          tunnel: [w2645 w2653] -> w2638
          tunnel: w2637 -> [_ w2653]
          frame False {
            n529 = Get Variant Attribute(Variant=w2651, name=w2652, default value (empty Variant)=w2647, error in=w2649) -> (duplicate Variant=w2650:variant, value=w2646:dbl[unit], error out=w2648:errorcluster)  [unwired: 1 out]
            n530 = To Variant(anything=w2646) -> (Variant=w2645:variant)
          }
          frame True {
            n531 = Variant To Data(type=w2660, Variant=w2653) -> (data=w2655:dbl[unit])  [unwired: 1 in, 1 out]
            n532 = Set Variant Attribute(Variant=w2659, name=w2656, value=w2655, error in=w2657) -> (Variant out=w2658:variant, error out=w2654:errorcluster)  [unwired: 1 out]
          }
        }
      }
      frame "Time Traces:Use Intensity Correction File" {
        n533 = case shown="True" w2669 {
          tunnel: w2668 -> [w2677 w2681]
          tunnel: w2667 -> [w2676 w2684]
          tunnel: [w2675 w2683] -> w2666
          tunnel: w2665 -> [w2674 w2682]
          tunnel: [w2673 w2679] -> w2664
          tunnel: "Use Intensity Correction File" -> [w2672 w2685]
          tunnel: [w2670 w2678] -> w2663
          tunnel: w2662 -> [_ w2678]
          frame False {
            n534 = Get Variant Attribute(Variant=w2676, name=w2677, default value (empty Variant)=w2672, error in=w2674) -> (duplicate Variant=w2675:variant, value=w2671:bool, error out=w2673:errorcluster)  [unwired: 1 out]
            n535 = To Variant(anything=w2671) -> (Variant=w2670:variant)
          }
          frame True {
            n536 = Variant To Data(type=w2685, Variant=w2678) -> (data=w2680:bool)  [unwired: 1 in, 1 out]
            n537 = Set Variant Attribute(Variant=w2684, name=w2681, value=w2680, error in=w2682) -> (Variant out=w2683:variant, error out=w2679:errorcluster)  [unwired: 1 out]
          }
        }
      }
      frame "Time Traces:Intensity Correction File" {
        n538 = case shown="True" w2694 {
          tunnel: w2693 -> [w2702 w2706]
          tunnel: w2692 -> [w2701 w2709]
          tunnel: [w2700 w2708] -> w2691
          tunnel: w2690 -> [w2699 w2707]
          tunnel: [w2698 w2704] -> w2689
          tunnel: "Intensity Correction File" -> [w2697 w2710]
          tunnel: [w2695 w2703] -> w2688
          tunnel: w2687 -> [_ w2703]
          frame False {
            n539 = Get Variant Attribute(Variant=w2701, name=w2702, default value (empty Variant)=w2697, error in=w2699) -> (duplicate Variant=w2700:variant, value=w2696:path, error out=w2698:errorcluster)  [unwired: 1 out]
            n540 = To Variant(anything=w2696) -> (Variant=w2695:variant)
          }
          frame True {
            n541 = Variant To Data(type=w2710, Variant=w2703) -> (data=w2705:path)  [unwired: 1 in, 1 out]
            n542 = Set Variant Attribute(Variant=w2709, name=w2706, value=w2705, error in=w2707) -> (Variant out=w2708:variant, error out=w2704:errorcluster)  [unwired: 1 out]
          }
        }
      }
      frame "Phasor Plot:Phasor Plot Smoothing Options" {
        n543 = case shown="True" w2719 {
          tunnel: w2718 -> [w2727 w2731]
          tunnel: w2717 -> [w2726 w2734]
          tunnel: [w2725 w2733] -> w2716
          tunnel: w2715 -> [w2724 w2732]
          tunnel: [w2723 w2729] -> w2714
          tunnel: "Phasor Plot Smoothing Options" -> [w2722 w2735]
          tunnel: [w2720 w2728] -> w2713
          tunnel: w2712 -> [_ w2728]
          frame False {
            n544 = Get Variant Attribute(Variant=w2726, name=w2727, default value (empty Variant)=w2722, error in=w2724) -> (duplicate Variant=w2725:variant, value=w2721:T46, error out=w2723:errorcluster)  [unwired: 1 out]
            n545 = To Variant(anything=w2721) -> (Variant=w2720:variant)
          }
          frame True {
            n546 = Variant To Data(type=w2735, Variant=w2728) -> (data=w2730:T46)  [unwired: 1 in, 1 out]
            n547 = Set Variant Attribute(Variant=w2734, name=w2731, value=w2730, error in=w2732) -> (Variant out=w2733:variant, error out=w2729:errorcluster)  [unwired: 1 out]
          }
        }
      }
      frame "Phasor Plot:Phasor Plot Size" {
        n548 = case shown="True" w2744 {
          tunnel: w2743 -> [w2752 w2756]
          tunnel: w2742 -> [w2751 w2759]
          tunnel: [w2750 w2758] -> w2741
          tunnel: w2740 -> [w2749 w2757]
          tunnel: [w2748 w2754] -> w2739
          tunnel: "Phasor Plot Size" -> [w2747 w2760]
          tunnel: [w2745 w2753] -> w2738
          tunnel: w2737 -> [_ w2753]
          frame False {
            n549 = Get Variant Attribute(Variant=w2751, name=w2752, default value (empty Variant)=w2747, error in=w2749) -> (duplicate Variant=w2750:variant, value=w2746:T49, error out=w2748:errorcluster)  [unwired: 1 out]
            n550 = To Variant(anything=w2746) -> (Variant=w2745:variant)
          }
          frame True {
            n551 = Variant To Data(type=w2760, Variant=w2753) -> (data=w2755:T49)  [unwired: 1 in, 1 out]
            n552 = Set Variant Attribute(Variant=w2759, name=w2756, value=w2755, error in=w2757) -> (Variant out=w2758:variant, error out=w2754:errorcluster)  [unwired: 1 out]
          }
        }
      }
      frame "Phasor Plot:Phasor Plot Graphics Options" {
        n553 = case shown="True" w2769 {
          tunnel: w2768 -> [w2777 w2781]
          tunnel: w2767 -> [w2776 w2784]
          tunnel: [w2775 w2783] -> w2766
          tunnel: w2765 -> [w2774 w2782]
          tunnel: [w2773 w2779] -> w2764
          tunnel: "Phasor Plot Graphics Options" -> [w2772 w2785]
          tunnel: [w2770 w2778] -> w2763
          tunnel: w2762 -> [_ w2778]
          frame False {
            n554 = Get Variant Attribute(Variant=w2776, name=w2777, default value (empty Variant)=w2772, error in=w2774) -> (duplicate Variant=w2775:variant, value=w2771:T45, error out=w2773:errorcluster)  [unwired: 1 out]
            n555 = To Variant(anything=w2771) -> (Variant=w2770:variant)
          }
          frame True {
            n556 = Variant To Data(type=w2785, Variant=w2778) -> (data=w2780:T45)  [unwired: 1 in, 1 out]
            n557 = Set Variant Attribute(Variant=w2784, name=w2781, value=w2780, error in=w2782) -> (Variant out=w2783:variant, error out=w2779:errorcluster)  [unwired: 1 out]
          }
        }
      }
      frame "Phasor Plot:Cumulative Phasor Plot" {
        n558 = case shown="True" w2794 {
          tunnel: w2793 -> [w2802 w2806]
          tunnel: w2792 -> [w2801 w2809]
          tunnel: [w2800 w2808] -> w2791
          tunnel: w2790 -> [w2799 w2807]
          tunnel: [w2798 w2804] -> w2789
          tunnel: "Cumulative Phasor Plot" -> [w2797 w2810]
          tunnel: [w2795 w2803] -> w2788
          tunnel: w2787 -> [_ w2803]
          frame False {
            n559 = Get Variant Attribute(Variant=w2801, name=w2802, default value (empty Variant)=w2797, error in=w2799) -> (duplicate Variant=w2800:variant, value=w2796:bool, error out=w2798:errorcluster)  [unwired: 1 out]
            n560 = To Variant(anything=w2796) -> (Variant=w2795:variant)
          }
          frame True {
            n561 = Variant To Data(type=w2810, Variant=w2803) -> (data=w2805:bool)  [unwired: 1 in, 1 out]
            n562 = Set Variant Attribute(Variant=w2809, name=w2806, value=w2805, error in=w2807) -> (Variant out=w2808:variant, error out=w2804:errorcluster)  [unwired: 1 out]
          }
        }
      }
      frame "Phasor Plot:Use Phasor Brightness" {
        n563 = case shown="True" w2819 {
          tunnel: w2818 -> [w2827 w2831]
          tunnel: w2817 -> [w2826 w2834]
          tunnel: [w2825 w2833] -> w2816
          tunnel: w2815 -> [w2824 w2832]
          tunnel: [w2823 w2829] -> w2814
          tunnel: "Use Phasor Brightness" -> [w2822 w2835]
          tunnel: [w2820 w2828] -> w2813
          tunnel: w2812 -> [_ w2828]
          frame False {
            n564 = Get Variant Attribute(Variant=w2826, name=w2827, default value (empty Variant)=w2822, error in=w2824) -> (duplicate Variant=w2825:variant, value=w2821:bool, error out=w2823:errorcluster)  [unwired: 1 out]
            n565 = To Variant(anything=w2821) -> (Variant=w2820:variant)
          }
          frame True {
            n566 = Variant To Data(type=w2835, Variant=w2828) -> (data=w2830:bool)  [unwired: 1 in, 1 out]
            n567 = Set Variant Attribute(Variant=w2834, name=w2831, value=w2830, error in=w2832) -> (Variant out=w2833:variant, error out=w2829:errorcluster)  [unwired: 1 out]
          }
        }
      }
      frame "Phasor Plot:Blend Overlay with Phasor Background" {
        n568 = case shown="True" w2844 {
          tunnel: w2843 -> [w2852 w2856]
          tunnel: w2842 -> [w2851 w2859]
          tunnel: [w2850 w2858] -> w2841
          tunnel: w2840 -> [w2849 w2857]
          tunnel: [w2848 w2854] -> w2839
          tunnel: "Blend Overlay with Phasor Background" -> [w2847 w2860]
          tunnel: [w2845 w2853] -> w2838
          tunnel: w2837 -> [_ w2853]
          frame False {
            n569 = Get Variant Attribute(Variant=w2851, name=w2852, default value (empty Variant)=w2847, error in=w2849) -> (duplicate Variant=w2850:variant, value=w2846:bool, error out=w2848:errorcluster)  [unwired: 1 out]
            n570 = To Variant(anything=w2846) -> (Variant=w2845:variant)
          }
          frame True {
            n571 = Variant To Data(type=w2860, Variant=w2853) -> (data=w2855:bool)  [unwired: 1 in, 1 out]
            n572 = Set Variant Attribute(Variant=w2859, name=w2856, value=w2855, error in=w2857) -> (Variant out=w2858:variant, error out=w2854:errorcluster)  [unwired: 1 out]
          }
        }
      }
      frame "Phasor Plot:Save Phasor Plot" {
        n573 = case shown="True" w2869 {
          tunnel: w2868 -> [w2877 w2881]
          tunnel: w2867 -> [w2876 w2884]
          tunnel: [w2875 w2883] -> w2866
          tunnel: w2865 -> [w2874 w2882]
          tunnel: [w2873 w2879] -> w2864
          tunnel: "Save Phasor Plot" -> [w2872 w2885]
          tunnel: [w2870 w2878] -> w2863
          tunnel: w2862 -> [_ w2878]
          frame False {
            n574 = Get Variant Attribute(Variant=w2876, name=w2877, default value (empty Variant)=w2872, error in=w2874) -> (duplicate Variant=w2875:variant, value=w2871:bool, error out=w2873:errorcluster)  [unwired: 1 out]
            n575 = To Variant(anything=w2871) -> (Variant=w2870:variant)
          }
          frame True {
            n576 = Variant To Data(type=w2885, Variant=w2878) -> (data=w2880:bool)  [unwired: 1 in, 1 out]
            n577 = Set Variant Attribute(Variant=w2884, name=w2881, value=w2880, error in=w2882) -> (Variant out=w2883:variant, error out=w2879:errorcluster)  [unwired: 1 out]
          }
        }
      }
      frame "Phasor Plot:Show References" {
        n578 = case shown="True" w2894 {
          tunnel: w2893 -> [w2902 w2906]
          tunnel: w2892 -> [w2901 w2909]
          tunnel: [w2900 w2908] -> w2891
          tunnel: w2890 -> [w2899 w2907]
          tunnel: [w2898 w2904] -> w2889
          tunnel: "Show References" -> [w2897 w2910]
          tunnel: [w2895 w2903] -> w2888
          tunnel: w2887 -> [_ w2903]
          frame False {
            n579 = Get Variant Attribute(Variant=w2901, name=w2902, default value (empty Variant)=w2897, error in=w2899) -> (duplicate Variant=w2900:variant, value=w2896:bool, error out=w2898:errorcluster)  [unwired: 1 out]
            n580 = To Variant(anything=w2896) -> (Variant=w2895:variant)
          }
          frame True {
            n581 = Variant To Data(type=w2910, Variant=w2903) -> (data=w2905:bool)  [unwired: 1 in, 1 out]
            n582 = Set Variant Attribute(Variant=w2909, name=w2906, value=w2905, error in=w2907) -> (Variant out=w2908:variant, error out=w2904:errorcluster)  [unwired: 1 out]
          }
        }
      }
      frame "Phasor Plot:Phasor Ratio Decay Range" {
        n583 = case shown="True" w2919 {
          tunnel: w2918 -> [w2927 w2931]
          tunnel: w2917 -> [w2926 w2934]
          tunnel: [w2925 w2933] -> w2916
          tunnel: w2915 -> [w2924 w2932]
          tunnel: [w2923 w2929] -> w2914
          tunnel: "Phasor Ratio Decay Range" -> [w2922 w2935]
          tunnel: [w2920 w2928] -> w2913
          tunnel: w2912 -> [_ w2928]
          frame False {
            n584 = Get Variant Attribute(Variant=w2926, name=w2927, default value (empty Variant)=w2922, error in=w2924) -> (duplicate Variant=w2925:variant, value=w2921:dbl, error out=w2923:errorcluster)  [unwired: 1 out]
            n585 = To Variant(anything=w2921) -> (Variant=w2920:variant)
          }
          frame True {
            n586 = Variant To Data(type=w2935, Variant=w2928) -> (data=w2930:dbl)  [unwired: 1 in, 1 out]
            n587 = Set Variant Attribute(Variant=w2934, name=w2931, value=w2930, error in=w2932) -> (Variant out=w2933:variant, error out=w2929:errorcluster)  [unwired: 1 out]
          }
        }
      }
      frame "Phasor Plot:Exponential Fading" {
        n588 = case shown="True" w2944 {
          tunnel: w2943 -> [w2952 w2956]
          tunnel: w2942 -> [w2951 w2959]
          tunnel: [w2950 w2958] -> w2941
          tunnel: w2940 -> [w2949 w2957]
          tunnel: [w2948 w2954] -> w2939
          tunnel: "Exponential Fading" -> [w2947 w2960]
          tunnel: [w2945 w2953] -> w2938
          tunnel: w2937 -> [_ w2953]
          frame False {
            n589 = Get Variant Attribute(Variant=w2951, name=w2952, default value (empty Variant)=w2947, error in=w2949) -> (duplicate Variant=w2950:variant, value=w2946:bool, error out=w2948:errorcluster)  [unwired: 1 out]
            n590 = To Variant(anything=w2946) -> (Variant=w2945:variant)
          }
          frame True {
            n591 = Variant To Data(type=w2960, Variant=w2953) -> (data=w2955:bool)  [unwired: 1 in, 1 out]
            n592 = Set Variant Attribute(Variant=w2959, name=w2956, value=w2955, error in=w2957) -> (Variant out=w2958:variant, error out=w2954:errorcluster)  [unwired: 1 out]
          }
        }
      }
      frame "Phasor Plot:Phasor Ratio Reference Colors" {
        n593 = case shown="True" w2969 {
          tunnel: w2968 -> [w2977 w2981]
          tunnel: w2967 -> [w2976 w2984]
          tunnel: [w2975 w2983] -> w2966
          tunnel: w2965 -> [w2974 w2982]
          tunnel: [w2973 w2979] -> w2964
          tunnel: "Phasor Ratio Reference Colors" -> [w2972 w2985]
          tunnel: [w2970 w2978] -> w2963
          tunnel: w2962 -> [_ w2978]
          frame False {
            n594 = Get Variant Attribute(Variant=w2976, name=w2977, default value (empty Variant)=w2972, error in=w2974) -> (duplicate Variant=w2975:variant, value=w2971:T48, error out=w2973:errorcluster)  [unwired: 1 out]
            n595 = To Variant(anything=w2971) -> (Variant=w2970:variant)
          }
          frame True {
            n596 = Variant To Data(type=w2985, Variant=w2978) -> (data=w2980:T48)  [unwired: 1 in, 1 out]
            n597 = Set Variant Attribute(Variant=w2984, name=w2981, value=w2980, error in=w2982) -> (Variant out=w2983:variant, error out=w2979:errorcluster)  [unwired: 1 out]
          }
        }
      }
      frame "Phasor Plot:Reference Radius" {
        n598 = case shown="True" w2994 {
          tunnel: w2993 -> [w3002 w3006]
          tunnel: w2992 -> [w3001 w3009]
          tunnel: [w3000 w3008] -> w2991
          tunnel: w2990 -> [w2999 w3007]
          tunnel: [w2998 w3004] -> w2989
          tunnel: "Reference Radius" -> [w2997 w3010]
          tunnel: [w2995 w3003] -> w2988
          tunnel: w2987 -> [_ w3003]
          frame False {
            n599 = Get Variant Attribute(Variant=w3001, name=w3002, default value (empty Variant)=w2997, error in=w2999) -> (duplicate Variant=w3000:variant, value=w2996:i32, error out=w2998:errorcluster)  [unwired: 1 out]
            n600 = To Variant(anything=w2996) -> (Variant=w2995:variant)
          }
          frame True {
            n601 = Variant To Data(type=w3010, Variant=w3003) -> (data=w3005:i32)  [unwired: 1 in, 1 out]
            n602 = Set Variant Attribute(Variant=w3009, name=w3006, value=w3005, error in=w3007) -> (Variant out=w3008:variant, error out=w3004:errorcluster)  [unwired: 1 out]
          }
        }
      }
      frame "Phasor Plot:Show Color Map Vertices" {
        n603 = case shown="True" w3019 {
          tunnel: w3018 -> [w3027 w3031]
          tunnel: w3017 -> [w3026 w3034]
          tunnel: [w3025 w3033] -> w3016
          tunnel: w3015 -> [w3024 w3032]
          tunnel: [w3023 w3029] -> w3014
          tunnel: "Show Color Map Vertices" -> [w3022 w3035]
          tunnel: [w3020 w3028] -> w3013
          tunnel: w3012 -> [_ w3028]
          frame False {
            n604 = Get Variant Attribute(Variant=w3026, name=w3027, default value (empty Variant)=w3022, error in=w3024) -> (duplicate Variant=w3025:variant, value=w3021:bool, error out=w3023:errorcluster)  [unwired: 1 out]
            n605 = To Variant(anything=w3021) -> (Variant=w3020:variant)
          }
          frame True {
            n606 = Variant To Data(type=w3035, Variant=w3028) -> (data=w3030:bool)  [unwired: 1 in, 1 out]
            n607 = Set Variant Attribute(Variant=w3034, name=w3031, value=w3030, error in=w3032) -> (Variant out=w3033:variant, error out=w3029:errorcluster)  [unwired: 1 out]
          }
        }
      }
      frame "Phasor Plot:Phasor Plot Active" {
        w3036 = FALSE  # Not a Settings Window Control
        n608 = case shown="True" w3044 {
          tunnel: w3043 -> [w3052 w3056]
          tunnel: w3042 -> [w3051 w3059]
          tunnel: [w3050 w3058] -> w3041
          tunnel: w3040 -> [w3049 w3057]
          tunnel: [w3048 w3054] -> w3039
          tunnel: w3036 -> [w3047 w3060]
          tunnel: [w3045 w3053] -> w3038
          tunnel: w3037 -> [_ w3053]
          frame False {
            n609 = Get Variant Attribute(Variant=w3051, name=w3052, default value (empty Variant)=w3047, error in=w3049) -> (duplicate Variant=w3050:variant, value=w3046:bool, error out=w3048:errorcluster)  [unwired: 1 out]
            n610 = To Variant(anything=w3046) -> (Variant=w3045:variant)
          }
          frame True {
            n611 = Variant To Data(type=w3060, Variant=w3053) -> (data=w3055:bool)  [unwired: 1 in, 1 out]
            n612 = Set Variant Attribute(Variant=w3059, name=w3056, value=w3055, error in=w3057) -> (Variant out=w3058:variant, error out=w3054:errorcluster)  [unwired: 1 out]
          }
        }
      }
      frame "Phasor Plot:Phasor Ratio Color Map Type" {
        n613 = case shown="True" w3069 {
          tunnel: w3068 -> [w3077 w3081]
          tunnel: w3067 -> [w3076 w3084]
          tunnel: [w3075 w3083] -> w3066
          tunnel: w3065 -> [w3074 w3082]
          tunnel: [w3073 w3079] -> w3064
          tunnel: "Phasor Ratio Color Map Type" -> [w3072 w3085]
          tunnel: [w3070 w3078] -> w3063
          tunnel: w3062 -> [_ w3078]
          frame False {
            n614 = Get Variant Attribute(Variant=w3076, name=w3077, default value (empty Variant)=w3072, error in=w3074) -> (duplicate Variant=w3075:variant, value=w3071:T47, error out=w3073:errorcluster)  [unwired: 1 out]
            n615 = To Variant(anything=w3071) -> (Variant=w3070:variant)
          }
          frame True {
            n616 = Variant To Data(type=w3085, Variant=w3078) -> (data=w3080:T47)  [unwired: 1 in, 1 out]
            n617 = Set Variant Attribute(Variant=w3084, name=w3081, value=w3080, error in=w3082) -> (Variant out=w3083:variant, error out=w3079:errorcluster)  [unwired: 1 out]
          }
        }
      }
      frame "Phasor Plot:Phasor Ratio Color Map" {
        n618 = case shown="True" w3094 {
          tunnel: w3093 -> [w3102 w3106]
          tunnel: w3092 -> [w3101 w3109]
          tunnel: [w3100 w3108] -> w3091
          tunnel: w3090 -> [w3099 w3107]
          tunnel: [w3098 w3104] -> w3089
          tunnel: "Phasor Ratio Color Map" -> [w3097 w3110]
          tunnel: [w3095 w3103] -> w3088
          tunnel: w3087 -> [_ w3103]
          frame False {
            n619 = Get Variant Attribute(Variant=w3101, name=w3102, default value (empty Variant)=w3097, error in=w3099) -> (duplicate Variant=w3100:variant, value=w3096:string, error out=w3098:errorcluster)  [unwired: 1 out]
            n620 = To Variant(anything=w3096) -> (Variant=w3095:variant)
          }
          frame True {
            n621 = Variant To Data(type=w3110, Variant=w3103) -> (data=w3105:string)  [unwired: 1 in, 1 out]
            n622 = Set Variant Attribute(Variant=w3109, name=w3106, value=w3105, error in=w3107) -> (Variant out=w3108:variant, error out=w3104:errorcluster)  [unwired: 1 out]
          }
        }
      }
      frame "Phasor Plot:Phasor Ratio Display Range" {
        n623 = Variant To Data(error in=w3113, type=cluster{"Min":dbl, "Max":dbl} {"Min"=0.0, "Max"=1.0} ("Phasor Ratio Display Range"), Variant="Phasor Ratio Display Range") -> (data=w3114:cluster{"Min":dbl, "Max":dbl}, error out=w3112:errorcluster)
        n624 = case shown="True" w3122 {
          tunnel: w3121 -> [w3130 w3134]
          tunnel: w3120 -> [w3129 w3137]
          tunnel: [w3128 w3136] -> w3119
          tunnel: w3112 -> [w3127 w3135]
          tunnel: [w3126 w3132] -> w3118
          tunnel: w3114 -> [w3125 w3138]
          tunnel: [w3123 w3131] -> w3117
          tunnel: w3116 -> [_ w3131]
          frame False {
            n625 = Get Variant Attribute(Variant=w3129, name=w3130, default value (empty Variant)=w3125, error in=w3127) -> (duplicate Variant=w3128:variant, value=w3124:cluster{"Min":dbl, "Max":dbl}, error out=w3126:errorcluster)  [unwired: 1 out]
            n626 = To Variant(anything=w3124) -> (Variant=w3123:variant)
          }
          frame True {
            n627 = Variant To Data(type=w3138, Variant=w3131) -> (data=w3133:cluster{"Min":dbl, "Max":dbl})  [unwired: 1 in, 1 out]
            n628 = Set Variant Attribute(Variant=w3137, name=w3134, value=w3133, error in=w3135) -> (Variant out=w3136:variant, error out=w3132:errorcluster)  [unwired: 1 out]
          }
        }
      }
      frame "Phasor Plot:Selected Image ROI(s)" {
        n629 = case shown="True" w3147 {
          tunnel: w3146 -> [w3155 w3159]
          tunnel: w3145 -> [w3154 w3162]
          tunnel: [w3153 w3161] -> w3144
          tunnel: w3140 -> [w3152 w3160]
          tunnel: [w3151 w3157] -> w3143
          tunnel: "Selected Image ROI(s)" -> [w3150 w3163]
          tunnel: [w3148 w3156] -> w3142
          tunnel: w3141 -> [_ w3156]
          frame False {
            n630 = Get Variant Attribute(Variant=w3154, name=w3155, default value (empty Variant)=w3150, error in=w3152) -> (duplicate Variant=w3153:variant, value=w3149:bool, error out=w3151:errorcluster)  [unwired: 1 out]
            n631 = To Variant(anything=w3149) -> (Variant=w3148:variant)
          }
          frame True {
            n632 = Variant To Data(type=w3163, Variant=w3156) -> (data=w3158:bool)  [unwired: 1 in, 1 out]
            n633 = Set Variant Attribute(Variant=w3162, name=w3159, value=w3158, error in=w3160) -> (Variant out=w3161:variant, error out=w3157:errorcluster)  [unwired: 1 out]
          }
        }
      }
      frame "Phasor Plot:All Image ROIs" {
        n634 = case shown="True" w3172 {
          tunnel: w3171 -> [w3180 w3184]
          tunnel: w3170 -> [w3179 w3187]
          tunnel: [w3178 w3186] -> w3169
          tunnel: w3165 -> [w3177 w3185]
          tunnel: [w3176 w3182] -> w3168
          tunnel: "All Image ROIs" -> [w3175 w3188]
          tunnel: [w3173 w3181] -> w3167
          tunnel: w3166 -> [_ w3181]
          frame False {
            n635 = Get Variant Attribute(Variant=w3179, name=w3180, default value (empty Variant)=w3175, error in=w3177) -> (duplicate Variant=w3178:variant, value=w3174:bool, error out=w3176:errorcluster)  [unwired: 1 out]
            n636 = To Variant(anything=w3174) -> (Variant=w3173:variant)
          }
          frame True {
            n637 = Variant To Data(type=w3188, Variant=w3181) -> (data=w3183:bool)  [unwired: 1 in, 1 out]
            n638 = Set Variant Attribute(Variant=w3187, name=w3184, value=w3183, error in=w3185) -> (Variant out=w3186:variant, error out=w3182:errorcluster)  [unwired: 1 out]
          }
        }
      }
      frame "Phasor Plot:Selected Phasor Plot ROI(s)" {
        n639 = case shown="True" w3197 {
          tunnel: w3196 -> [w3205 w3209]
          tunnel: w3195 -> [w3204 w3212]
          tunnel: [w3203 w3211] -> w3194
          tunnel: w3190 -> [w3202 w3210]
          tunnel: [w3201 w3207] -> w3193
          tunnel: "Selected Phasor Plot ROI(s)" -> [w3200 w3213]
          tunnel: [w3198 w3206] -> w3192
          tunnel: w3191 -> [_ w3206]
          frame False {
            n640 = Get Variant Attribute(Variant=w3204, name=w3205, default value (empty Variant)=w3200, error in=w3202) -> (duplicate Variant=w3203:variant, value=w3199:bool, error out=w3201:errorcluster)  [unwired: 1 out]
            n641 = To Variant(anything=w3199) -> (Variant=w3198:variant)
          }
          frame True {
            n642 = Variant To Data(type=w3213, Variant=w3206) -> (data=w3208:bool)  [unwired: 1 in, 1 out]
            n643 = Set Variant Attribute(Variant=w3212, name=w3209, value=w3208, error in=w3210) -> (Variant out=w3211:variant, error out=w3207:errorcluster)  [unwired: 1 out]
          }
        }
      }
      frame "Phasor Plot:All Phasor Plot ROIs" {
        n644 = case shown="True" w3222 {
          tunnel: w3221 -> [w3230 w3234]
          tunnel: w3220 -> [w3229 w3237]
          tunnel: [w3228 w3236] -> w3219
          tunnel: w3215 -> [w3227 w3235]
          tunnel: [w3226 w3232] -> w3218
          tunnel: "All Phasor Plot ROIs" -> [w3225 w3238]
          tunnel: [w3223 w3231] -> w3217
          tunnel: w3216 -> [_ w3231]
          frame False {
            n645 = Get Variant Attribute(Variant=w3229, name=w3230, default value (empty Variant)=w3225, error in=w3227) -> (duplicate Variant=w3228:variant, value=w3224:bool, error out=w3226:errorcluster)  [unwired: 1 out]
            n646 = To Variant(anything=w3224) -> (Variant=w3223:variant)
          }
          frame True {
            n647 = Variant To Data(type=w3238, Variant=w3231) -> (data=w3233:bool)  [unwired: 1 in, 1 out]
            n648 = Set Variant Attribute(Variant=w3237, name=w3234, value=w3233, error in=w3235) -> (Variant out=w3236:variant, error out=w3232:errorcluster)  [unwired: 1 out]
          }
        }
      }
      frame "Phasor Plot:Phasor Ratio Color-Coded Quantity" {
        n649 = case shown="True" w3247 {
          tunnel: w3246 -> [w3255 w3259]
          tunnel: w3245 -> [w3254 w3262]
          tunnel: [w3253 w3261] -> w3244
          tunnel: w3240 -> [w3252 w3260]
          tunnel: [w3251 w3257] -> w3243
          tunnel: "Phasor Ratio Color-Coded Quantity" -> [w3250 w3263]
          tunnel: [w3248 w3256] -> w3242
          tunnel: w3241 -> [_ w3256]
          frame False {
            n650 = Get Variant Attribute(Variant=w3254, name=w3255, default value (empty Variant)=w3250, error in=w3252) -> (duplicate Variant=w3253:variant, value=w3249:T44, error out=w3251:errorcluster)  [unwired: 1 out]
            n651 = To Variant(anything=w3249) -> (Variant=w3248:variant)
          }
          frame True {
            n652 = Variant To Data(type=w3263, Variant=w3256) -> (data=w3258:T44)  [unwired: 1 in, 1 out]
            n653 = Set Variant Attribute(Variant=w3262, name=w3259, value=w3258, error in=w3260) -> (Variant out=w3261:variant, error out=w3257:errorcluster)  [unwired: 1 out]
          }
        }
      }
      frame "Phasor Plot:Store Phasor Harmonics" {
        n654 = case shown="True" w3272 {
          tunnel: w3271 -> [w3280 w3284]
          tunnel: w3270 -> [w3279 w3287]
          tunnel: [w3278 w3286] -> w3269
          tunnel: w3265 -> [w3277 w3285]
          tunnel: [w3276 w3282] -> w3268
          tunnel: "Store Phasor Harmonics" -> [w3275 w3288]
          tunnel: [w3273 w3281] -> w3267
          tunnel: w3266 -> [_ w3281]
          frame False {
            n655 = Get Variant Attribute(Variant=w3279, name=w3280, default value (empty Variant)=w3275, error in=w3277) -> (duplicate Variant=w3278:variant, value=w3274:bool, error out=w3276:errorcluster)  [unwired: 1 out]
            n656 = To Variant(anything=w3274) -> (Variant=w3273:variant)
          }
          frame True {
            n657 = Variant To Data(type=w3288, Variant=w3281) -> (data=w3283:bool)  [unwired: 1 in, 1 out]
            n658 = Set Variant Attribute(Variant=w3287, name=w3284, value=w3283, error in=w3285) -> (Variant out=w3286:variant, error out=w3282:errorcluster)  [unwired: 1 out]
          }
        }
      }
      frame "Phasor Plot:Draw Reference Segment" {
        n659 = case shown="True" w3297 {
          tunnel: w3296 -> [w3305 w3309]
          tunnel: w3295 -> [w3304 w3312]
          tunnel: [w3303 w3311] -> w3294
          tunnel: w3290 -> [w3302 w3310]
          tunnel: [w3301 w3307] -> w3293
          tunnel: "Draw Reference Segment" -> [w3300 w3313]
          tunnel: [w3298 w3306] -> w3292
          tunnel: w3291 -> [_ w3306]
          frame False {
            n660 = Get Variant Attribute(Variant=w3304, name=w3305, default value (empty Variant)=w3300, error in=w3302) -> (duplicate Variant=w3303:variant, value=w3299:bool, error out=w3301:errorcluster)  [unwired: 1 out]
            n661 = To Variant(anything=w3299) -> (Variant=w3298:variant)
          }
          frame True {
            n662 = Variant To Data(type=w3313, Variant=w3306) -> (data=w3308:bool)  [unwired: 1 in, 1 out]
            n663 = Set Variant Attribute(Variant=w3312, name=w3309, value=w3308, error in=w3310) -> (Variant out=w3311:variant, error out=w3307:errorcluster)  [unwired: 1 out]
          }
        }
      }
      frame "Phasor Plot:User-Defined Quantity" {
        n664 = case shown="True" w3322 {
          tunnel: w3321 -> [w3330 w3334]
          tunnel: w3320 -> [w3329 w3337]
          tunnel: [w3328 w3336] -> w3319
          tunnel: w3315 -> [w3327 w3335]
          tunnel: [w3326 w3332] -> w3318
          tunnel: "User-defined Quantity" -> [w3325 w3338]
          tunnel: [w3323 w3331] -> w3317
          tunnel: w3316 -> [_ w3331]
          frame False {
            n665 = Get Variant Attribute(Variant=w3329, name=w3330, default value (empty Variant)=w3325, error in=w3327) -> (duplicate Variant=w3328:variant, value=w3324:string, error out=w3326:errorcluster)  [unwired: 1 out]
            n666 = To Variant(anything=w3324) -> (Variant=w3323:variant)
          }
          frame True {
            n667 = Variant To Data(type=w3338, Variant=w3331) -> (data=w3333:string)  [unwired: 1 in, 1 out]
            n668 = Set Variant Attribute(Variant=w3337, name=w3334, value=w3333, error in=w3335) -> (Variant out=w3336:variant, error out=w3332:errorcluster)  [unwired: 1 out]
          }
        }
      }
      frame "Phasor Graph:Phasor Frequency" {
        n669 = case shown="True" w3347 {
          tunnel: w3346 -> [w3355 w3359]
          tunnel: w3345 -> [w3354 w3362]
          tunnel: [w3353 w3361] -> w3344
          tunnel: w3343 -> [w3352 w3360]
          tunnel: [w3351 w3357] -> w3342
          tunnel: "Phasor Frequency" -> [w3350 w3363]
          tunnel: [w3348 w3356] -> w3341
          tunnel: w3340 -> [_ w3356]
          frame False {
            n670 = Get Variant Attribute(Variant=w3354, name=w3355, default value (empty Variant)=w3350, error in=w3352) -> (duplicate Variant=w3353:variant, value=w3349:dbl[unit], error out=w3351:errorcluster)  [unwired: 1 out]
            n671 = To Variant(anything=w3349) -> (Variant=w3348:variant)
          }
          frame True {
            n672 = Variant To Data(type=w3363, Variant=w3356) -> (data=w3358:dbl[unit])  [unwired: 1 in, 1 out]
            n673 = Set Variant Attribute(Variant=w3362, name=w3359, value=w3358, error in=w3360) -> (Variant out=w3361:variant, error out=w3357:errorcluster)  [unwired: 1 out]
          }
        }
      }
      frame "Phasor Graph:Phasor Ratio Type" {
        # "item 0: Intensity-weighted\nitem 1: amplitude-weighted"
        n674 = case shown="True" w3372 {
          tunnel: w3371 -> [w3380 w3384]
          tunnel: w3370 -> [w3379 w3387]
          tunnel: [w3378 w3386] -> w3369
          tunnel: w3368 -> [w3377 w3385]
          tunnel: [w3376 w3382] -> w3367
          tunnel: "Phasor Ratio Type" -> [w3375 w3388]
          tunnel: [w3373 w3381] -> w3366
          tunnel: w3365 -> [_ w3381]
          frame False {
            n675 = Get Variant Attribute(Variant=w3379, name=w3380, default value (empty Variant)=w3375, error in=w3377) -> (duplicate Variant=w3378:variant, value=w3374:T52, error out=w3376:errorcluster)  [unwired: 1 out]
            n676 = To Variant(anything=w3374) -> (Variant=w3373:variant)
          }
          frame True {
            n677 = Variant To Data(type=w3388, Variant=w3381) -> (data=w3383:T52)  [unwired: 1 in, 1 out]
            n678 = Set Variant Attribute(Variant=w3387, name=w3384, value=w3383, error in=w3385) -> (Variant out=w3386:variant, error out=w3382:errorcluster)  [unwired: 1 out]
          }
        }
      }
      frame "Phasor Graph:Pixel-level Phasor Computation" {
        n679 = case shown="True" w3397 {
          tunnel: w3396 -> [w3405 w3409]
          tunnel: w3395 -> [w3404 w3412]
          tunnel: [w3403 w3411] -> w3394
          tunnel: w3393 -> [w3402 w3410]
          tunnel: [w3401 w3407] -> w3392
          tunnel: "Pixel-level Phasor Computation" -> [w3400 w3413]
          tunnel: [w3398 w3406] -> w3391
          tunnel: w3390 -> [_ w3406]
          frame False {
            n680 = Get Variant Attribute(Variant=w3404, name=w3405, default value (empty Variant)=w3400, error in=w3402) -> (duplicate Variant=w3403:variant, value=w3399:bool, error out=w3401:errorcluster)  [unwired: 1 out]
            n681 = To Variant(anything=w3399) -> (Variant=w3398:variant)
          }
          frame True {
            n682 = Variant To Data(type=w3413, Variant=w3406) -> (data=w3408:bool)  [unwired: 1 in, 1 out]
            n683 = Set Variant Attribute(Variant=w3412, name=w3409, value=w3408, error in=w3410) -> (Variant out=w3411:variant, error out=w3407:errorcluster)  [unwired: 1 out]
          }
        }
      }
      frame "Phasor Graph:Save Phasor Graph" {
        n684 = case shown="True" w3422 {
          tunnel: w3421 -> [w3430 w3434]
          tunnel: w3420 -> [w3429 w3437]
          tunnel: [w3428 w3436] -> w3419
          tunnel: w3418 -> [w3427 w3435]
          tunnel: [w3426 w3432] -> w3417
          tunnel: "Save Phasor Graph Image" -> [w3425 w3438]
          tunnel: [w3423 w3431] -> w3416
          tunnel: w3415 -> [_ w3431]
          frame False {
            n685 = Get Variant Attribute(Variant=w3429, name=w3430, default value (empty Variant)=w3425, error in=w3427) -> (duplicate Variant=w3428:variant, value=w3424:bool, error out=w3426:errorcluster)  [unwired: 1 out]
            n686 = To Variant(anything=w3424) -> (Variant=w3423:variant)
          }
          frame True {
            n687 = Variant To Data(type=w3438, Variant=w3431) -> (data=w3433:bool)  [unwired: 1 in, 1 out]
            n688 = Set Variant Attribute(Variant=w3437, name=w3434, value=w3433, error in=w3435) -> (Variant out=w3436:variant, error out=w3432:errorcluster)  [unwired: 1 out]
          }
        }
      }
      frame "Phasor Graph:Phasor Graph Active" {
        n689 = case shown="True" w3447 {
          tunnel: w3446 -> [w3455 w3459]
          tunnel: w3445 -> [w3454 w3462]
          tunnel: [w3453 w3461] -> w3444
          tunnel: w3443 -> [w3452 w3460]
          tunnel: [w3451 w3457] -> w3442
          tunnel: "Phasor Graph Active" -> [w3450 w3463]
          tunnel: [w3448 w3456] -> w3441
          tunnel: w3440 -> [_ w3456]
          frame False {
            n690 = Get Variant Attribute(Variant=w3454, name=w3455, default value (empty Variant)=w3450, error in=w3452) -> (duplicate Variant=w3453:variant, value=w3449:bool, error out=w3451:errorcluster)  [unwired: 1 out]
            n691 = To Variant(anything=w3449) -> (Variant=w3448:variant)
          }
          frame True {
            n692 = Variant To Data(type=w3463, Variant=w3456) -> (data=w3458:bool)  [unwired: 1 in, 1 out]
            n693 = Set Variant Attribute(Variant=w3462, name=w3459, value=w3458, error in=w3460) -> (Variant out=w3461:variant, error out=w3457:errorcluster)  [unwired: 1 out]
          }
        }
      }
      frame "Phasor Graph:Phasor SDV Options" {
        n694 = case shown="True" w3472 {
          tunnel: w3471 -> [w3480 w3484]
          tunnel: w3470 -> [w3479 w3487]
          tunnel: [w3478 w3486] -> w3469
          tunnel: w3468 -> [w3477 w3485]
          tunnel: [w3476 w3482] -> w3467
          tunnel: "Phasor SDV Options" -> [w3475 w3488]
          tunnel: [w3473 w3481] -> w3466
          tunnel: w3465 -> [_ w3481]
          frame False {
            n695 = Get Variant Attribute(Variant=w3479, name=w3480, default value (empty Variant)=w3475, error in=w3477) -> (duplicate Variant=w3478:variant, value=w3474:T50, error out=w3476:errorcluster)  [unwired: 1 out]
            n696 = To Variant(anything=w3474) -> (Variant=w3473:variant)
          }
          frame True {
            n697 = Variant To Data(type=w3488, Variant=w3481) -> (data=w3483:T50)  [unwired: 1 in, 1 out]
            n698 = Set Variant Attribute(Variant=w3487, name=w3484, value=w3483, error in=w3485) -> (Variant out=w3486:variant, error out=w3482:errorcluster)  [unwired: 1 out]
          }
        }
      }
      frame "Phasor Calibration:Use Backup Calibration if needed" {
        n699 = case shown="True" w3497 {
          tunnel: w3496 -> [w3505 w3509]
          tunnel: w3495 -> [w3504 w3512]
          tunnel: [w3503 w3511] -> w3494
          tunnel: w3493 -> [w3502 w3510]
          tunnel: [w3501 w3507] -> w3492
          tunnel: "Use Backup Calibration if needed" -> [w3500 w3513]
          tunnel: [w3498 w3506] -> w3491
          tunnel: w3490 -> [_ w3506]
          frame False {
            n700 = Get Variant Attribute(Variant=w3504, name=w3505, default value (empty Variant)=w3500, error in=w3502) -> (duplicate Variant=w3503:variant, value=w3499:bool, error out=w3501:errorcluster)  [unwired: 1 out]
            n701 = To Variant(anything=w3499) -> (Variant=w3498:variant)
          }
          frame True {
            n702 = Variant To Data(type=w3513, Variant=w3506) -> (data=w3508:bool)  [unwired: 1 in, 1 out]
            n703 = Set Variant Attribute(Variant=w3512, name=w3509, value=w3508, error in=w3510) -> (Variant out=w3511:variant, error out=w3507:errorcluster)  [unwired: 1 out]
          }
        }
      }
      frame "Phasor Graph:Define Shortest Lifetime as" {
        n704 = case shown="True" w3522 {
          tunnel: w3521 -> [w3530 w3534]
          tunnel: w3520 -> [w3529 w3537]
          tunnel: [w3528 w3536] -> w3519
          tunnel: w3518 -> [w3527 w3535]
          tunnel: [w3526 w3532] -> w3517
          tunnel: "Define Shortest Lifetime as" -> [w3525 w3538]
          tunnel: [w3523 w3531] -> w3516
          tunnel: w3515 -> [_ w3531]
          frame False {
            n705 = Get Variant Attribute(Variant=w3529, name=w3530, default value (empty Variant)=w3525, error in=w3527) -> (duplicate Variant=w3528:variant, value=w3524:T51, error out=w3526:errorcluster)  [unwired: 1 out]
            n706 = To Variant(anything=w3524) -> (Variant=w3523:variant)
          }
          frame True {
            n707 = Variant To Data(type=w3538, Variant=w3531) -> (data=w3533:T51)  [unwired: 1 in, 1 out]
            n708 = Set Variant Attribute(Variant=w3537, name=w3534, value=w3533, error in=w3535) -> (Variant out=w3536:variant, error out=w3532:errorcluster)  [unwired: 1 out]
          }
        }
      }
      frame "Phasor Calibration:Backup Calibration Type" {
        n709 = case shown="True" w3547 {
          tunnel: w3546 -> [w3555 w3559]
          tunnel: w3545 -> [w3554 w3562]
          tunnel: [w3553 w3561] -> w3544
          tunnel: w3543 -> [w3552 w3560]
          tunnel: [w3551 w3557] -> w3542
          tunnel: "Backup Calibration Type" -> [w3550 w3563]
          tunnel: [w3548 w3556] -> w3541
          tunnel: w3540 -> [_ w3556]
          frame False {
            n710 = Get Variant Attribute(Variant=w3554, name=w3555, default value (empty Variant)=w3550, error in=w3552) -> (duplicate Variant=w3553:variant, value=w3549:T65, error out=w3551:errorcluster)  [unwired: 1 out]
            n711 = To Variant(anything=w3549) -> (Variant=w3548:variant)
          }
          frame True {
            n712 = Variant To Data(type=w3563, Variant=w3556) -> (data=w3558:T65)  [unwired: 1 in, 1 out]
            n713 = Set Variant Attribute(Variant=w3562, name=w3559, value=w3558, error in=w3560) -> (Variant out=w3561:variant, error out=w3557:errorcluster)  [unwired: 1 out]
          }
        }
      }
      frame "Phasor Calibration:Calibration Type" {
        n714 = case shown="True" w3572 {
          tunnel: w3571 -> [w3580 w3584]
          tunnel: w3570 -> [w3579 w3587]
          tunnel: [w3578 w3586] -> w3569
          tunnel: w3568 -> [w3577 w3585]
          tunnel: [w3576 w3582] -> w3567
          tunnel: "Calibration Type" -> [w3575 w3588]
          tunnel: [w3573 w3581] -> w3566
          tunnel: w3565 -> [_ w3581]
          frame False {
            n715 = Get Variant Attribute(Variant=w3579, name=w3580, default value (empty Variant)=w3575, error in=w3577) -> (duplicate Variant=w3578:variant, value=w3574:T64, error out=w3576:errorcluster)  [unwired: 1 out]
            n716 = To Variant(anything=w3574) -> (Variant=w3573:variant)
          }
          frame True {
            n717 = Variant To Data(type=w3588, Variant=w3581) -> (data=w3583:T64)  [unwired: 1 in, 1 out]
            n718 = Set Variant Attribute(Variant=w3587, name=w3584, value=w3583, error in=w3585) -> (Variant out=w3586:variant, error out=w3582:errorcluster)  [unwired: 1 out]
          }
        }
      }
      frame "Phasor Calibration:Calibration Lifetime" {
        n719 = case shown="True" w3597 {
          tunnel: w3596 -> [w3605 w3609]
          tunnel: w3595 -> [w3604 w3612]
          tunnel: [w3603 w3611] -> w3594
          tunnel: w3593 -> [w3602 w3610]
          tunnel: [w3601 w3607] -> w3592
          tunnel: "Calibration Lifetime" -> [w3600 w3613]
          tunnel: [w3598 w3606] -> w3591
          tunnel: w3590 -> [_ w3606]
          frame False {
            n720 = Get Variant Attribute(Variant=w3604, name=w3605, default value (empty Variant)=w3600, error in=w3602) -> (duplicate Variant=w3603:variant, value=w3599:dbl[unit], error out=w3601:errorcluster)  [unwired: 1 out]
            n721 = To Variant(anything=w3599) -> (Variant=w3598:variant)
          }
          frame True {
            n722 = Variant To Data(type=w3613, Variant=w3606) -> (data=w3608:dbl[unit])  [unwired: 1 in, 1 out]
            n723 = Set Variant Attribute(Variant=w3612, name=w3609, value=w3608, error in=w3610) -> (Variant out=w3611:variant, error out=w3607:errorcluster)  [unwired: 1 out]
          }
        }
      }
      frame "Phasor Calibration:Calibration Map Algorithm" {
        n724 = case shown="True" w3622 {
          tunnel: w3621 -> [w3630 w3634]
          tunnel: w3620 -> [w3629 w3637]
          tunnel: [w3628 w3636] -> w3619
          tunnel: w3618 -> [w3627 w3635]
          tunnel: [w3626 w3632] -> w3617
          tunnel: "Calibration Map Algorithm" -> [w3625 w3638]
          tunnel: [w3623 w3631] -> w3616
          tunnel: w3615 -> [_ w3631]
          frame False {
            n725 = Get Variant Attribute(Variant=w3629, name=w3630, default value (empty Variant)=w3625, error in=w3627) -> (duplicate Variant=w3628:variant, value=w3624:T63, error out=w3626:errorcluster)  [unwired: 1 out]
            n726 = To Variant(anything=w3624) -> (Variant=w3623:variant)
          }
          frame True {
            n727 = Variant To Data(type=w3638, Variant=w3631) -> (data=w3633:T63)  [unwired: 1 in, 1 out]
            n728 = Set Variant Attribute(Variant=w3637, name=w3634, value=w3633, error in=w3635) -> (Variant out=w3636:variant, error out=w3632:errorcluster)  [unwired: 1 out]
          }
        }
      }
      frame "Single-Exponential Phasor Locus (SEPL):Gate Parameters" {
        n729 = case shown="True" w3647 {
          tunnel: w3646 -> [w3655 w3659]
          tunnel: w3645 -> [w3654 w3662]
          tunnel: [w3653 w3661] -> w3644
          tunnel: w3643 -> [w3652 w3660]
          tunnel: [w3651 w3657] -> w3642
          tunnel: "SEPL Gate Parameters" -> [w3650 w3663]
          tunnel: [w3648 w3656] -> w3641
          tunnel: w3640 -> [_ w3656]
          frame False {
            n730 = Get Variant Attribute(Variant=w3654, name=w3655, default value (empty Variant)=w3650, error in=w3652) -> (duplicate Variant=w3653:variant, value=w3649:T60, error out=w3651:errorcluster)  [unwired: 1 out]
            n731 = To Variant(anything=w3649) -> (Variant=w3648:variant)
          }
          frame True {
            n732 = Variant To Data(type=w3663, Variant=w3656) -> (data=w3658:T60)  [unwired: 1 in, 1 out]
            n733 = Set Variant Attribute(Variant=w3662, name=w3659, value=w3658, error in=w3660) -> (Variant out=w3661:variant, error out=w3657:errorcluster)  [unwired: 1 out]
          }
        }
      }
      frame "Single-Exponential Phasor Locus (SEPL):User-defined Gate" {
        n734 = case shown="True" w3672 {
          tunnel: w3671 -> [w3680 w3685]
          tunnel: w3670 -> [w3679 w3688]
          tunnel: [w3678 w3687] -> w3669
          tunnel: w3668 -> [w3677 w3686]
          tunnel: [w3676 w3684] -> w3667
          tunnel: T72 {"X Array"=[], "Y Array"=[]} ("Plot") -> [w3675 w3682]
          tunnel: [w3673 w3683] -> w3666
          tunnel: w3665 -> [_ w3683]
          frame False {
            n735 = Get Variant Attribute(Variant=w3679, name=w3680, default value (empty Variant)=w3675, error in=w3677) -> (duplicate Variant=w3678:variant, value=w3674:T72, error out=w3676:errorcluster)  [unwired: 1 out]
            n736 = To Variant(anything=w3674) -> (Variant=w3673:variant)
          }
          frame True {
            n737 = Variant To Data(type=w3682, Variant=w3683) -> (data=w3681:T72)  [unwired: 1 in, 1 out]
            n738 = global write "Phasor User-defined Gate & IRF.vi" "User-defined Gate"(w3681) -> ()
            n739 = Set Variant Attribute(Variant=w3688, name=w3685, value=w3681, error in=w3686) -> (Variant out=w3687:variant, error out=w3684:errorcluster)  [unwired: 1 out]
          }
        }
      }
      frame "Single-Exponential Phasor Locus (SEPL):User-defined IRF" {
        n740 = case shown="True" w3697 {
          tunnel: w3696 -> [w3705 w3710]
          tunnel: w3695 -> [w3704 w3713]
          tunnel: [w3703 w3712] -> w3694
          tunnel: w3693 -> [w3702 w3711]
          tunnel: [w3701 w3709] -> w3692
          tunnel: T72 {"X Array"=[], "Y Array"=[]} ("Plot") -> [w3700 w3707]
          tunnel: [w3698 w3708] -> w3691
          tunnel: w3690 -> [_ w3708]
          frame False {
            n741 = Get Variant Attribute(Variant=w3704, name=w3705, default value (empty Variant)=w3700, error in=w3702) -> (duplicate Variant=w3703:variant, value=w3699:T72, error out=w3701:errorcluster)  [unwired: 1 out]
            n742 = To Variant(anything=w3699) -> (Variant=w3698:variant)
          }
          frame True {
            n743 = Variant To Data(type=w3707, Variant=w3708) -> (data=w3706:T72)  [unwired: 1 in, 1 out]
            n744 = global write "Phasor User-defined Gate & IRF.vi" "User-defined IRF"(w3706) -> ()
            n745 = Set Variant Attribute(Variant=w3713, name=w3710, value=w3706, error in=w3711) -> (Variant out=w3712:variant, error out=w3709:errorcluster)  [unwired: 1 out]
          }
        }
      }
      frame "Single-Exponential Phasor Locus (SEPL):Phasor Parameters" {
        n746 = case shown="True" w3722 {
          tunnel: w3721 -> [w3730 w3734]
          tunnel: w3720 -> [w3729 w3737]
          tunnel: [w3728 w3736] -> w3719
          tunnel: w3718 -> [w3727 w3735]
          tunnel: [w3726 w3732] -> w3717
          tunnel: "SEPL Phasor Parameters" -> [w3725 w3738]
          tunnel: [w3723 w3731] -> w3716
          tunnel: w3715 -> [_ w3731]
          frame False {
            n747 = Get Variant Attribute(Variant=w3729, name=w3730, default value (empty Variant)=w3725, error in=w3727) -> (duplicate Variant=w3728:variant, value=w3724:T55, error out=w3726:errorcluster)  [unwired: 1 out]
            n748 = To Variant(anything=w3724) -> (Variant=w3723:variant)
          }
          frame True {
            n749 = Variant To Data(type=w3738, Variant=w3731) -> (data=w3733:T55)  [unwired: 1 in, 1 out]
            n750 = Set Variant Attribute(Variant=w3737, name=w3734, value=w3733, error in=w3735) -> (Variant out=w3736:variant, error out=w3732:errorcluster)  [unwired: 1 out]
          }
        }
      }
      frame "Single-Exponential Phasor Locus (SEPL):Decay & IRF Parameters" {
        n751 = case shown="True" w3747 {
          tunnel: w3746 -> [w3755 w3759]
          tunnel: w3745 -> [w3754 w3762]
          tunnel: [w3753 w3761] -> w3744
          tunnel: w3743 -> [w3752 w3760]
          tunnel: [w3751 w3757] -> w3742
          tunnel: "SEPL IRF Parameters" -> [w3750 w3763]
          tunnel: [w3748 w3756] -> w3741
          tunnel: w3740 -> [_ w3756]
          frame False {
            n752 = Get Variant Attribute(Variant=w3754, name=w3755, default value (empty Variant)=w3750, error in=w3752) -> (duplicate Variant=w3753:variant, value=w3749:T58, error out=w3751:errorcluster)  [unwired: 1 out]
            n753 = To Variant(anything=w3749) -> (Variant=w3748:variant)
          }
          frame True {
            n754 = Variant To Data(type=w3763, Variant=w3756) -> (data=w3758:T58)  [unwired: 1 in, 1 out]
            n755 = Set Variant Attribute(Variant=w3762, name=w3759, value=w3758, error in=w3760) -> (Variant out=w3761:variant, error out=w3757:errorcluster)  [unwired: 1 out]
          }
        }
      }
      frame "Single-Exponential Phasor Locus (SEPL):Display Parameters" {
        n756 = case shown="True" w3772 {
          tunnel: w3771 -> [w3780 w3784]
          tunnel: w3770 -> [w3779 w3787]
          tunnel: [w3778 w3786] -> w3769
          tunnel: w3768 -> [w3777 w3785]
          tunnel: [w3776 w3782] -> w3767
          tunnel: "SEPL Display Parameters" -> [w3775 w3788]
          tunnel: [w3773 w3781] -> w3766
          tunnel: w3765 -> [_ w3781]
          frame False {
            n757 = Get Variant Attribute(Variant=w3779, name=w3780, default value (empty Variant)=w3775, error in=w3777) -> (duplicate Variant=w3778:variant, value=w3774:T53, error out=w3776:errorcluster)  [unwired: 1 out]
            n758 = To Variant(anything=w3774) -> (Variant=w3773:variant)
          }
          frame True {
            n759 = Variant To Data(type=w3788, Variant=w3781) -> (data=w3783:T53)  [unwired: 1 in, 1 out]
            n760 = Set Variant Attribute(Variant=w3787, name=w3784, value=w3783, error in=w3785) -> (Variant out=w3786:variant, error out=w3782:errorcluster)  [unwired: 1 out]
          }
        }
      }
      frame "Lifetime Analysis:Decay Analysis Parameters" {
        n761 = case shown="True" w3797 {
          tunnel: w3796 -> [w3805 w3809]
          tunnel: w3795 -> [w3804 w3812]
          tunnel: [w3803 w3811] -> w3794
          tunnel: w3793 -> [w3802 w3810]
          tunnel: [w3801 w3807] -> w3792
          tunnel: "Decay Analysis Parameters" -> [w3800 w3813]
          tunnel: [w3798 w3806] -> w3791
          tunnel: w3790 -> [_ w3806]
          frame False {
            n762 = Get Variant Attribute(Variant=w3804, name=w3805, default value (empty Variant)=w3800, error in=w3802) -> (duplicate Variant=w3803:variant, value=w3799:T20, error out=w3801:errorcluster)  [unwired: 1 out]
            n763 = To Variant(anything=w3799) -> (Variant=w3798:variant)
          }
          frame True {
            n764 = Variant To Data(type=w3813, Variant=w3806) -> (data=w3808:T20)  [unwired: 1 in, 1 out]
            n765 = Set Variant Attribute(Variant=w3812, name=w3809, value=w3808, error in=w3810) -> (Variant out=w3811:variant, error out=w3807:errorcluster)  [unwired: 1 out]
          }
        }
      }
      frame "Lifetime Analysis:Lifetime Map Active" {
        w3814 = FALSE  # Not a Settings Window Control
        n766 = case shown="True" w3822 {
          tunnel: w3821 -> [w3830 w3834]
          tunnel: w3820 -> [w3829 w3837]
          tunnel: [w3828 w3836] -> w3819
          tunnel: w3818 -> [w3827 w3835]
          tunnel: [w3826 w3832] -> w3817
          tunnel: w3814 -> [w3825 w3838]
          tunnel: [w3823 w3831] -> w3816
          tunnel: w3815 -> [_ w3831]
          frame False {
            n767 = Get Variant Attribute(Variant=w3829, name=w3830, default value (empty Variant)=w3825, error in=w3827) -> (duplicate Variant=w3828:variant, value=w3824:bool, error out=w3826:errorcluster)  [unwired: 1 out]
            n768 = To Variant(anything=w3824) -> (Variant=w3823:variant)
          }
          frame True {
            n769 = Variant To Data(type=w3838, Variant=w3831) -> (data=w3833:bool)  [unwired: 1 in, 1 out]
            n770 = Set Variant Attribute(Variant=w3837, name=w3834, value=w3833, error in=w3835) -> (Variant out=w3836:variant, error out=w3832:errorcluster)  [unwired: 1 out]
          }
        }
      }
      frame "Plugins:Python Settings" {
        n771 = case shown="False" w3847 {
          tunnel: w3846 -> [w3855 w3859]
          tunnel: w3845 -> [w3854 w3862]
          tunnel: [w3853 w3861] -> w3844
          tunnel: w3843 -> [w3852 w3860]
          tunnel: [w3851 w3857] -> w3842
          tunnel: "Python Settings" -> [w3850 w3863]
          tunnel: [w3848 w3856] -> w3841
          tunnel: w3840 -> [_ w3856]
          frame False {
            n772 = Get Variant Attribute(Variant=w3854, name=w3855, default value (empty Variant)=w3850, error in=w3852) -> (duplicate Variant=w3853:variant, value=w3849:T66, error out=w3851:errorcluster)  [unwired: 1 out]
            n773 = To Variant(anything=w3849) -> (Variant=w3848:variant)
          }
          frame True {
            n774 = Variant To Data(type=w3863, Variant=w3856) -> (data=w3858:T66)  [unwired: 1 in, 1 out]
            n775 = Set Variant Attribute(Variant=w3862, name=w3859, value=w3858, error in=w3860) -> (Variant out=w3861:variant, error out=w3857:errorcluster)  [unwired: 1 out]
          }
        }
      }
      frame "Miscellaneous:Verbose Mode" {
        n776 = case shown="True" w3872 {
          tunnel: w3871 -> [w3880 w3885]
          tunnel: w3870 -> [w3879 w3888]
          tunnel: [w3878 w3887] -> w3869
          tunnel: w3868 -> [w3877 w3886]
          tunnel: [w3876 w3884] -> w3867
          tunnel: "Verbose Mode" -> [w3875 w3882]
          tunnel: [w3873 w3883] -> w3866
          tunnel: w3865 -> [_ w3883]
          frame False {
            n777 = Get Variant Attribute(Variant=w3879, name=w3880, default value (empty Variant)=w3875, error in=w3877) -> (duplicate Variant=w3878:variant, value=w3874:bool, error out=w3876:errorcluster)  [unwired: 1 out]
            n778 = To Variant(anything=w3874) -> (Variant=w3873:variant)
          }
          frame True {
            n779 = Variant To Data(type=w3882, Variant=w3883) -> (data=w3881:bool)  [unwired: 1 in, 1 out]
            n780 = global write "Verbose Mode.vi" "Verbose Mode"(w3881) -> ()
            n781 = Set Variant Attribute(Variant=w3888, name=w3885, value=w3881, error in=w3886) -> (Variant out=w3887:variant, error out=w3884:errorcluster)  [unwired: 1 out]
          }
        }
      }
      frame "Miscellaneous:Beep after Script" {
        n782 = case shown="True" w3897 {
          tunnel: w3896 -> [w3905 w3909]
          tunnel: w3895 -> [w3904 w3912]
          tunnel: [w3903 w3911] -> w3894
          tunnel: w3893 -> [w3902 w3910]
          tunnel: [w3901 w3907] -> w3892
          tunnel: "Beep after Script" -> [w3900 w3913]
          tunnel: [w3898 w3906] -> w3891
          tunnel: w3890 -> [_ w3906]
          frame False {
            n783 = Get Variant Attribute(Variant=w3904, name=w3905, default value (empty Variant)=w3900, error in=w3902) -> (duplicate Variant=w3903:variant, value=w3899:bool, error out=w3901:errorcluster)  [unwired: 1 out]
            n784 = To Variant(anything=w3899) -> (Variant=w3898:variant)
          }
          frame True {
            n785 = Variant To Data(type=w3913, Variant=w3906) -> (data=w3908:bool)  [unwired: 1 in, 1 out]
            n786 = Set Variant Attribute(Variant=w3912, name=w3909, value=w3908, error in=w3910) -> (Variant out=w3911:variant, error out=w3907:errorcluster)  [unwired: 1 out]
          }
        }
      }
      frame "Miscellaneous:Saved Image File Format" {
        n787 = case shown="False" w3922 {
          tunnel: w3921 -> [w3930 w3934]
          tunnel: w3920 -> [w3929 w3937]
          tunnel: [w3928 w3936] -> w3919
          tunnel: w3918 -> [w3927 w3935]
          tunnel: [w3926 w3932] -> w3917
          tunnel: "Saved Displayed Image File Format" -> [w3925 w3938]
          tunnel: [w3923 w3931] -> w3916
          tunnel: w3915 -> [_ w3931]
          frame False {
            n788 = Get Variant Attribute(Variant=w3929, name=w3930, default value (empty Variant)=w3925, error in=w3927) -> (duplicate Variant=w3928:variant, value=w3924:T71, error out=w3926:errorcluster)  [unwired: 1 out]
            n789 = To Variant(anything=w3924) -> (Variant=w3923:variant)
          }
          frame True {
            n790 = Variant To Data(type=w3938, Variant=w3931) -> (data=w3933:T71)  [unwired: 1 in, 1 out]
            n791 = Set Variant Attribute(Variant=w3937, name=w3934, value=w3933, error in=w3935) -> (Variant out=w3936:variant, error out=w3932:errorcluster)  [unwired: 1 out]
          }
        }
      }
      frame "Miscellaneous:Exported Gate Image Settings" {
        n792 = case shown="False" w3947 {
          tunnel: w3946 -> [w3955 w3959]
          tunnel: w3945 -> [w3954 w3962]
          tunnel: [w3953 w3961] -> w3944
          tunnel: w3943 -> [w3952 w3960]
          tunnel: [w3951 w3957] -> w3942
          tunnel: "Exported Gate Image Settings" -> [w3950 w3963]
          tunnel: [w3948 w3956] -> w3941
          tunnel: w3940 -> [_ w3956]
          frame False {
            n793 = Get Variant Attribute(Variant=w3954, name=w3955, default value (empty Variant)=w3950, error in=w3952) -> (duplicate Variant=w3953:variant, value=w3949:T70, error out=w3951:errorcluster)  [unwired: 1 out]
            n794 = To Variant(anything=w3949) -> (Variant=w3948:variant)
          }
          frame True {
            n795 = Variant To Data(type=w3963, Variant=w3956) -> (data=w3958:T70)  [unwired: 1 in, 1 out]
            n796 = Set Variant Attribute(Variant=w3962, name=w3959, value=w3958, error in=w3960) -> (Variant out=w3961:variant, error out=w3957:errorcluster)  [unwired: 1 out]
          }
        }
      }
      frame "Miscellaneous:Include Loading in Timing" {
        n797 = case shown="True" w3972 {
          tunnel: w3971 -> [w3980 w3984]
          tunnel: w3970 -> [w3979 w3987]
          tunnel: [w3978 w3986] -> w3969
          tunnel: w3968 -> [w3977 w3985]
          tunnel: [w3976 w3982] -> w3967
          tunnel: "Include Loading in Timing" -> [w3975 w3988]
          tunnel: [w3973 w3981] -> w3966
          tunnel: w3965 -> [_ w3981]
          frame False {
            n798 = Get Variant Attribute(Variant=w3979, name=w3980, default value (empty Variant)=w3975, error in=w3977) -> (duplicate Variant=w3978:variant, value=w3974:bool, error out=w3976:errorcluster)  [unwired: 1 out]
            n799 = To Variant(anything=w3974) -> (Variant=w3973:variant)
          }
          frame True {
            n800 = Variant To Data(type=w3988, Variant=w3981) -> (data=w3983:bool)  [unwired: 1 in, 1 out]
            n801 = Set Variant Attribute(Variant=w3987, name=w3984, value=w3983, error in=w3985) -> (Variant out=w3986:variant, error out=w3982:errorcluster)  [unwired: 1 out]
          }
        }
      }
      frame "Miscellaneous:Verbose Settings Mode" {
        n802 = case shown="False" w3997 {
          tunnel: w3996 -> [w4005 w4009]
          tunnel: w3995 -> [w4004 w4012]
          tunnel: [w4003 w4011] -> w3994
          tunnel: w3993 -> [w4002 w4010]
          tunnel: [w4001 w4007] -> w3992
          tunnel: "Verbose Settings Mode" -> [w4000 w4013]
          tunnel: [w3998 w4006] -> w3991
          tunnel: w3990 -> [_ w4006]
          frame False {
            n803 = Get Variant Attribute(Variant=w4004, name=w4005, default value (empty Variant)=w4000, error in=w4002) -> (duplicate Variant=w4003:variant, value=w3999:bool, error out=w4001:errorcluster)  [unwired: 1 out]
            n804 = To Variant(anything=w3999) -> (Variant=w3998:variant)
          }
          frame True {
            n805 = Variant To Data(type=w4013, Variant=w4006) -> (data=w4008:bool)  [unwired: 1 in, 1 out]
            n806 = Set Variant Attribute(Variant=w4012, name=w4009, value=w4008, error in=w4010) -> (Variant out=w4011:variant, error out=w4007:errorcluster)  [unwired: 1 out]
          }
        }
      }
      frame "Miscellaneous:Histogram Options" {
        n807 = case shown="False" w4022 {
          tunnel: w4021 -> [w4030 w4034]
          tunnel: w4020 -> [w4029 w4037]
          tunnel: [w4028 w4036] -> w4019
          tunnel: w4018 -> [w4027 w4035]
          tunnel: [w4026 w4032] -> w4017
          tunnel: "Histogram Options" -> [w4025 w4038]
          tunnel: [w4023 w4031] -> w4016
          tunnel: w4015 -> [_ w4031]
          frame False {
            n808 = Get Variant Attribute(Variant=w4029, name=w4030, default value (empty Variant)=w4025, error in=w4027) -> (duplicate Variant=w4028:variant, value=w4024:T67, error out=w4026:errorcluster)  [unwired: 1 out]
            n809 = To Variant(anything=w4024) -> (Variant=w4023:variant)
          }
          frame True {
            n810 = Variant To Data(type=w4038, Variant=w4031) -> (data=w4033:T67)  [unwired: 1 in, 1 out]
            n811 = Set Variant Attribute(Variant=w4037, name=w4034, value=w4033, error in=w4035) -> (Variant out=w4036:variant, error out=w4032:errorcluster)  [unwired: 1 out]
          }
        }
      }
      frame "Miscellaneous:Beep on Error" {
        n812 = case shown="False" w4047 {
          tunnel: w4046 -> [w4055 w4059]
          tunnel: w4045 -> [w4054 w4062]
          tunnel: [w4053 w4061] -> w4044
          tunnel: w4043 -> [w4052 w4060]
          tunnel: [w4051 w4057] -> w4042
          tunnel: "Beep on Error" -> [w4050 w4063]
          tunnel: [w4048 w4056] -> w4041
          tunnel: w4040 -> [_ w4056]
          frame False {
            n813 = Get Variant Attribute(Variant=w4054, name=w4055, default value (empty Variant)=w4050, error in=w4052) -> (duplicate Variant=w4053:variant, value=w4049:bool, error out=w4051:errorcluster)  [unwired: 1 out]
            n814 = To Variant(anything=w4049) -> (Variant=w4048:variant)
          }
          frame True {
            n815 = Variant To Data(type=w4063, Variant=w4056) -> (data=w4058:bool)  [unwired: 1 in, 1 out]
            n816 = Set Variant Attribute(Variant=w4062, name=w4059, value=w4058, error in=w4060) -> (Variant out=w4061:variant, error out=w4057:errorcluster)  [unwired: 1 out]
          }
        }
      }
      frame "Miscellaneous:# Logical Processors Used" {
        n817 = case shown="True" w4072 {
          tunnel: w4071 -> [w4080 w4085]
          tunnel: w4070 -> [w4079 w4088]
          tunnel: [w4078 w4087] -> w4069
          tunnel: w4068 -> [w4077 w4086]
          tunnel: [w4076 w4084] -> w4067
          tunnel: "# Logical Processors Used" -> [w4075 w4089]
          tunnel: [w4073 w4083] -> w4066
          tunnel: w4065 -> [_ w4083]
          frame False {
            n818 = Get Variant Attribute(Variant=w4079, name=w4080, default value (empty Variant)=w4075, error in=w4077) -> (duplicate Variant=w4078:variant, value=w4074:i32, error out=w4076:errorcluster)  [unwired: 1 out]
            n819 = To Variant(anything=w4074) -> (Variant=w4073:variant)
          }
          frame True {
            n820 = Variant To Data(type=w4089, Variant=w4083) -> (data=w4082:i32)  [unwired: 1 in, 1 out]
            n821 = call "Logical Processors Used.vi"("Set/Get (F)"=TRUE, "# Logical Processor Used"=w4082) -> ()  [unwired: 4 in, 1 out]
            n822 = Set Variant Attribute(Variant=w4088, name=w4085, value=w4082, error in=w4086) -> (Variant out=w4087:variant, error out=w4084:errorcluster)  [unwired: 1 out]
          }
        }
      }
      frame "Miscellaneous:ROI Description Max Characters" {
        n823 = case shown="False" w4098 {
          tunnel: w4097 -> [w4106 w4110]
          tunnel: w4096 -> [w4105 w4113]
          tunnel: [w4104 w4112] -> w4095
          tunnel: w4094 -> [w4103 w4111]
          tunnel: [w4102 w4108] -> w4093
          tunnel: "ROI Description Max Characters" -> [w4101 w4114]
          tunnel: [w4099 w4107] -> w4092
          tunnel: w4091 -> [_ w4107]
          frame False {
            n824 = Get Variant Attribute(Variant=w4105, name=w4106, default value (empty Variant)=w4101, error in=w4103) -> (duplicate Variant=w4104:variant, value=w4100:i32, error out=w4102:errorcluster)  [unwired: 1 out]
            n825 = To Variant(anything=w4100) -> (Variant=w4099:variant)
          }
          frame True {
            n826 = Variant To Data(type=w4114, Variant=w4107) -> (data=w4109:i32)  [unwired: 1 in, 1 out]
            n827 = Set Variant Attribute(Variant=w4113, name=w4110, value=w4109, error in=w4111) -> (Variant out=w4112:variant, error out=w4108:errorcluster)  [unwired: 1 out]
          }
        }
      }
      frame "Miscellaneous:Verbose Error Mode" {
        n828 = case shown="True" w4123 {
          tunnel: w4122 -> [w4131 w4136]
          tunnel: w4121 -> [w4130 w4139]
          tunnel: [w4129 w4138] -> w4120
          tunnel: w4119 -> [w4128 w4137]
          tunnel: [w4127 w4134] -> w4118
          tunnel: "Verbose Error Mode" -> [w4126 w4132]
          tunnel: [w4124 w4133] -> w4117
          tunnel: w4116 -> [_ w4133]
          frame False {
            n829 = Get Variant Attribute(Variant=w4130, name=w4131, default value (empty Variant)=w4126, error in=w4128) -> (duplicate Variant=w4129:variant, value=w4125:bool, error out=w4127:errorcluster)  [unwired: 1 out]
            n830 = To Variant(anything=w4125) -> (Variant=w4124:variant)
          }
          frame True {
            n831 = Variant To Data(type=w4132, Variant=w4133) -> (data=w4135:bool)  [unwired: 1 in, 1 out]
            n832 = global write "Verbose Mode.vi" "Verbose Error Mode"(w4132) -> ()
            n833 = Set Variant Attribute(Variant=w4139, name=w4136, value=w4135, error in=w4137) -> (Variant out=w4138:variant, error out=w4134:errorcluster)  [unwired: 1 out]
          }
        }
      }
      frame "Miscellaneous:Transparent Mask Color" {
        n834 = case shown="True" w4148 {
          tunnel: w4147 -> [w4156 w4161]
          tunnel: w4146 -> [w4155 w4164]
          tunnel: [w4154 w4163] -> w4145
          tunnel: w4144 -> [w4153 w4162]
          tunnel: [w4152 w4159] -> w4143
          tunnel: "Transparent Mask Color" -> [w4151 w4157]
          tunnel: [w4149 w4158] -> w4142
          tunnel: w4141 -> [_ w4158]
          frame False {
            n835 = Get Variant Attribute(Variant=w4155, name=w4156, default value (empty Variant)=w4151, error in=w4153) -> (duplicate Variant=w4154:variant, value=w4150:u32, error out=w4152:errorcluster)  [unwired: 1 out]
            n836 = To Variant(anything=w4150) -> (Variant=w4149:variant)
          }
          frame True {
            n837 = Variant To Data(type=w4157, Variant=w4158) -> (data=w4160:u32)  [unwired: 1 in, 1 out]
            n838 = Set Variant Attribute(Variant=w4164, name=w4161, value=w4160, error in=w4162) -> (Variant out=w4163:variant, error out=w4159:errorcluster)  [unwired: 1 out]
          }
        }
      }
    }
  }
  "Error Out" <- w4
  "Variant Data out" <- w3
